vi "BIMS_Collector (SPR).vi"() -> ()   [LabVIEW 2015]
doc: "This program is currently beta software. It is designed to address the data requirements defined primarily by the DHB Ballistic Test Report.\n\nThe general operation of this program is based on the Ballistics Version 2005 application developed internally by DuPont as a research tool for the Spruance Plant Ballistics Lab in Richmond, VA.\n\nPlease note that the original trigger control logic was modified and no longer depends on a safety interlock system to enable operation of a ballistic test.\n\nDuPont makes no warranties and assumes no liabilities in connection with any use of this program."
uses:
  DataSource.ctl
  shotsArr.ctl
  Shot Record.ctl
  Collector State.ctl
  <vilib>/Utility/error.llb/DialogType.ctl
  <vilib>/registry/registry.llb/Registry RtKey.ctl
  <vilib>/DAQmx/read.llb/DAQmx Read (Counter DBL 1Chan 1Samp).vi
  BIMS_Collector Globals.vi
  <vilib>/Utility/config.llb/Write Key (String).vi
  <vilib>/addons/database/Connection.llb/DB Tools Open Connec (Path).vi
  <vilib>/addons/database/Connection.llb/Conn Execute.vi
  <vilib>/addons/database/Recordset.llb/Rec Destroy - Connection.vi
  <vilib>/DAQmx/miscellaneous.llb/DAQmx Fill In Error Info.vi
  <vilib>/addons/database/NI_Database_API.lvlib
  <vilib>/Utility/config.llb/NI_LVConfig.lvlib
  <vilib>/Utility/file.llb/Write To Spreadsheet File (string).vi
panel:
  in  "diagPageVisible":bool
  in  "runtimeMenusVisible":bool=TRUE
  out "loadStatus":string
  out "Loading":u16(ring)
  in  "RESET All":bool
  out "ConfigName":string
  out "TimeNow":string
  in  "EXIT":bool
  in  "mainTabCntrl":enum32{"Setup", "Measure", "History", "System"}(tab)=enum."System"
  in  "SampleEntryTabCntrl":enum32{"Environment", "Sample"}(tab)
  in  "ThreatDetails":u16(ring) caption="Detail"
  in  "ThreatGroups":u16(ring) caption="Group" items=["", "RCC", "FSP", "44 Magnum", "40 S&W", "9mm Luger", "357 Magnum", "357 Sig", "5.56 NATO / 223", "7.62 Win"]
  in  "PowderTypes":u16(ring) caption="Type" items=["", "ACCURATE, NO.2", "ACCURATE, NO.9", "Alliant Herc. Bullseye", "Alliant 2400", "Hercules", "Hi-Skor 700x", "Hi-Skor 800x", "IMR-4198", "IMR-4756", "IMR-4895", "Power Pistol", "Winchester Ball", "WINCHESTER-231", "WINCHESTER-296", "OTHER"]
  in  "Ballisticians":u16(ring) caption="Ballistician" items=["", "Luke Jeter", "Eric Key", "Luke Jeter - Eric Key"]
  in  "Recorders":u16(ring) caption="Recorder"
  in  "Shooters":u16(ring) caption="Shooter"
  in  "Methods":u16(ring) caption="Method" items=["", "V50", "NIJ", "V0", "Custom"]
  in  "RoomT":sgl caption="Temperature (° F)" format="%.1f"
  in  "RoomHum":sgl caption="Humidity (%)" min=0 max=100 format="%.1f"
  in  "SampleBackings":u16(ring)=3 caption="Type" items=["", "Clay", "Aluminum", "Air"]
  in  "clayCalArray":i16[](array[numeric])=[0, 0, 0, 0, 0] caption="Calibration (mm)" min=0 max=99 format="%02.0f"
  out "clayAverage":sgl caption="Clay Average (mm)" format="%#.1f"
  in  "clayTemp":sgl caption="Clay Temp (° F)" format="%.1f"
  out "threatDetails":T1 caption="Description"
  in  "SampleClamping":u16(ring) caption="Clamping" items=["", "None", "12 x 12", "12 x 15", "15 x 15 Flat", "15 x 15 Teeth", "16 x 16 Flat", "16 x 16 Teeth", "18 x 18", "20 x 20", "Hydro Pneumatic"]
  in  "Sample SubTabCntrl":T2(tab)
  in  "SampleID":string caption="Sample ID"
  in  "SampleDimensions":u16(ring) caption="Dimensions" items=["", "15 x 15", "12 x 12", "10.25 x 11.75", "15 x 16", "26 x 26", "8.5 x 11", "12 x 15", "16 x 16", "18 x 18", "20 x 16", "15 x 18", "24 x 24", "13 x 13", "7.5 x 7.5", "VEST PANEL", "CHEST PLATE", "HELMET", "NOT APPLICABLE", "ACH", "PASGT"]
  in  "ModelMfrs":u16(ring) caption="Manufacturer" items=["DuPont Experimental", "Clark Schwebel", "Industriales Textiles", "Maydown", "Second Chance Body Armor", "Point Blank-Marine Interceptor", "Safari Land", "American Body Armor", "Europe", "Force One", "Textile Filter", "Hexcel Schwebel", "BGF", "M.C. GILL", "COLUMBIA", "Britax HEATH TECN", "ARLON", "TEX TECH INC.", "TELAIR", "CADDIN BODY ARMOR", "GEPCO", "3 TEX", "PACA BODY ARMOR", "VON ROL ISOLA", "SIOUX MANUFACTURING", "APEJ-TAIWAN", "FLOPPY BODY ARMOR", "UNICOR", "n/a", "Point Blank", "Diamond Back", "Other"]
  in  "SampleTypes":u16(ring) caption="Sample Type" items=["", "Fabric", "Hard", "Helmet", "Vest", "Paper"]
  in  "Submitters":u16(ring) caption="Submitter" items=["", "Aldo Tavarez", "James Singletary", "Jeff Hanks", "Karl Chang", "Minshon Chiou", "Ron Egres", "Bryce VanArsdalen", "Kevin Mulcahy", "Dave Reichert", "Leo Carbajal"]
  in  "ProjectID":string caption="Project ID"
  in  "BackLayers":i32 caption="# of Layers" min=0 max=99 step=5
  in  "FrontLayers":i32 caption="# of Layers" min=0 max=99 step=5
  in  "BackLayer":u16(ring) caption="Back Layer" items=["", "n/a", "CORDURA 500d"]
  in  "FrontLayer":u16(ring) caption="Front Layer" items=["", "n/a", "CORDURA 1000d"]
  out "totalNumLayers":i32 caption="Total # of Layers" min=0 max=100 step=5
  out "totalBAW":sgl caption="Total BAW (psf)" format="%.2f"
  in  "LayerTabControl":enum32{"1", "2", "3", "4", "5", "6"}(tab) caption="Inner Layers"
  out "fab1_totalWt":sgl caption="Fab1 Wt" min=0 max=99 step=5 format="%.2f"
  out "SampleAttribs_1":T3 caption="fabricAttribs_1"
  in  "Layer_1":T4 caption="Fabric #1" {"plyNum" min=0 max=99 step=5}
  in  "SampleStyle_1":u16(ring)
  in  "Mfr_1":u16(ring) caption="vendor" items=["", "3M", "A&P Technology", "Absecon Mills", "ABT Sciences", "Aermet", "ArmorStruxx", "Artec", "Axiom", "BAE Advanced Ceramics", "Barrday", "BGF", "Citterio", "Coors-Tek", "DSM", "DuPont", "DuPont (JPS-SUBC)", "FTC", "Gentex", "Gurit", "Hexcel", "Honeywell", "JD Lincoln", "JPS", "JPS-Alexium", "JPS-Apjet", "JPS-DuPont", "JPS-Huntsman", "JPS-Old Hickory", "JPS-TSG", "Kamenskvolokno", "Lincoln Fabrics", "Loctite", "Lord", "LTC", "Marcus Materials", "McMaster-Carr", "Nanocomp", "Neva", "Nolax", "OConnell", "Patriot 3", "PATZ", "PBO", "Polystrand", "Pro-Systems", "ProTech", "Rusar", "Saati", "Saint Gobain", "S-Bond", "SEAL", "Sioux", "SPDW", "TechFiber", "Teijin", "Tencate", "Tensylon", "TexTech", "Toray", "TWARON", "UNKNOWN", "VonWeiss", "Xymid", "Z11"]
  in  "layerStitch_1":u16(ring) caption="Stitch" items=["", "1-inch quilt", "2-inch quilt", "Corner Bartack", "Corners", "Custom (Panel)", "Custom (Vest)", "Diamond", "Edge", "n/a", "Normal"]
  out "fab2_totalWt":sgl caption="Fab2 Wt" min=0 max=99 step=5 format="%.2f"
  out "SampleAttribs_2":T3 caption="fabricAttribs_2"
  in  "Layer_2":T4 caption="Fabric #2" {"plyNum" min=0 max=99 step=5}
  in  "SampleStyle_2":u16(ring)
  in  "Mfr_2":u16(ring) caption="vendor" items=["", "3M", "A&P Technology", "Absecon Mills", "ABT Sciences", "Aermet", "ArmorStruxx", "Artec", "Axiom", "BAE Advanced Ceramics", "Barrday", "BGF", "Citterio", "Coors-Tek", "DSM", "DuPont", "DuPont (JPS-SUBC)", "FTC", "Gentex", "Gurit", "Hexcel", "Honeywell", "JD Lincoln", "JPS", "JPS-Alexium", "JPS-Apjet", "JPS-DuPont", "JPS-Huntsman", "JPS-Old Hickory", "JPS-TSG", "Kamenskvolokno", "Lincoln Fabrics", "Loctite", "Lord", "LTC", "Marcus Materials", "McMaster-Carr", "Nanocomp", "Neva", "Nolax", "OConnell", "Patriot 3", "PATZ", "PBO", "Polystrand", "Pro-Systems", "ProTech", "Rusar", "Saati", "Saint Gobain", "S-Bond", "SEAL", "Sioux", "SPDW", "TechFiber", "Teijin", "Tencate", "Tensylon", "TexTech", "Toray", "TWARON", "UNKNOWN", "VonWeiss", "Xymid", "Z11"]
  in  "layerStitch_2":u16(ring) caption="Stitch" items=["", "1-inch quilt", "2-inch quilt", "Corner Bartack", "Corners", "Custom (Panel)", "Custom (Vest)", "Diamond", "Edge", "n/a", "Normal"]
  out "fab3_totalWt":sgl caption="Fab3 Wt" min=0 max=99 step=5 format="%.2f"
  out "SampleAttribs_3":T3 caption="fabricAttribs_3"
  in  "Layer_3":T4 caption="Fabric #3" {"plyNum" min=0 max=99 step=5}
  in  "SampleStyle_3":u16(ring)
  in  "Mfr_3":u16(ring) caption="vendor" items=["", "3M", "A&P Technology", "Absecon Mills", "ABT Sciences", "Aermet", "ArmorStruxx", "Artec", "Axiom", "BAE Advanced Ceramics", "Barrday", "BGF", "Citterio", "Coors-Tek", "DSM", "DuPont", "DuPont (JPS-SUBC)", "FTC", "Gentex", "Gurit", "Hexcel", "Honeywell", "JD Lincoln", "JPS", "JPS-Alexium", "JPS-Apjet", "JPS-DuPont", "JPS-Huntsman", "JPS-Old Hickory", "JPS-TSG", "Kamenskvolokno", "Lincoln Fabrics", "Loctite", "Lord", "LTC", "Marcus Materials", "McMaster-Carr", "Nanocomp", "Neva", "Nolax", "OConnell", "Patriot 3", "PATZ", "PBO", "Polystrand", "Pro-Systems", "ProTech", "Rusar", "Saati", "Saint Gobain", "S-Bond", "SEAL", "Sioux", "SPDW", "TechFiber", "Teijin", "Tencate", "Tensylon", "TexTech", "Toray", "TWARON", "UNKNOWN", "VonWeiss", "Xymid", "Z11"]
  in  "layerStitch_3":u16(ring) caption="Stitch" items=["", "1-inch quilt", "2-inch quilt", "Corner Bartack", "Corners", "Custom (Panel)", "Custom (Vest)", "Diamond", "Edge", "n/a", "Normal"]
  out "fab4_totalWt":sgl caption="Fab4 Wt" min=0 max=99 step=5 format="%.2f"
  out "SampleAttribs_4":T3 caption="fabricAttribs_4"
  in  "Layer_4":T4 caption="Fabric #4" {"plyNum" min=0 max=99 step=5}
  in  "SampleStyle_4":u16(ring)
  in  "Mfr_4":u16(ring) caption="vendor" items=["", "3M", "A&P Technology", "Absecon Mills", "ABT Sciences", "Aermet", "ArmorStruxx", "Artec", "Axiom", "BAE Advanced Ceramics", "Barrday", "BGF", "Citterio", "Coors-Tek", "DSM", "DuPont", "DuPont (JPS-SUBC)", "FTC", "Gentex", "Gurit", "Hexcel", "Honeywell", "JD Lincoln", "JPS", "JPS-Alexium", "JPS-Apjet", "JPS-DuPont", "JPS-Huntsman", "JPS-Old Hickory", "JPS-TSG", "Kamenskvolokno", "Lincoln Fabrics", "Loctite", "Lord", "LTC", "Marcus Materials", "McMaster-Carr", "Nanocomp", "Neva", "Nolax", "OConnell", "Patriot 3", "PATZ", "PBO", "Polystrand", "Pro-Systems", "ProTech", "Rusar", "Saati", "Saint Gobain", "S-Bond", "SEAL", "Sioux", "SPDW", "TechFiber", "Teijin", "Tencate", "Tensylon", "TexTech", "Toray", "TWARON", "UNKNOWN", "VonWeiss", "Xymid", "Z11"]
  in  "layerStitch_4":u16(ring) caption="Stitch" items=["", "1-inch quilt", "2-inch quilt", "Corner Bartack", "Corners", "Custom (Panel)", "Custom (Vest)", "Diamond", "Edge", "n/a", "Normal"]
  out "fab5_totalWt":sgl caption="Fab5 Wt" min=0 max=99 step=5 format="%.2f"
  out "SampleAttribs_5":T3 caption="fabricAttribs_5"
  in  "Layer_5":T4 caption="Fabric #5" {"plyNum" min=0 max=99 step=5}
  in  "SampleStyle_5":u16(ring)
  in  "Mfr_5":u16(ring) caption="vendor" items=["", "3M", "A&P Technology", "Absecon Mills", "ABT Sciences", "Aermet", "ArmorStruxx", "Artec", "Axiom", "BAE Advanced Ceramics", "Barrday", "BGF", "Citterio", "Coors-Tek", "DSM", "DuPont", "DuPont (JPS-SUBC)", "FTC", "Gentex", "Gurit", "Hexcel", "Honeywell", "JD Lincoln", "JPS", "JPS-Alexium", "JPS-Apjet", "JPS-DuPont", "JPS-Huntsman", "JPS-Old Hickory", "JPS-TSG", "Kamenskvolokno", "Lincoln Fabrics", "Loctite", "Lord", "LTC", "Marcus Materials", "McMaster-Carr", "Nanocomp", "Neva", "Nolax", "OConnell", "Patriot 3", "PATZ", "PBO", "Polystrand", "Pro-Systems", "ProTech", "Rusar", "Saati", "Saint Gobain", "S-Bond", "SEAL", "Sioux", "SPDW", "TechFiber", "Teijin", "Tencate", "Tensylon", "TexTech", "Toray", "TWARON", "UNKNOWN", "VonWeiss", "Xymid", "Z11"]
  in  "layerStitch_5":u16(ring) caption="Stitch" items=["", "1-inch quilt", "2-inch quilt", "Corner Bartack", "Corners", "Custom (Panel)", "Custom (Vest)", "Diamond", "Edge", "n/a", "Normal"]
  out "fab6_totalWt":sgl caption="Fab6 Wt" min=0 max=99 step=5 format="%.2f"
  out "SampleAttribs_6":T3 caption="fabricAttribs_6"
  in  "Layer_6":T4 caption="Fabric #6" {"plyNum" min=0 max=99 step=5}
  in  "SampleStyle_6":u16(ring)
  in  "Mfr_6":u16(ring) caption="vendor" items=["", "3M", "A&P Technology", "Absecon Mills", "ABT Sciences", "Aermet", "ArmorStruxx", "Artec", "Axiom", "BAE Advanced Ceramics", "Barrday", "BGF", "Citterio", "Coors-Tek", "DSM", "DuPont", "DuPont (JPS-SUBC)", "FTC", "Gentex", "Gurit", "Hexcel", "Honeywell", "JD Lincoln", "JPS", "JPS-Alexium", "JPS-Apjet", "JPS-DuPont", "JPS-Huntsman", "JPS-Old Hickory", "JPS-TSG", "Kamenskvolokno", "Lincoln Fabrics", "Loctite", "Lord", "LTC", "Marcus Materials", "McMaster-Carr", "Nanocomp", "Neva", "Nolax", "OConnell", "Patriot 3", "PATZ", "PBO", "Polystrand", "Pro-Systems", "ProTech", "Rusar", "Saati", "Saint Gobain", "S-Bond", "SEAL", "Sioux", "SPDW", "TechFiber", "Teijin", "Tencate", "Tensylon", "TexTech", "Toray", "TWARON", "UNKNOWN", "VonWeiss", "Xymid", "Z11"]
  in  "layerStitch_6":u16(ring) caption="Stitch" items=["", "1-inch quilt", "2-inch quilt", "Corner Bartack", "Corners", "Custom (Panel)", "Custom (Vest)", "Diamond", "Edge", "n/a", "Normal"]
  in  "SampleCoverings":u16(ring) caption="Sample Covering" items=["None", "RipStop", "Plastic bag", "Other"]
  in  "Assemblers":u16(ring) caption="Technician" items=["", "Steve Fox", "Ron Egres", "Patti Whitlow", "Tom Boyer", "Patti Whitlow - Steve Fox"]
  in  "Thickness":dbl caption="Thickness (in)" format="%.3f"
  in  "totalSampleWt":sgl caption="Total Weight (lbs)" format="%.3f"
  in  "Comments":string caption="Remarks (optional):"
  in  "TestConditions":u16(ring) caption="Sample Condition" items=["", "Dry", "Wet", "Hot 160 DEG. F", "Cold", "Weapon Lubricant", "Motor Oil", "Conditioned", "Accelerated Aging"]
  in  "shotsTabCntrl":T5(tab)
  out "cntDn":i32
  in  "Frag Rod":sgl format="%.1f"
  in  "Drag Corrected":bool=TRUE
  out "Impact/speed":sgl caption="Chronograph 1" min=0 max=10000 step=0.1 format="%.1f"
  out "residual/speed":sgl caption="Residual" min=0 max=10000 step=0.1 format="%.1f"
  in  "MeasVelScrnSet1":sgl caption="Set #1" min=0 max=10000 step=0.1 format="%.1f"
  in  "Current/shotstatus":u16(ring) caption="Penetration" items=["Partial", "Complete"]
  in  "Current/residual/speed":sgl caption="Residual Set" min=0 max=10000 step=0.1 format="%.1f"
  in  "shotTimestamp":string caption="Date/Time"
  in  "MeasVelScrnSet2":sgl caption="Set #2" min=0 max=1000000 step=0.1 format="%.1f"
  out "%_Difference":sgl caption="% Vel Diff" format="%.3f"
  in  "backdepth":sgl caption="BF Depth"
  out "Redundant/speed":sgl caption="Chronograph 2" min=0 max=10000 step=0.1 format="%.1f"
  out "Current/avg/speed":sgl caption="Average" min=0 max=1000000 step=0.1 format="%.1f"
  out "Avg/speed":sgl caption="Average" min=0 max=10000 step=0.1 format="%.1f"
  out "DC_ factor":sgl=1.0 caption="DC Factor" format="%.4f"
  in  "Barrel Temp":sgl format="%.1f"
  in  "Shot Description":string caption="Description (optional)"
  in  "Powder Loading":sgl caption="Powder Load" min=0 max=100 step=0.1 format="%.3f"
  in  "Shot Angle":u16 max=90 step=1
  out "Projectile Mass":sgl caption="Projectile Mass (grains)" min=0 step=1
  in  "N.I.J":u16(ring) items=["n/a", "PASS", "FAIL"]
  in  "addShot":bool caption="RANGE SETUP must be selected before shots can be added."
  in  "loadingUnits":enum32{"grams", "grains"}(radio)
  out "instruct_addShot":string="RANGE SETUP and THREAT must be selected before shots can be added."
  out "Set#1 Separation":sgl=4.0 caption="Outer" format="%.2f"
  out "Set#2 Separation":sgl=4.0 caption="Inner" format="%.2f"
  out "ARMED":bool caption="Armed"
  out "saveReq":string="Number of layers in sample ply specification and number of shots in shots table must be greater than 0 to enable saving."
  in  "VsVr Report":bool caption="Report"
  out "Table of Shots":string[][](table) caption="Shot Table"
  in  "MC Listbox of Shots":i32(listbox)
  in  "saveShots":bool
  in  "clearShots":bool
  out "highPartial":i32 caption="High Partial" min=0 max=10000 step=1
  out "lowComplete":i32 caption="Low Complete" min=0 max=10000 step=1
  out "rangeOfResults":i32 caption="Range of Results" min=0 max=10000 step=1
  out "zmr 2":sgl caption="ZMR" format="%.1f"
  out "computed_V50":sgl caption="V50" format="%.1f"
  out "Pairs":i16 min=0 max=100 step=1
  in  "reportV50":bool caption="Report"
  in  "maxDev":sgl=125.0 caption="Max Deviation" min=0 max=300 step=25
  in  "undoLastShot":bool
  in  "deleteShot":bool
  in  "nextShot":bool
  in  "shotsArr":T6 {"Frag Rod" format="%.1f"; "UncorrectedAvgVel_PB" format="%.1f"; "UncorrectedRed_PB" format="%.1f"; "strikeVel_PB" format="%.1f"; "velLoss_PB" format="%.1f"; "avgVel_PB" format="%.1f"; "Redundant_Velocity" format="%.1f"; "Energy Loss (J)" format="%.3e"; "Projectile Mass" min=0 step=1 format="%.4f"; "Corrected residual" format="%.2f"; "Uncorrected Residual" format="%.1f"; "Corrected Impact" format="%.2f"; "Uncorrected Impact" format="%.1f"; "Shot Angle" max=90 step=1; "SHOT STATUS" items=["Partial", "Complete"]; "IMPACT VELOCITY" min=0 max=10000 step=0.1 format="%.1f"; "Barrel Temperature" format="%.1f"; "Powder Loading" format="%.4f"; "RESIDUAL  VELOCITY" min=0 max=10000 step=0.1 format="%.1f"}
  out "velProfile":cluster{dbl, dbl}[](graph) caption="Shot Velocity Measurement Profile"
  out "velCompProf":cluster{"vStrike":dbl, "vA":dbl} caption="Velocity in fps\n(computed)"
  out "velMeasProf":T8 caption="Velocity in fps\n(measured)"
  out "relativeTime":cluster{"ts2":dbl, "ts3":dbl, "ts1":dbl} caption="Relative time\n(microsec)"
  out "displacement":T9={"ds_v2"=6.75, "ds2"=5.0833, "ds_vB"=4.9167, "ds3"=4.75, "ds_vAvg"=6.9167, "ds_v1"=7.0833, "ds1"=8.75, "ds_vA"=8.9167, "ds0"=9.0833} caption="Distance from\ntarget (ft)" {"ds0" format="%_4g"; "ds_vA" format="%_4g"; "ds1" format="%_4g"; "ds_v1" format="%_4g"; "ds_vAvg" format="%_4g"; "ds3" format="%_4g"; "ds_vB" format="%#_4g"; "ds2" format="%#_4g"; "ds_v2" format="%_4g"}
  out "arrIDC":dbl[](array[numeric]) caption="Instantaneous Drag Coefficient"
  in  "rangeSetup":u16(ring)=1 caption="Range Dimensions" items=["Short (small frag)", "Standard (handgun)", "Long (rifle)"]
  out "mid_to_targ_dist":sgl=5.0 caption="Mid To Target (ft)"
  in  "historyTabCntrl":enum32{"Powder Loading", "Panel Search"}(tab)=enum."Panel Search"
  in  "Threat.freeTxt":string caption="Threat"
  in  "Powder.freeTxt":string caption="Powder"
  in  "QueryLoad":bool
  in  "lkupEndDate":timestamp caption="End Date" format="%<%x>T"
  in  "lkupStartDate":timestamp caption="Begin Date" format="%<%x>T"
  out "Vel.vs.Loading":cluster{dbl[], dbl[]}(graph)
  out "v50_table":string[][](table)
  in  "maxRecs":u16=1001 caption="Max # of SHOT Records" min=1 max=10000 step=100
  out "ActualNumRecs":i32=1001 caption="Actual # Returned"
  in  "ThreatSize_0":u16(ring) caption="Threat Size" items=["", "2", "4", "16", "17", "44", "55", "62", "64", "85", "123", "124", "125", "148", "158", "166", "180", "207", "240"]
  in  "panelSearch":bool
  in  "Mfr_0":u16(ring) caption="Manufacturer" items=["", "3M", "A&P Technology", "Absecon Mills", "ABT Sciences", "Aermet", "ArmorStruxx", "Artec", "Axiom", "BAE Advanced Ceramics", "Barrday", "BGF", "Citterio", "Coors-Tek", "DSM", "DuPont", "DuPont (JPS-SUBC)", "FTC", "Gentex", "Gurit", "Hexcel", "Honeywell", "JD Lincoln", "JPS", "JPS-Alexium", "JPS-Apjet", "JPS-DuPont", "JPS-Huntsman", "JPS-Old Hickory", "JPS-TSG", "Kamenskvolokno", "Lincoln Fabrics", "Loctite", "Lord", "LTC", "Marcus Materials", "McMaster-Carr", "Nanocomp", "Neva", "Nolax", "OConnell", "Patriot 3", "PATZ", "PBO", "Polystrand", "Pro-Systems", "ProTech", "Rusar", "Saati", "Saint Gobain", "S-Bond", "SEAL", "Sioux", "SPDW", "TechFiber", "Teijin", "Tencate", "Tensylon", "TexTech", "Toray", "TWARON", "UNKNOWN", "VonWeiss", "Xymid", "Z11"]
  in  "SampleStyle_0":u16(ring) caption="Sample Style"
  in  "srchParams":T10={"maxPanels"=1001, "lkupPanelStartDate"=timestamp(0 s since 1904-01-01), "lkupPanelEndDate"=timestamp(3376658114.0909824 s since 1904-01-01)} {"lkupPanelEndDate" format="%<%x>T"; "lkupPanelStartDate" format="%<%x>T"; "maxPanels" min=1 max=10000 step=100}
  out "actualNumPanels":i32 caption="Actual # Returned"
  out "pastPanels":string[][](table)
  in  "Record #":i32=1 min=0 max=59980
  in  "reportV50_History":bool
  out "SampleAttribs_0":T11 caption="fabricAttribs_1"
  in  "Requestors_0":u16(ring) caption="Submitter" items=["", "Aldo Tavarez", "Bryce VanArsdalen", "Dave Reichert", "James Singletary", "Jeff Hanks", "Karl Chang", "Kevin Mulcahy", "Leo Carbajal", "Minshon Chiou", "Ron Egres"]
  in  "aboutTabCntrl":enum32{"About ", "Internal Use"}(tab)
  in  "RefreshMetadata":bool
  out "lastShot":i32 caption="Shot"
  out "lastSamp":i32 caption="Sample"
  in  "PublishNewRecords":bool
  in  "internal":enum32{"ctr", "deploy", "misc"}(tab)=enum."misc"
  out "taskCtr1":refnum<k21>
  in  "ctr1":tag="LightScreens/ctr1"
  in  "readyClock":bool caption="Clock"
  in  "ActiveDev":tag="LightScreens"
  in  "ctr0":tag="LightScreens/ctr0"
  in  "SampClk.Timebase.Src":tag="/LightScreens/80MHzTimebase"
  out "Device S/N":string
  in  "MeasSrc":T12=enum."Screens" caption="Source"
  in  "ARM":bool
  out "errCtr0":errorcluster
  out "errCtr1":errorcluster
  out "taskCtr0":refnum<k21>
  in  "Folder":string="esvrs11" caption="Publish Folder"
  in  "useBMC":bool caption="Use Message Center?"
  in  "Server":string="esvrs11"
  in  "Site":string="ICE1"
  in  "InterlockExists":bool=TRUE caption="Safety Interlock Hardware Exist?"
  in  "ScreenSetAvgg":bool=TRUE caption="Average Screen Sets?"
  in  "Sort by AVG":bool=TRUE caption="Sort shots by average velocity"
  in  "useBallisitican":bool=TRUE caption="Use Ballistician field in Setup?"
  in  "useRecorder":bool caption="Use Recorder field in Setup?"
  in  "useShooter":bool caption="Use Shooter field in Setup?"
  in  "close arming loop":bool
  out "progState":T13
  in  "clearErrors":bool
  in  "LayerStitchTypes":u16(ring) caption="Stitch" items=["", "Custom (Vest)", "Corners", "1-inch quilt", "2-inch quilt", "Normal", "Custom (Panel)", "Corner Bartack", "Diamond", "Edge", "n/a"]
  out "GrainSize":u16 caption="Grain"
  out "U/I EvErr":errorcluster
  out "SMErr":errorcluster
  in  "Models":u16(ring) caption="Model #" items=["n/a"]
  in  "serialNum":string caption="Serial #"
  in  "SampleDescrip":u16(ring) caption="Misc. Sample Description (legacy)"
  out "lengthUnits":string="FOOT" caption="Distance Units"
  out "massUnits":string="GRAMS" caption="Weight Units"
  in  "Threat":u16(ring) caption="Threat (long description)"
  in  "Type of work":string="QC"
  in  "minV50":i32=1500 caption="Minimum V50"
  out "configPath":path=path "P:/Private/My Projects/AFS/BIMS/2008/BIMS_Collector.ini" caption="Configuration Path (INI)"
  out "STOP (Shots MC LB)":bool=TRUE
  in  "lookupRec":bool caption="lookup"
  in  "clayCalib":string="##-##-##-##-##" caption="Calibration"
  in  "Fabric Description":string caption="Fabric Desc"
  in  "Areal density text":string
  in  "Areal Density":dbl format="%.2f"
  out "Residual factor":sgl=1.0 caption="Residual" min=0 max=1 format="%.5f"
  out "Impact factor":sgl=1.0 caption="Impact" min=0 max=1 format="%.5f"
  out "Partial":sgl[](array[numeric]) format="%.2f"
  out "factor array":sgl[](array[numeric]) format="%.4f"
  out "Complete":sgl[](array[numeric]) format="%.2f"
  in  "old threat":u16
  out "Z.M.R.":sgl min=0 step=0.1 format="%.1f"
  in  "Residual/Target Dist":sgl=7.083333 format="%.2f"
  out "Residual/Separation":sgl=4.0 format="%.2f"
  in  "Set#1_to_Target":sgl=7.083333 format="%.2f"
  out "Barrel to Screen":sgl=7.8333 format="%.2f"
  out "CorrectedVelScrnSet1":sgl=1503.981 format="%.2f"
  out "Corrected Residual":sgl=751.9905 format="%.2f"
  out "correction coefficient":sgl format="%.8f"
  in  "SoftwareVersion":dbl caption="Version" format="%.2f"
  in  "percent warning":sgl=1.0 format="%.2f"
  out "#_partials":i32
  out "#_completes":i32
  out "conversion factor":sgl=0.3048037 format="%.5f"
  out "CorrectedVelScrnSet2":sgl=1551.8816 caption="Corrected Redundant" format="%.2f"
  out "Corrected Average":sgl=1527.9313 format="%.2f"
  in  "processShots":bool caption="Proc Shots"
  in  "WeaponTypes":u16(ring) caption="Weapon" items=["", "Universal Receiver", "Other"]
  in  "TestStandards":u16(ring)=2 caption="Standard" items=["n/a", "NIJ 0101.04", "MIL-STD-662F"]
  out "SUBMIT DATE/TIME":string
  # "Effectively restarts the application from scratch, as if the user pressed the EXIT button and then restarted the application."
  # "Configured for"
  # "Threat"
  # "*"
  # "*"
  # "Test"
  # "Powder"
  # "*"
  # "Personnel"
  # "Room"
  # "*"
  # "Backing"
  # "*"
  # "*"
  # "*"
  # "Strike Face"
  # "Body Side"
  # "Layer"
  # "Mfr"
  # "Style"
  # "# of Plies"
  # "Lot"
  # "Roll"
  # "Stitch"
  # "Internal ID"
  # "Fiber"
  # "Denier"
  # "Construction"
  # "Weave"
  # "Finish"
  # "Basis weight (oz/yd²)"
  # "Yarn Merge"
  # "Total Weight"
  # "*"
  # "*"
  # "*"
  # "1"
  # "2"
  # "3"
  # "4"
  # "5"
  # "6"
  # "Required"
  # "*"
  # "Shot Parameters"
  # "cm"
  # "deg"
  # "degF"
  # "Screens\nSeparation"
  # "Ft"
  # "Velocity Measurements"
  # "Observations"
  # "Table Functions"
  # "Summary"
  # "Reports"
  # "Test Record"
  # "Edit Shot Records"
  # "Corrected"
  # "Shot #"
  # "t0"
  # "0"
  # "S Strike"
  # "0"
  # "Internal ID#"
  # "Fiber"
  # "Denier"
  # "Pick"
  # "Weave"
  # "Finish"
  # "oz/yd²"
  # "Asset"
  # "DuPont Protection Technologies\nBallistics Information Management System\n\nBIMS\nEnterprise\n\n\nSample Performance\nData Collector\n\nJanuary 2015"
  # "DuET Measurement System Technologies\nDUCOM 8 695-2330 for technical support"
  # "Last Assigned\nRecord Numbers"
  # "Deployment Configuration"
  # "NI LabVIEW 2014 Ver 14.0f1 (32-bit)\nLast build on 12/05/2014"
  # "Correction Factors"
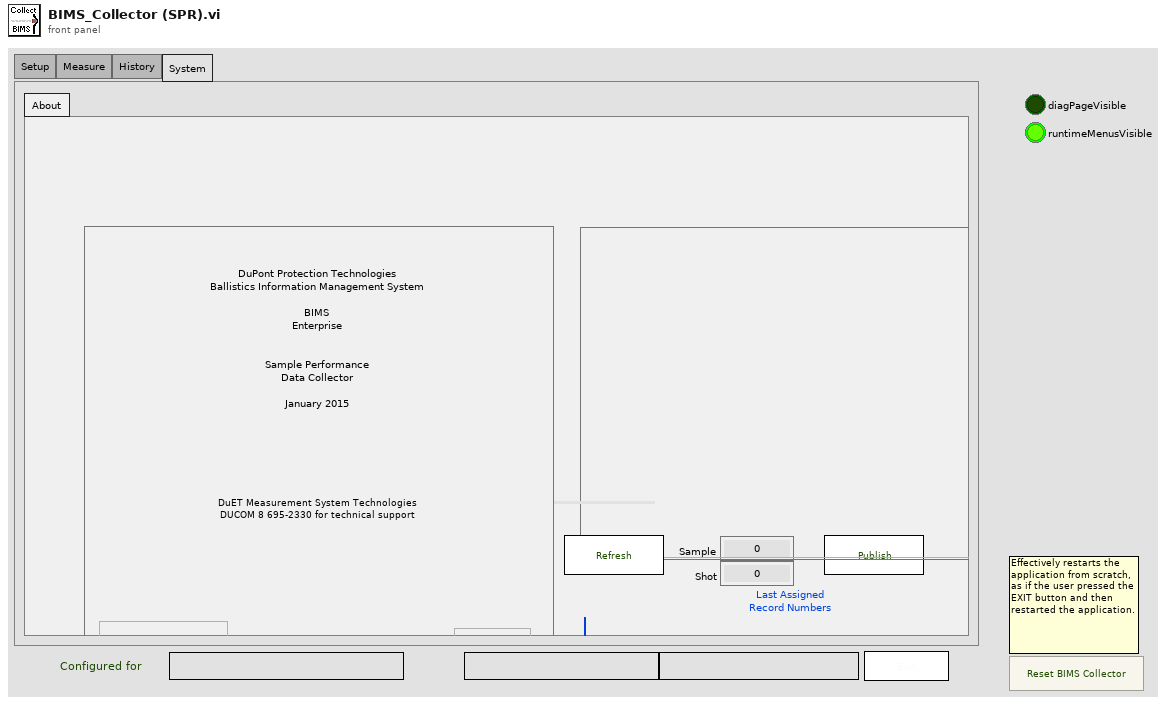
[diagram p1: front panel]
types:
  T1 = cluster{"barrelLength":string, "dragCorrection":string, "detailDescription":string, "barrelCaliber":string, "grainSize":string, "Make":string, "Model":string}
  T2 = enum32{"General Specification", "Ply Specification", "Preparation"}
  T3 = cluster{"Fabric.fiber":string, "Fabric.denier":string, "pick":string, "weave":string, "finish":string, "ozPerYd2":string, "fabricID_DHB":string, "yarnMerge":string}
  T4 = cluster{"plyNum":i32, "LotNum":string, "RollNum":string}
  T5 = enum32{"Ready-Aim-Fire", "Shots Table", "Edit", "Instantaneous DC"}
  T6 = typedef "shotsArr.ctl" = T7[]
  T7 = typedef "Shot Record.ctl" = cluster{"Uncorrected Impact":sgl, "Uncorrected Residual":sgl, "avgVel_PB":sgl, "IMPACT VELOCITY":sgl, "RESIDUAL  VELOCITY ":sgl, "Shot Description":string, "Powder Loading ":sgl, "Barrel Temperature":sgl, "TIME / DATE":string, "shot order":i32, "SHOT STATUS":u16, "Shot Angle":u16, "Corrected Impact":sgl, "Corrected residual":sgl, "Projectile Mass":sgl, "usedv50":bool, "Energy Loss (J)":sgl, "BackFace\nDepth":sgl, "BackFace\nDiameter":sgl, "Redundant_Velocity":sgl, "velLoss_PB":sgl, "strikeVel_PB":sgl, "UncorrectedRed_PB":sgl, "CorrectedRed_PB":sgl, "UncorrectedAvgVel_PB":sgl, "V50userExcl":bool, "Frag Rod":sgl}
  T8 = cluster{"v2":dbl, "vB":dbl, "vOuter":dbl, "v1":dbl, "vA":dbl, "vInner":dbl}
  T9 = cluster{"ds_v2":dbl, "ds2":dbl, "ds_vB":dbl, "ds3":dbl, "ds_vAvg":dbl, "ds_v1":dbl, "ds1":dbl, "ds_vA":dbl, "ds0":dbl}
  T10 = cluster{"maxPanels":u16, "lkupPanelStartDate":timestamp, "lkupPanelEndDate":timestamp}
  T11 = cluster{"Fabric.fiber":string, "Fabric.denier":string, "pick":string, "weave":string, "finish":string, "ozPerYd2":string, "fabricID_DHB":string, "asset":string}
  T12 = typedef "DataSource.ctl" = enum16{"Simulated", "Radar", "Screens"}
  T13 = typedef "Collector State.ctl" = enum16{"POLL", "INITIALIZE", "V50 Report or GET Record", "VsVr Report", "SAVE SHOTS", "ADD SHOT", "CLEAR SHOTS", "NEXT SHOT", "DELETE SHOT", "READY CLOCK", "PROC SHOTS", "CHECK DAQ"}
  T14 = typedef "DialogType.ctl" = u16
  T15 = enum8{"Enabled", "Disabled", "Disabled and Grayed Out"}
  T16 = enum32{"Page Enabled", "Page Disabled", "Page Disabled & Grayed"}
  T17 = enum32{"invalid app kind", "Development System", "Run Time System", "Student Edition", "Embedded LabVIEW", "Evaluation", "Custom"}
  T18 = typedef "LVRowAndColumnTypeDef.ctl" = cluster{"Row":i32, "Column":i32}
  T19 = cluster{"barrelLength":string, "dragCoefficient":string, "detailDescription":string, "barrelCaliber":string, "grainSize":string, "Make":string, "Model":string}
  T20 = cluster{"fiber":string, "denier":string, "construction":string, "weave":string, "finish":string, "ozPerYd2":string, "fabricStyle_DHB":string, "yarnMerge":string}
  T21 = cluster{"fiber":string, "denier":string, "pick":string, "weave":string, "finish":string, "ozPerYd2":string, "internal_ID":string, "asset":string}[]
  T22 = cluster{"plyNum":i32, "LotNum":string, "RollNum":string}[]
  T23 = typedef "NI_LVConfig.lvlib/Config Data RefNum.ctl" = refnum<k1>
  T24 = typedef "Registry RtKey.ctl" = enum32{"HKEY_CLASSES_ROOT", "HKEY_CURRENT_USER", "HKEY_LOCAL_MACHINE", "HKEY_USERS", "HKEY_PERFORMANCE_DATA", "HKEY_CURRENT_CONFIG", "HKEY_DYN_DATA"}
  T25 = cluster{"[0]":string, "[1]":string, "[2]":string, "[3]":string, "[4]":string, "[5]":string, "[6]":string, "[7]":string, "[8]":string, "[9]":string}[]
  T26 = cluster{"[0]":string, "[1]":string, "[2]":string, "[3]":string, "[4]":string, "[5]":string, "[6]":string, "[7]":string, "[8]":string}[]
  T27 = cluster{"Fabric.fiber":string, "Fabric.denier":string, "pick":string, "weave":string, "finish":string, "ozPerYd2":string, "fabricID_DHB":string, "yarnMerge":string}[]
  T28 = cluster{"Uncorrected Impact":bool, "Uncorrected Residual":bool, "avgVel_PB":bool, "IMPACT VELOCITY":bool, "RESIDUAL  VELOCITY ":bool, "Shot Description":bool, "Powder Loading ":bool, "Barrel Temperature":bool, "TIME / DATE":bool, "shot order":bool, "SHOT STATUS":bool, "Shot Angle":bool, "Corrected Impact":bool, "Corrected residual":bool, "Projectile Mass":bool, "usedv50":bool, "Energy Loss (J)":bool, "BackFace\nDepth":bool, "BackFace\nDiameter":bool, "Redundant_Velocity":bool, "velLoss_PB":bool, "strikeVel_PB":bool, "UncorrectedRed_PB":bool, "CorrectedRed_PB":bool, "UncorrectedAvgVel_PB":bool, "V50userExcl":bool, "Frag Rod":bool}
  T29 = cluster{"SampleTypes":refnum<vi>, "SampleDescrip":refnum<vi>}
  T30 = cluster{"max dev":sgl, "residual separation":sgl, "Set#1 Separation":sgl, "Set#2 Separation ":sgl, "impact target dist":sgl, "resid target dist":sgl, "barrel screen dist":sgl, "midpt_to_target_dist":sgl}
  T31 = cluster{"numOfPlies":i32, "LotNum":string, "RollNum":string}[]
  T32 = cluster{string, string, string, string, string, string, string, string, "clayCalib":string, string}
  T33 = cluster{string, string, string, string, string, string, string}
  T34 = cluster{"SampleID":string, "element":string, "Type of work":string, "serialNum":string, "element":string, string, string, string, "element":string, string}
  T35 = cluster{"SampleID":string, "element":string, string, string, string, "element":string}
  T36 = cluster{"[0]":string, "[1]":string, "[2]":string, "[3]":string, "[4]":string, "[5]":string, "[6]":string, "[7]":string, "[8]":string, "[9]":string}
  T37 = cluster{"[0]":string, "[1]":string, "[2]":string, "[3]":string, "[4]":string, "[5]":string, "[6]":string, "[7]":string, "[8]":string}
  T38 = cluster{"element":string, "element":string, "grainSize":string, "element":string, "barrelLength":string, string, "element":string, "element":string, "element":string}
  T39 = cluster{"element":string, "grainSize":string, "element":string, "barrelLength":string, string, "element":string}
  T40 = typedef "NI_Database_API.lvlib/Conn ObjectReference.ctl" = refnum<k1>
  T41 = typedef "NI_Database_API.lvlib/Rec ObjectReference.ctl" = refnum<k1>
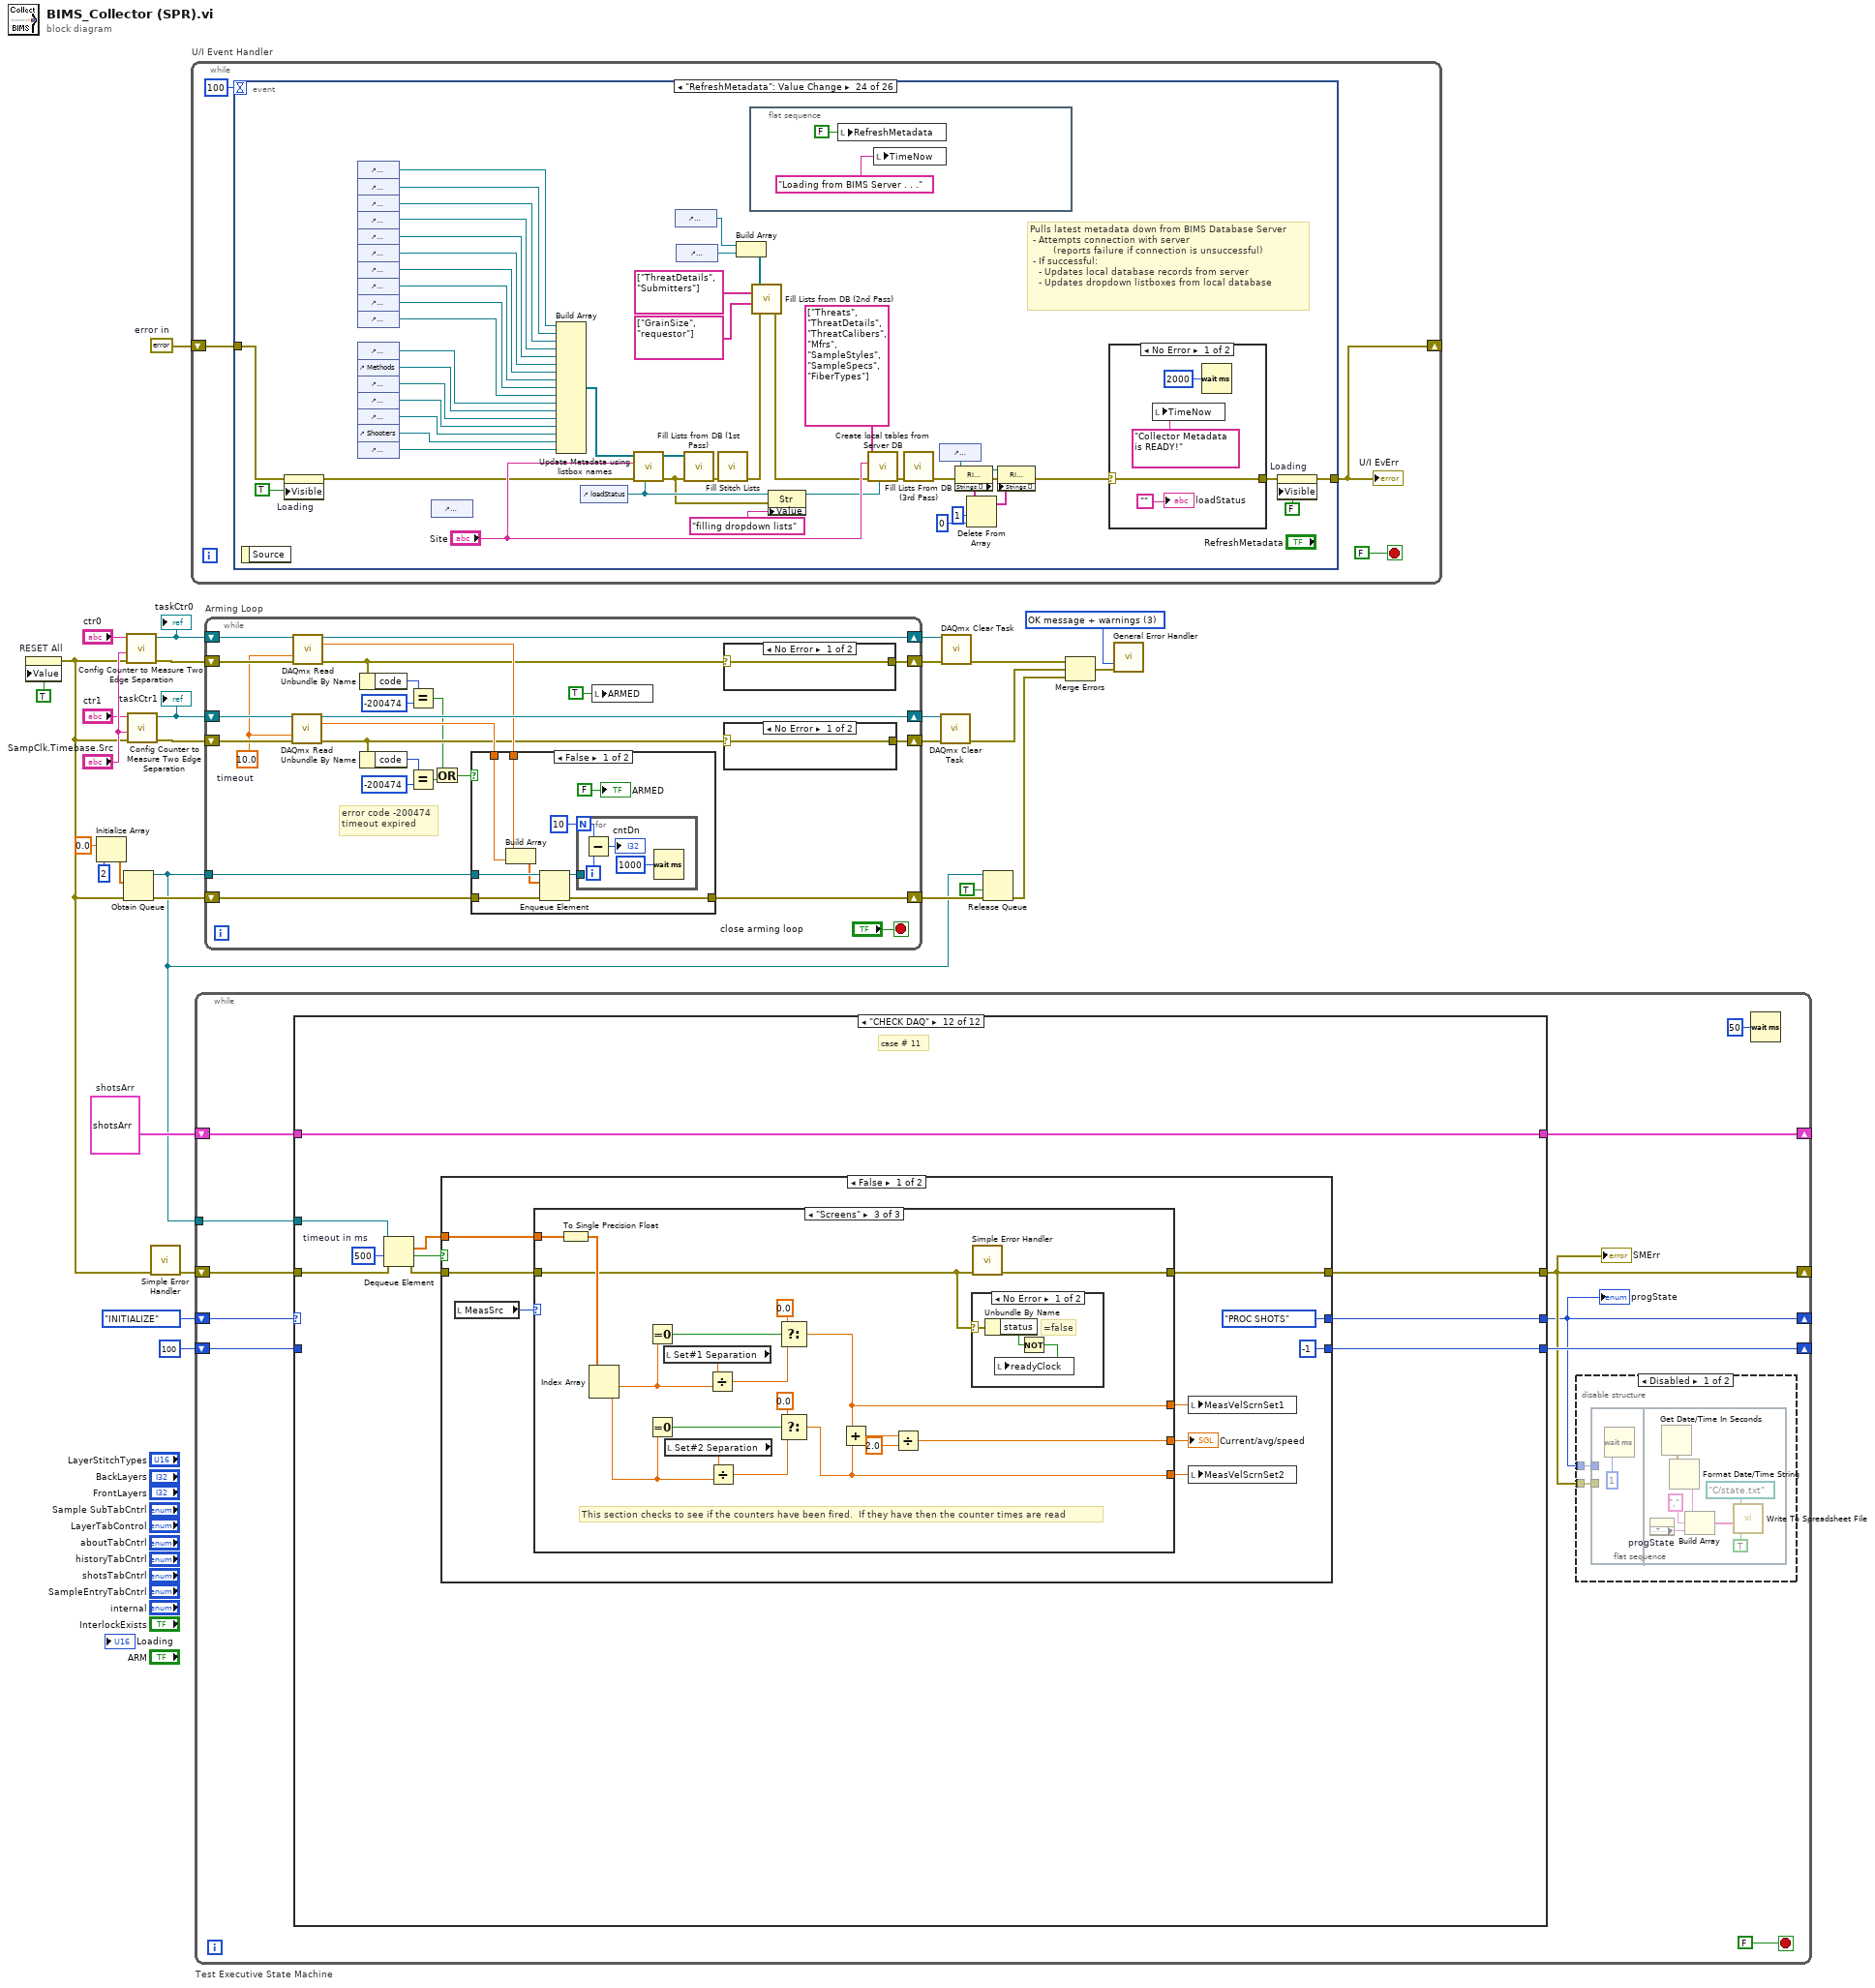
[diagram p0: block diagram]
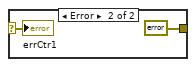
[diagram p3: hidden frame]
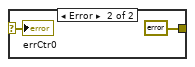
[diagram p4: hidden frame]
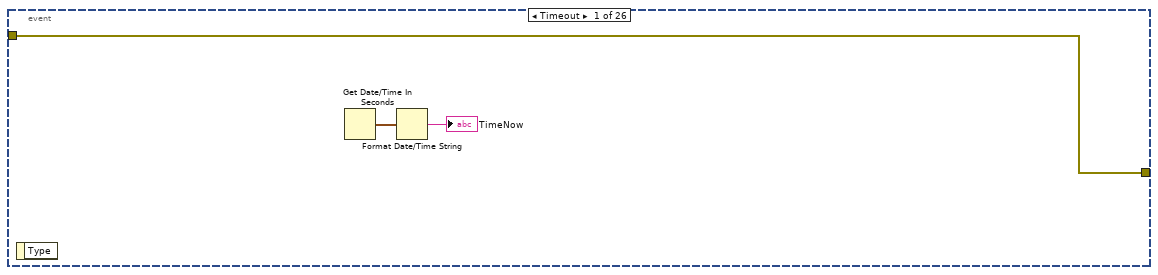
[diagram p5: hidden frame]
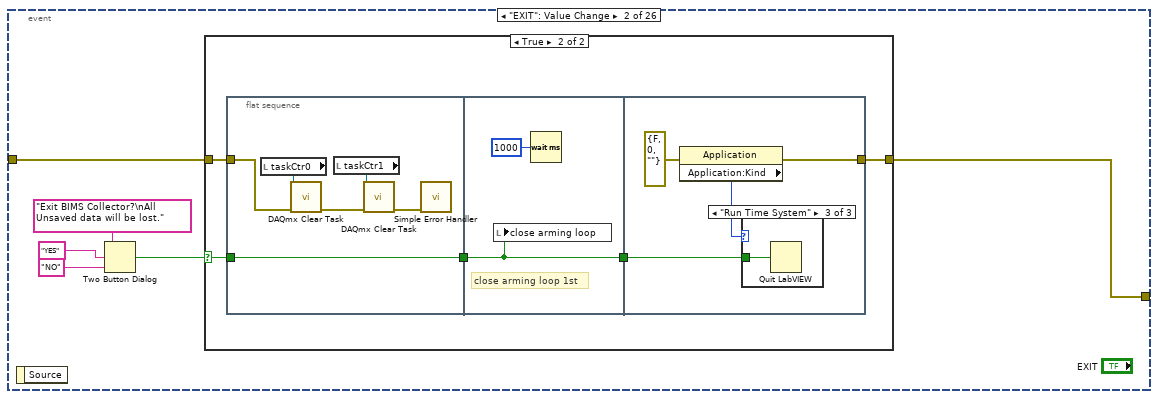
[diagram p6: hidden frame]
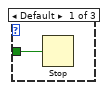
[diagram p8: hidden frame]
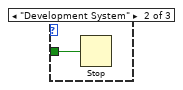
[diagram p9: hidden frame]
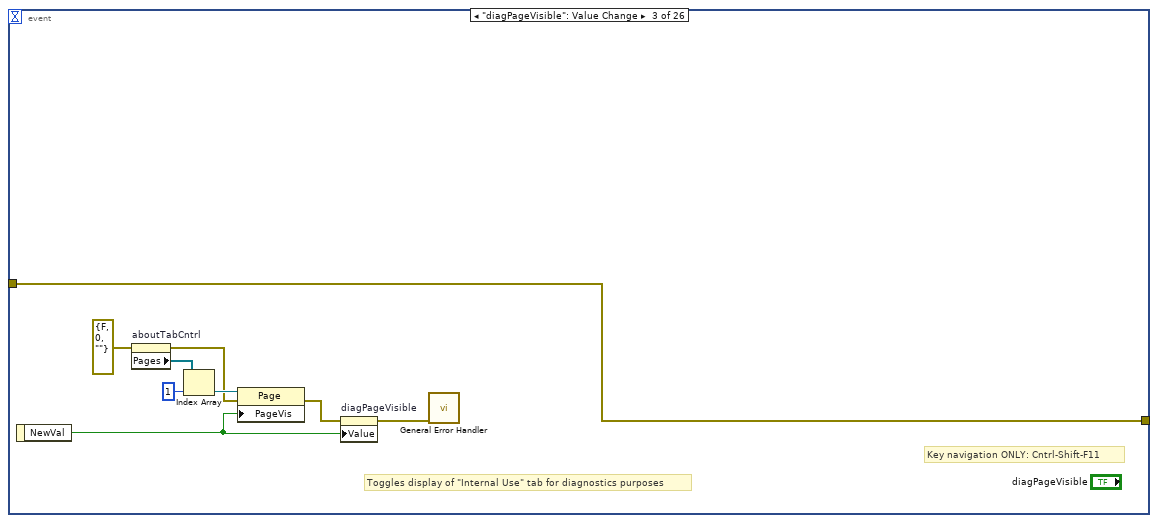
[diagram p10: hidden frame]
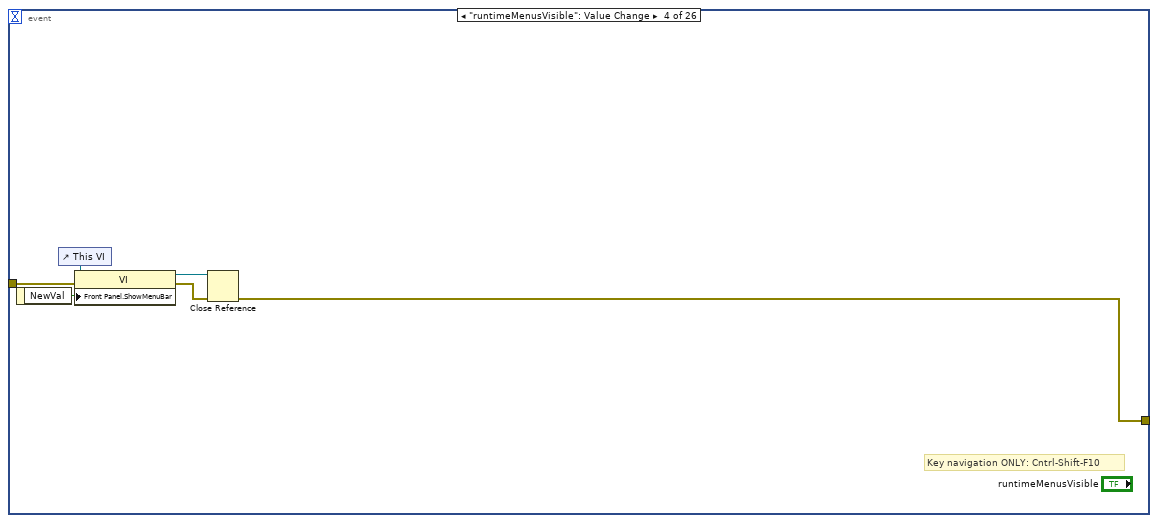
[diagram p11: hidden frame]
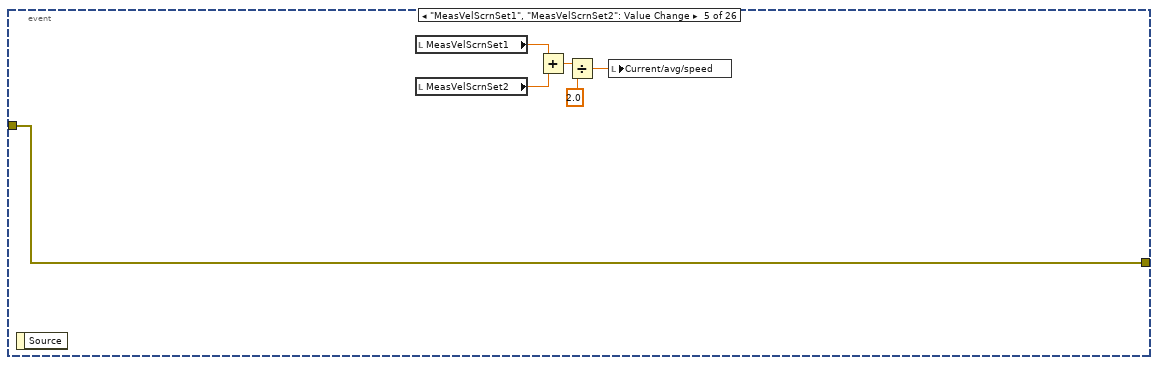
[diagram p12: hidden frame]
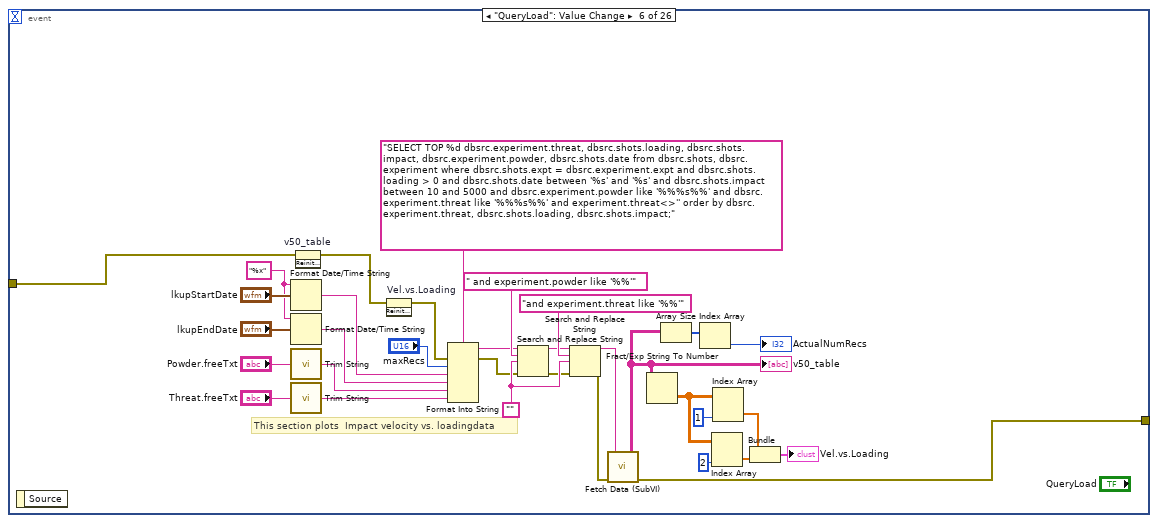
[diagram p13: hidden frame]
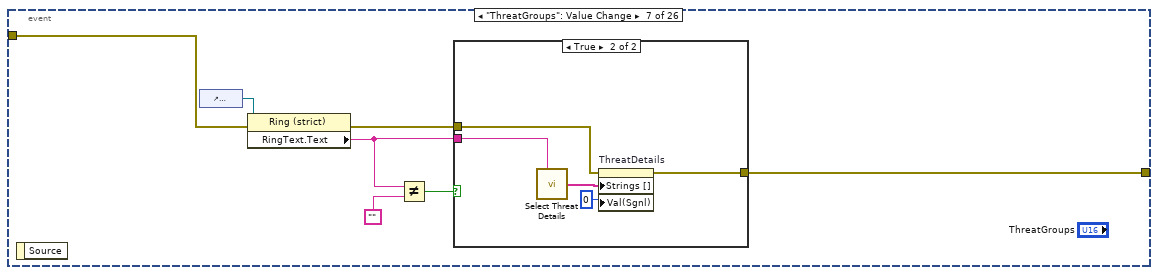
[diagram p14: hidden frame]
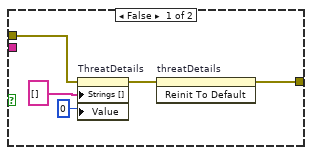
[diagram p15: hidden frame]
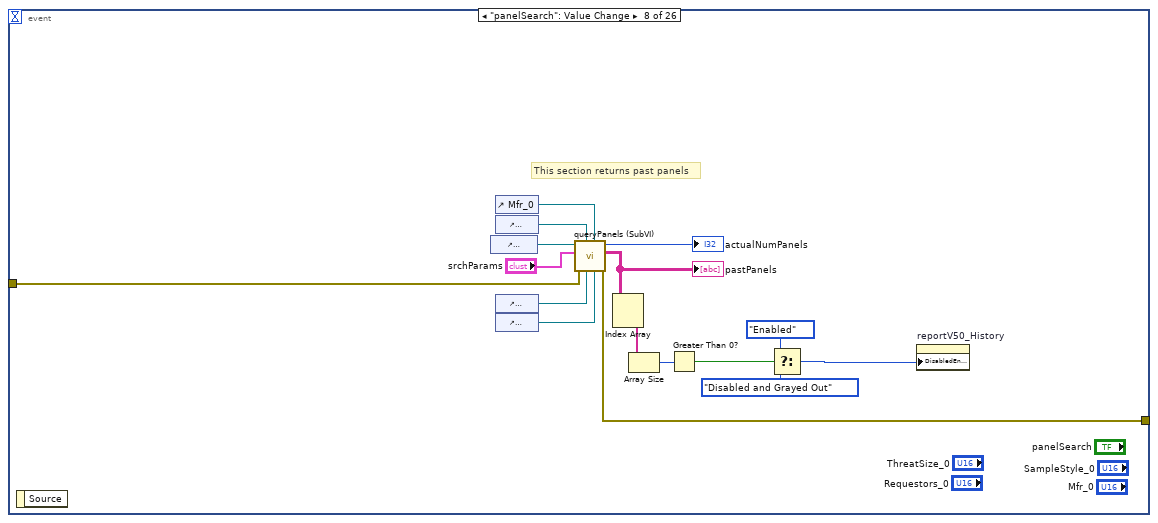
[diagram p16: hidden frame]
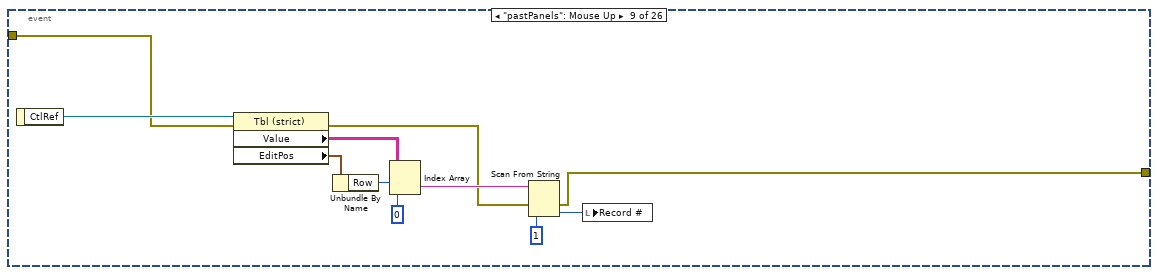
[diagram p17: hidden frame]
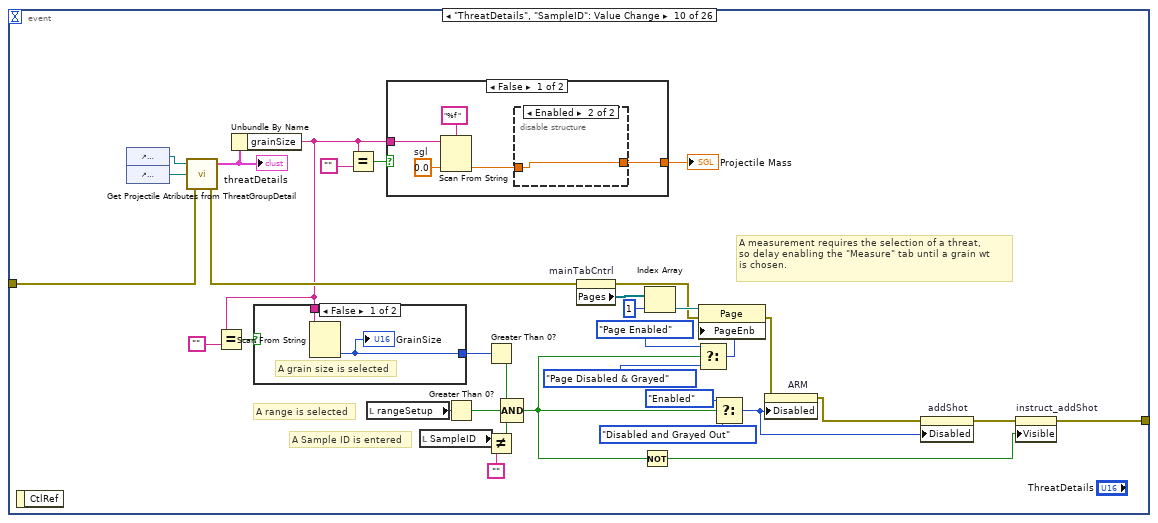
[diagram p18: hidden frame]
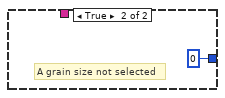
[diagram p19: hidden frame]
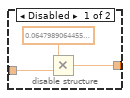
[diagram p20: hidden frame]
diagram:
  w16 = T14 3 items=["no dialog", "OK message", "continue or stop message", "OK message + warnings", "continue/stop + warnings"] ("type of dialog (OK msg:1)")
  w26 = T6 [{"Uncorrected Impact"=0.0, "Uncorrected Residual"=0.0, "avgVel_PB"=0.0, "IMPACT VELOCITY"=0.0, "RESIDUAL  VELOCITY "=0.0, "Shot Description"="", "Powder Loading "=0.0, "Barrel Temperature"=0.0, "TIME / DATE"="", "shot order"=1, "SHOT STATUS"=1, "Shot Angle"=0, "Corrected Impact"=0.0, "Corrected residual"=0.0, "Projectile Mass"=0.0, "usedv50"=FALSE, "Energy Loss (J)"=0.0, "BackFace\nDepth"=0.0, "BackFace\nDiameter"=0.0, "Redundant_Velocity"=0.0, "velLoss_PB"=0.0, "strikeVel_PB"=0.0, "UncorrectedRed_PB"=0.0, "CorrectedRed_PB"=0.0, "UncorrectedAvgVel_PB"=0.0, "V50userExcl"=FALSE, "Frag Rod"=0.0}]  # shotsArr
  w27 = errorcluster {"status"=FALSE, "code"=0, "source"=""}  # error in
  n1 = property on="RESET All" class="Bool (strict)"("Value"=TRUE ("RESET")) -> (error out=w5:errorcluster)  [unwired: 2 in, 1 out]
  n2 = Initialize Array(0.0, 2 ("dimension size")) -> (w6:dbl[])
  n3 = Obtain Queue(element data type=w6, error in (no error)=w5) -> (queue out=w3:refnum<queue>, error out=w21:errorcluster)  [unwired: 3 in, 1 out]
  n4 = call "Config Counter to Measure Two Edge Separation.vi"("errIN"=w5, "SampClk.Timebase.Src"="SampClk.Timebase.Src", "Counter"="ctr0") -> ("errOUT"=w10:errorcluster, "task out"=w2:refnum<k21>)  [unwired: 7 in]
  "taskCtr0" <- w2
  n5 = call "Config Counter to Measure Two Edge Separation.vi"("errIN"=w5, "SampClk.Timebase.Src"="SampClk.Timebase.Src", "Counter"="ctr1") -> ("errOUT"=w9:errorcluster, "task out"=w1:refnum<k21>)  [unwired: 7 in]
  "taskCtr1" <- w1
  n6 = call <vilib>:"Simple Error Handler.vi"("error in (no error)"=w5) -> ("error out"=w22:errorcluster)  [unwired: 4 in, 4 out]
  n7 = while "U/I Event Handler" {
    shift-right: [w31] -> _
    shift-left: w27 -> [w32]
    stop <- FALSE stop-if-true
    n8 = event shown="[23] \"RefreshMetadata\": Value Change" {
      selector: _ -> [_ _ _ _ _ _ _ _ _ _ _ _ _ _ _ _ _ _ _ _ _ _ _ _ _ _]
      dyn-events: _ -> [_ _ _ _ _ _ _ _ _ _ _ _ _ _ _ _ _ _ _ _ _ _ _ _ _ _]
      timeout: 100 -> [_ _ _ _ _ _ _ _ _ _ _ _ _ _ _ _ _ _ _ _ _ _ _ _ _ _]
      tunnel: w32 -> [w35 w38 w67 w77 w85 w87 w124 w148 w154 w180 w217 w259 w297 w299 w335 w371 w374 w383 w410 w416 w442 w459 w461 w493 w524 _]
      tunnel: [w35 w40 w67 w74 w85 w86 w123 w147 w152 w188 w216 w256 w297 w299 w335 w371 w373 w379 w410 w413 w439 w459 w461 w495 w524 w531] -> w31
      event Timeout {
        n9 = event-data() -> ()  [unwired: 2 out]
        n10 = Get Date/Time In Seconds() -> (seconds since 1Jan1904=w37:timestamp)
        n11 = Format Date/Time String(seconds (now)=w37) -> (date/time string=→"TimeNow":string)  [unwired: 2 out]
      }
      event "EXIT": Value Change {
        n12 = event-data() -> ()  [unwired: 2 out]
        n13 = Two Button Dialog(message="Exit BIMS Collector?\nAll Unsaved data will be lost.", 1:"NO" ("F button name (\"Cancel\")"), 2:"YES" ("T button name (\"OK\")")) -> (T button?=w39:bool)
        n14 = case shown="True" w39 {
          selector: w39 -> [_ w48]
          tunnel: [w44 w49] -> w40
          tunnel: w38 -> [w44 w45]
          frame False {
          }
          frame True {
            n15 = flat-sequence {
              tunnel: w48 -> [w55]
              tunnel: [w55] -> w46
              tunnel: w45 -> [w52]
              tunnel: [w57] -> w47
              tunnel: w46 -> [w57]
              tunnel: [w59] -> w49
              tunnel: w47 -> [w58]
              frame #0 {
                n16 = local read "taskCtr0"() -> (w53:refnum<k21>)
                n17 = call <vilib>:"DAQmx Clear Task.vi"("task in"=w53, "error in"=w52) -> ("error out"=w51:errorcluster)  [unwired: 13 in]
                n18 = local read "taskCtr1"() -> (w54:refnum<k21>)
                n19 = call <vilib>:"DAQmx Clear Task.vi"("task in"=w54, "error in"=w51) -> ("error out"=w50:errorcluster)  [unwired: 13 in]
                n20 = call <vilib>:"Simple Error Handler.vi"("error in (no error)"=w50) -> ()  [unwired: 4 in, 5 out]
              }
              frame #1 {
                # "close arming loop 1st"
                n21 = local write "close arming loop"(w57) -> ()
                n22 = Wait (ms)(milliseconds to wait=u32 1000) -> ()  [unwired: 1 out]
              }
              frame #2 {
                n23 = property on="Property Node" class="Application"(error in=errorcluster {"status"=FALSE, "code"=0, "source"=""} ("error in (no error)")) -> (error out=w59:errorcluster, "Application:Kind"=w61:T17)  [unwired: 1 in, 1 out]
                n24 = case shown="\"Run Time System\"" w61 {
                  tunnel: w58 -> [w62 w63 w64]
                  frame Default {
                    n25 = Stop(stop? (T)=w62) -> ()
                  }
                  frame "Development System" {
                    n26 = Stop(stop? (T)=w63) -> ()
                  }
                  frame "Run Time System" {
                    n27 = Quit LabVIEW(quit? (T)=w64) -> ()
                  }
                }
              }
            }
          }
        }
      }
      event "diagPageVisible": Value Change {
        # "Toggles display of \"Internal Use\" tab for diagnostics purposes"
        # "Key navigation ONLY: Cntrl-Shift-F11"
        n28 = event-data() -> ("NewVal"=w70:bool)  [unwired: 1 out]
        n29 = property on="aboutTabCntrl" class="TabCtl (strict)"(error in=errorcluster {"status"=FALSE, "code"=0, "source"=""} ("error in (no error)")) -> (error out=w69:errorcluster, "Pages"=w73:refnum<vi>[])  [unwired: 1 in, 1 out]
        n30 = Index Array(array=w73, index=1) -> (element=w71:refnum<vi>)
        n31 = property on="Property Node" class="Page"(reference=w71, error in=w69, "PageVis"=w70) -> (error out=w68:errorcluster)  [unwired: 1 out]
        n32 = property on="diagPageVisible" class="Bool (strict)"(error in=w68, "Value"=w70) -> (error out=w65:errorcluster)  [unwired: 1 in, 1 out]
        n33 = call <vilib>:"General Error Handler.vi"("error in (no error)"=w65) -> ()  [unwired: 2 in, 13 out]
      }
      event "runtimeMenusVisible": Value Change {
        # "Key navigation ONLY: Cntrl-Shift-F10"
        n34 = event-data() -> ("NewVal"=w79:bool)  [unwired: 1 out]
        n35 = control-ref of="This VI"() -> (w78:refnum<vi>)
        n36 = property class="VI"(reference=w78, error in=w77, "Front Panel.ShowMenuBar"=w79) -> (reference out=w76:refnum<vi>, error out=w75:errorcluster)
        n37 = Close Reference(reference=w76, error in (no error)=w75) -> (error out=w74:errorcluster)
      }
      event "MeasVelScrnSet1", "MeasVelScrnSet2": Value Change {
        n38 = event-data() -> ()  [unwired: 2 out]
        n39 = local read "MeasVelScrnSet1"() -> (w84:sgl)
        n40 = local read "MeasVelScrnSet2"() -> (w83:sgl)
        n41 = Add(x=w84, y=w83) -> (x+y=w82:sgl)
        n42 = Divide(x=w82, y=sgl 2.0) -> (x/y=w80:sgl)
        n43 = local write "Current/avg/speed"(w80) -> ()
      }
      event "QueryLoad": Value Change {
        w92 = "%x" ("time format string (%c)")
        w108 = "" ("replace string (\"\")")
        # "This section plots  Impact velocity vs. loadingdata"
        n44 = event-data() -> ()  [unwired: 2 out]
        n45 = Format Date/Time String(time format string (%c)=w92, seconds (now)="lkupStartDate") -> (date/time string=w91:string)  [unwired: 1 out]
        n46 = Format Date/Time String(time format string (%c)=w92, seconds (now)="lkupEndDate") -> (date/time string=w90:string)  [unwired: 1 out]
        n47 = call "Trim String.vi"("inStr"="Powder.freeTxt") -> ("outStr"=w106:string)
        n48 = call "Trim String.vi"("inStr"="Threat.freeTxt") -> ("outStr"=w107:string)
        n49 = invoke on="v50_table" class="Tbl" method="Reinit To Default"(error in=w87) -> (error out=w99:errorcluster)  [unwired: 2 in, 2 out]
        n50 = invoke on="Vel.vs.Loading" class="WFGraph (strict)" method="Reinit To Default"(error in=w99) -> (error out=w94:errorcluster)  [unwired: 2 in, 2 out]
        n51 = Format Into String(format string="SELECT TOP %d dbsrc.experiment.threat, dbsrc.shots.loading, dbsrc.shots.impact, dbsrc.experiment.powder, dbsrc.shots.date from dbsrc.shots, dbsrc.experiment where dbsrc.shots.expt = dbsrc.experiment.expt and dbsrc.shots.loading > 0 and dbsrc.shots.date between '%s' and '%s' and dbsrc.shots.impact between 10 and 5000 and dbsrc.experiment.powder like '%%%s%%' and dbsrc.experiment.threat like '%%%s%%' and experiment.threat<>'' order by dbsrc.experiment.threat, dbsrc.shots.loading, dbsrc.shots.impact;" ("Format String"), error in=w94, "maxRecs", w91, w90, w106, w107) -> (resulting string=w112:string, error out=w97:errorcluster)  [unwired: 1 in]
        n52 = Search and Replace String(input string=w112, search string=" and experiment.powder like '%%'", replace string=w108, error in=w97) -> (result string=w110:string, error out=w98:errorcluster)  [unwired: 6 out]
        n53 = Search and Replace String(input string=w110, search string="and experiment.threat like '%%'", replace string=w108, error in=w98) -> (result string=w101:string, error out=w96:errorcluster)  [unwired: 6 out]
        n54 = call "Fetch Data (SubVI).vi"("error IN"=w96, "query string"=w101) -> ("error OUT"=w86:errorcluster, "recordset data"=w102:string[][])  [unwired: 4 out]
        "v50_table" <- w102
        n55 = Fract/Exp String To Number(string=w102) -> (number=w116:dbl[][])  [unwired: 4 out]
        n56 = Array Size(array=w102) -> (size(s)=w104:i32[])
        n57 = Index Array(array=w104) -> (element=→"ActualNumRecs":i32)  [unwired: 1 in]
        n58 = Index Array(array=w116, index (col)=2 ("Disabled Index (col)")) -> (element=w115:dbl[])  [unwired: 1 in]
        n59 = Index Array(array=w116, index (col)=1 ("Disabled Index (col)")) -> (element=w114:dbl[])  [unwired: 1 in]
        n60 = Bundle(w114, w115) -> (→"Vel.vs.Loading":cluster{dbl[], dbl[]})  [unwired: 1 out]
      }
      event "ThreatGroups": Value Change {
        n61 = event-data() -> ()  [unwired: 2 out]
        n62 = control-ref of="ThreatGroups"() -> (w125:refnum<vi>)
        n63 = property on="Property Node" class="Ring (strict)"(reference=w125, error in=w124) -> (error out=w122:errorcluster, "RingText.Text"=w120:string)  [unwired: 1 out]
        n64 = Not Equal?(x=w120, y="") -> (x != y?=w119:bool)
        n65 = case shown="True" w119 {
          tunnel: w120 -> [_ w134]
          tunnel: [w126 w132] -> w123
          tunnel: w122 -> [w129 w131]
          frame False {
            n66 = property on="ThreatDetails" class="Ring (strict)"(error in=w129, "Strings []"=string[] [], "Value"=u16 0 ("Value (Signaling)")) -> (error out=w127:errorcluster)  [unwired: 1 in, 1 out]
            n67 = invoke on="threatDetails" class="Clust (strict)" method="Reinit To Default"(error in=w127) -> (error out=w126:errorcluster)  [unwired: 2 in, 2 out]
          }
          frame True {
            n68 = call "Select Threat Details.vi"("threatGroup"=w134) -> ("threatDetails"=w133:string[])  [unwired: 1 out]
            n69 = property on="ThreatDetails" class="Ring (strict)"(error in=w131, "Strings []"=w133, "Val(Sgnl)"=u16 0 ("Value (Signaling)")) -> (error out=w132:errorcluster)  [unwired: 1 in, 1 out]
          }
        }
      }
      event "panelSearch": Value Change {
        # "This section returns past panels"
        n70 = event-data() -> ()  [unwired: 2 out]
        n71 = control-ref of="pastPanels"() -> (w150:refnum<vi>)
        n72 = control-ref of="Mfr_0"() -> (w145:refnum<vi>)
        n73 = control-ref of="SampleStyle_0"() -> (w146:refnum<vi>)
        n74 = control-ref of="Requestors_0"() -> (w144:refnum<vi>)
        n75 = control-ref of="ThreatSize_0"() -> (w143:refnum<vi>)
        n76 = call "queryPanels (SubVI).vi"("ThreatSize_0"=w143, "Mfr_0"=w145, "Requestors_0"=w144, "Style_0"=w146, "error in"=w148, "srchParams"="srchParams", "pastPanels"=w150) -> ("error out"=w147:errorcluster, "recordset data"=w142:string[][], "actualNumPanels"=→"actualNumPanels":i32)  [unwired: 2 in]
        "pastPanels" <- w142
        n77 = Index Array(array=w142) -> (element=w136:string[])  [unwired: 2 in]
        n78 = Array Size(array=w136) -> (size(s)=w141:i32)
        n79 = Greater Than 0?(x=w141) -> (x > 0?=w140:bool)
        n80 = Select(t=T15."Enabled" ("Disabled"), s=w140, f=T15."Disabled and Grayed Out" ("Disabled")) -> (s? t:f=w139:T15)
        n81 = property on="reportV50_History" class="Bool"("DisabledEnum"=w139) -> ()  [unwired: 2 in, 2 out]
      }
      event "pastPanels": Mouse Up {
        n82 = event-data() -> ("CtlRef"=w162:refnum<vi>)  [unwired: 1 out]
        n83 = property on="Property Node" class="Tbl (strict)"(reference=w162, error in=w154) -> (error out=w153:errorcluster, "Value"=w161:string[][], "EditPos"=w160:T18)  [unwired: 1 out]
        n84 = Unbundle By Name(w160) -> ("Row"=w159:i32)
        n85 = Index Array(array=w161, index (row)=w159, index (col)=0 ("disabled index (col)")) -> (element=w158:string)
        n86 = Scan From String(input string=w158, error in=w153, default 1=1 ("Record #")) -> (error out=w152:errorcluster, output 1=w156:i32)  [unwired: 2 in, 2 out]
        n87 = local write "Record #"(w156) -> ()
      }
      event "ThreatDetails", "SampleID": Value Change {
        # "A Sample ID is entered"
        # "A range is selected"
        # "A measurement requires the selection of a threat,\nso delay enabling the \"Measure\" tab until a grain wt\nis chosen."
        n88 = event-data() -> ()  [unwired: 2 out]
        n89 = control-ref of="ThreatGroups"() -> (w181:refnum<vi>)
        n90 = control-ref of="ThreatDetails"() -> (w178:refnum<vi>)
        n91 = call "Get Projectile Atributes from ThreatGroupDetail.vi"("error IN"=w180, "ThreatDetail"=w178, "ThreatGroup"=w181) -> ("error out"=w179:errorcluster, "projectileAttribs"=w177:T19)  [unwired: 1 out]
        "threatDetails" <- w177
        n92 = Unbundle By Name(w177) -> ("grainSize"=w170:string)
        n93 = Equal?(x=w170, y="") -> (x = y?=w171:bool)
        n94 = case shown="False" w171 {
          tunnel: w170 -> [w198 _]
          tunnel: [w197 u16 0 ("GrainSize")] -> w176
          frame False {
            # "A grain size is selected"
            n95 = Scan From String(input string=w198) -> (output 1=w197:u16)  [unwired: 3 in, 4 out]
            "GrainSize" <- w197
          }
          frame True {
            # "A grain size not selected"
          }
        }
        n96 = Equal?(x=w170, y="") -> (x = y?=w195:bool)
        n97 = local read "rangeSetup"() -> (w192:u16)
        n98 = case shown="False" w195 {
          tunnel: [w202 sgl 0.0] -> w191
          tunnel: w170 -> [w200 _]
          frame False {
            w204 = sgl 0.0  # sgl
            n99 = Scan From String(format string="%f " ("Format String"), input string=w200, default 1=w204) -> (output 1=w203:sgl)  [unwired: 2 in, 3 out]
            n100 = disable-structure shown="Enabled" {
              disable-tunnel: w203 -> [w207 w208]
              disable-tunnel: [w206 w208] -> w202
              frame Disabled {
                n101 = Multiply(x=sgl 0.06479891, y=w207) -> (x*y=w206:sgl)
              }
              frame Enabled {
              }
            }
          }
          frame True {
          }
        }
        "Projectile Mass" <- w191
        n102 = local read "SampleID"() -> (w175:string)
        n103 = Greater Than 0?(x=w192) -> (x > 0?=w193:bool)
        n104 = Greater Than 0?(x=w176) -> (x > 0?=w194:bool)
        n105 = Not Equal?(x=w175, y="") -> (x != y?=w173:bool)
        n106 = Compound Arithmetic op=AND(w194, w193, w173) -> (w168:bool)
        n107 = property on="mainTabCntrl" class="TabCtl (strict)"(error in=w179) -> (error out=w184:errorcluster, "Pages"=w187:refnum<vi>[])  [unwired: 1 in, 1 out]
        n108 = Not(x=w168) -> (.not. x?=w183:bool)
        n109 = Index Array(array=w187, index=1) -> (element=w185:refnum<vi>)
        n110 = Select(t=T16."Page Enabled" ("Page Enabled State"), s=w168, f=T16."Page Disabled & Grayed" ("Page Enabled State")) -> (s? t:f=w167:T16)
        n111 = property on="Property Node" class="Page"(reference=w185, error in=w184, "PageEnb"=w167) -> (error out=w182:errorcluster)  [unwired: 1 out]
        n112 = Select(t=T15."Enabled" ("Disabled"), s=w168, f=T15."Disabled and Grayed Out" ("Disabled")) -> (s? t:f=w165:T15)
        n113 = property on="ARM" class="Bool"(error in=w182, "Disabled"=w165) -> (error out=w190:errorcluster)  [unwired: 1 in, 1 out]
        n114 = property on="addShot" class="Bool"(error in=w190, "Disabled"=w165) -> (error out=w189:errorcluster)  [unwired: 1 in, 1 out]
        n115 = property on="instruct_addShot" class="Str"(error in=w189, "Visible"=w183) -> (error out=w188:errorcluster)  [unwired: 1 in, 1 out]
      }
      event "Mfr_1", "Mfr_2", "Mfr_3", "Mfr_4", "Mfr_5", "Mfr_6", "Mfr_0": Value Change {
        n116 = event-data() -> ("CtlRef"=w225:refnum<vi>)  [unwired: 1 out]
        n117 = property on="Property Node" class="Ring (strict)"(reference=w225, error in=w217) -> (error out=w215:errorcluster, "Label.Text"=w221:string, "RingText.Text"=w222:string)  [unwired: 1 out]
        n118 = flat-sequence {
          tunnel: ["Mfr_1"] -> _
          tunnel: ["Mfr_2"] -> _
          tunnel: ["Mfr_3"] -> _
          tunnel: ["Mfr_4"] -> _
          tunnel: ["Mfr_5"] -> _
          tunnel: ["Mfr_6"] -> _
          frame #0 {
          }
        }
        n119 = call "Select Sample Style.vi"("error IN"=w215, "Mfr"=w222) -> ("error Out"=w214:errorcluster, "SampleStyles"=w211:string[])  [unwired: 4 out]
        n120 = Scan From String(format string="Mfr_%d", input string=w221, error in=w214, default 1=0 ("Mfr#")) -> (error out=w212:errorcluster, output 1=w220:i32)  [unwired: 1 in, 2 out]
        n121 = case shown="1" w220 {
          tunnel: [w237 w240 w243 w246 w249 w252 w255] -> w219
          tunnel: [w236 w239 w242 w245 w248 w251 w254] -> w213
          tunnel: w212 -> [w236 w239 w242 w245 w248 w251 w254]
          tunnel: w211 -> [w235 w238 w241 w244 w247 w250 w253]
          tunnel: [w234 w238 w241 w244 w247 w250 w253] -> w210
          frame 0, Default {
            n122 = Delete From Array(array=w235, length=1, index=0) -> (array with subset deleted=w234:string[])  [unwired: 1 out]
            n123 = control-ref of="SampleStyle_0"() -> (w237:refnum<vi>)
          }
          frame 1 {
            n124 = control-ref of="SampleStyle_1"() -> (w240:refnum<vi>)
          }
          frame 2 {
            n125 = control-ref of="SampleStyle_2"() -> (w243:refnum<vi>)
          }
          frame 3 {
            n126 = control-ref of="SampleStyle_3"() -> (w246:refnum<vi>)
          }
          frame 4 {
            n127 = control-ref of="SampleStyle_4"() -> (w249:refnum<vi>)
          }
          frame 5 {
            n128 = control-ref of="SampleStyle_5"() -> (w252:refnum<vi>)
          }
          frame 6 {
            n129 = control-ref of="SampleStyle_6"() -> (w255:refnum<vi>)
          }
        }
        n130 = property on="Property Node" class="Ring (strict)"(reference=w219, error in=w213, "Strings []"=w210, "Val(Sgnl)"=u16 0 ("Value (Signaling)")) -> (error out=w216:errorcluster)  [unwired: 1 out]
      }
      event "SampleStyle_1", "SampleStyle_2", "SampleStyle_3", "SampleStyle_4", "SampleStyle_5", "SampleStyle_6", "SampleStyle_0": Value Change {
        n131 = event-data() -> ("CtlRef"=w265:refnum<vi>)  [unwired: 1 out]
        n132 = call "Get Sample Style Atributes.vi"("StyleNumRef"=w265) -> ("SampleSpecs"=w260:T20)  [unwired: 1 in]
        n133 = flat-sequence {
          tunnel: ["SampleStyle_1"] -> _
          tunnel: ["SampleStyle_2"] -> _
          tunnel: ["SampleStyle_3"] -> _
          tunnel: ["SampleStyle_4"] -> _
          tunnel: ["SampleStyle_5"] -> _
          tunnel: ["SampleStyle_6"] -> _
          frame #0 {
          }
        }
        n134 = property on="Property Node" class="Ring (strict)"(reference=w265, error in=w259) -> (error out=w258:errorcluster, "Label.Text"=w264:string)  [unwired: 1 out]
        n135 = Scan From String(format string="SampleStyle_%d", input string=w264, error in=w258, default 1=0 ("default value 1")) -> (error out=w257:errorcluster, output 1=w262:i32)  [unwired: 1 in, 2 out]
        n136 = case shown="0, Default" w262 {
          tunnel: w260 -> [w274 w277 w280 w283 w286 w289 w292]
          tunnel: w257 -> [w273 w276 w279 w282 w285 w288 w291]
          tunnel: [w272 w275 w278 w281 w284 w287 w290] -> w256
          frame 0, Default {
            n137 = property on="SampleAttribs_0" class="Clust (strict)"(error in=w273, "Val(Sgnl)"=w274) -> (error out=w272:errorcluster)  [unwired: 1 in, 1 out]
            "SampleAttribs_0" <- w274
          }
          frame 1 {
            n138 = property on="SampleAttribs_1" class="Clust (strict)"(error in=w276, "Val(Sgnl)"=w277) -> (error out=w275:errorcluster)  [unwired: 1 in, 1 out]
            "SampleAttribs_1" <- w277
          }
          frame 2 {
            n139 = property on="SampleAttribs_2" class="Clust (strict)"(error in=w279, "Val(Sgnl)"=w280) -> (error out=w278:errorcluster)  [unwired: 1 in, 1 out]
            "SampleAttribs_2" <- w280
          }
          frame 3 {
            n140 = property on="SampleAttribs_3" class="Clust (strict)"(error in=w282, "Val(Sgnl)"=w283) -> (error out=w281:errorcluster)  [unwired: 1 in, 1 out]
            "SampleAttribs_3" <- w283
          }
          frame 4 {
            n141 = property on="SampleAttribs_4" class="Clust (strict)"(error in=w285, "Val(Sgnl)"=w286) -> (error out=w284:errorcluster)  [unwired: 1 in, 1 out]
            "SampleAttribs_4" <- w286
          }
          frame 5 {
            n142 = property on="SampleAttribs_5" class="Clust (strict)"(error in=w288, "Val(Sgnl)"=w289) -> (error out=w287:errorcluster)  [unwired: 1 in, 1 out]
            "SampleAttribs_5" <- w289
          }
          frame 6 {
            n143 = property on="SampleAttribs_6" class="Clust (strict)"(error in=w291, "Val(Sgnl)"=w292) -> (error out=w290:errorcluster)  [unwired: 1 in, 1 out]
            "SampleAttribs_6" <- w292
          }
        }
      }
      event "Sort by AVG": Value Change {
        n144 = event-data() -> ()  [unwired: 2 out]
        n145 = local read "shotsArr"() -> (w295:T6)
        n146 = local read "Site"() -> (w293:string)
        n147 = call "Update Shot Table.vi"("Sort by AVG"="Sort by AVG", "Site"=w293, "shotsArr"=w295) -> ("shotTable OUT"=→"Table of Shots":string[][])
      }
      event "Layer_1.plyNum", "Layer_2.plyNum", "Layer_3.plyNum", "Layer_4.plyNum", "Layer_5.plyNum", "Layer_6.plyNum", "SampleAttribs_1.ozPerYd2", "SampleAttribs_2.ozPerYd2", "SampleAttribs_3.ozPerYd2", "SampleAttribs_4.ozPerYd2", "SampleAttribs_5.ozPerYd2", "SampleAttribs_6.ozPerYd2": Value Change {
        n148 = event-data() -> ()  [unwired: 2 out]
        n149 = global read "BIMS_Collector Globals.vi" "SampleAttribs"() -> (w298:T21)
        n150 = Build Array("Layer_1", "Layer_2", "Layer_3", "Layer_4", "Layer_5", "Layer_6") -> (w300:T22)
        n151 = global write "BIMS_Collector Globals.vi" "LayerSpecs"(w300) -> ()
        n152 = for {
          tunnel: w300 -> [w327] mode=indexing
          shift-right: [w329] -> w308
          shift-left: 0 -> [w328]
          tunnel: [w326] -> w318 mode=indexing
          tunnel: w298 -> [w324] mode=indexing
          n153 = Unbundle By Name(w324) -> ("ozPerYd2"=w320:string)
          n154 = Equal?(x=w320, y="" ("Empty String Constant")) -> (x = y?=w319:bool)
          n155 = case shown="False" w319 {
            tunnel: [w333 sgl 0.0 ("default value 1")] -> w323
            tunnel: w320 -> [w330 _]
            frame False {
              n156 = Scan From String(format string="%f", input string=w330, default 1=sgl 0.0 ("default value 1")) -> (output 1=w333:sgl)  [unwired: 2 in, 3 out]
            }
            frame True {
            }
          }
          n157 = Unbundle By Name(w327) -> ("plyNum"=w325:i32)
          n158 = Add(x=w328, y=w325) -> (x+y=w329:i32)
          n159 = To Single Precision Float(number=w325) -> (single precision float=w322:sgl)
          n160 = Multiply(x=w322, y=w323) -> (x*y=w326:sgl)
        }
        "totalNumLayers" <- w308
        n161 = Divide(x=w318, y=sgl 144.0) -> (x/y=w316:sgl[])
        n162 = Index Array(array=w316) -> (element #1=→"fab1_totalWt":sgl, element #2=→"fab2_totalWt":sgl, element #3=→"fab3_totalWt":sgl, element #4=→"fab4_totalWt":sgl, element #5=→"fab5_totalWt":sgl, element #6=→"fab6_totalWt":sgl)  [unwired: 6 in]
        n163 = Add Array Elements(numeric array=w316) -> (sum=→"totalBAW":sgl)
      }
      event "clayCalArray": Value Change {
        n164 = event-data() -> ()  [unwired: 2 out]
        n165 = for {
          tunnel: "clayCalArray" -> [w361] mode=indexing
          shift-right: [w360] -> w343
          shift-left: "" ("Empty String Constant") -> [w358]
          shift-right: [w355] -> w339
          shift-left: i16[] [] -> [w354]
          n166 = Greater Than 0?(x=w361) -> (x > 0?=w362:bool)
          n167 = case shown="False" w362 {
            tunnel: w361 -> [_ w368]
            tunnel: ["##" ("clayCalib") w370] -> w359
            tunnel: w358 -> [w365 w369]
            tunnel: [w365 w369] -> w357
            tunnel: [w363 w367] -> w355
            tunnel: w354 -> [w363 w366]
            frame False {
            }
            frame True {
              n168 = Format Into String(w368) -> (resulting string=w370:string)  [unwired: 3 in, 1 out]
              n169 = Build Array (concatenate)(w366, w368) -> (w367:i16[])
            }
          }
          n170 = Concatenate Strings(w357, w359, "-" ("string")) -> (w360:string)
        }
        n171 = String Length(string=w343) -> (length=w344:i32)
        n172 = Add Array Elements(numeric array=w339) -> (sum=w348:i16)
        n173 = Array Size(array=w339) -> (size(s)=w349:i32)
        n174 = Decrement(x=w344) -> (x-1=w341:i32)
        n175 = To Single Precision Float(number=w348) -> (single precision float=w347:sgl)
        n176 = To Single Precision Float(number=w349) -> (single precision float=w337:sgl)
        n177 = String Subset(string=w343, length (rest)=w341) -> (substring=w342:string)  [unwired: 1 out]
        n178 = Equal To 0?(x=w337) -> (x = 0?=w336:bool)
        n179 = local write "clayCalib"(w342) -> ()
        n180 = case shown="True" w336 {
          tunnel: w347 -> [w352 w353]
          tunnel: w337 -> [w351 _]
          tunnel: [w350 w353] -> w346
          frame False {
            n181 = Divide(x=w352, y=w351) -> (x/y=w350:sgl)
          }
          frame True {
          }
        }
        "clayAverage" <- w346
      }
      event "reportV50_History": Value Change {
        n182 = event-data() -> ()  [unwired: 2 out]
        n183 = local write "lookupRec"(TRUE ("lookupRec")) -> ()
      }
      event "Methods": Value Change {
        n184 = event-data() -> ("CtlRef"=w378:refnum<vi>)  [unwired: 1 out]
        n185 = call "Dropdown Selection (SubVI).vi"("reference"=w378) -> ("element"=w377:string)
        n186 = Equal?(x=w377, y="V50") -> (x = y?=w375:bool)
        n187 = property on="minV50" class="DigNum (strict)"(error in=w374, "Visible"=w375) -> (error out=w373:errorcluster)  [unwired: 1 in, 1 out]
      }
      event "rangeSetup": Value Change {
        n188 = event-data() -> ("NewVal"=w387:u16)  [unwired: 1 out]
        n189 = case shown="2" w387 {
          tunnel: ["0" ("section") "5.0" ("section") "7.5" ("section") "45.0" ("section")] -> w393
          frame 0, Default {
          }
          frame 1 {
          }
          frame 2 {
          }
          frame 3 {
          }
        }
        n190 = local read "configPath"() -> (w395:path)
        n191 = local read "GrainSize"() -> (w386:u16)
        n192 = Greater Than 0?(x=w387) -> (x > 0?=w390:bool)
        n193 = Greater Than 0?(x=w386) -> (x > 0?=w388:bool)
        n194 = call <vilib>:"Open Config Data (compatibility).vi"("error in (no error)"=w383, "configuration file path"=w395) -> ("error out"=w403:errorcluster, "refnum"=w405:T23)  [unwired: 7 in, 1 out]
        n195 = And(x=w390, y=w388) -> (x .and. y?=w389:bool)
        n196 = call-poly <vilib>:"Write Key.vi"("write raw string? (F)"=TRUE, "section"="Ballistic Parameters", "error in (no error)"=w403, "value"=w393, "key"="MidPoint To Target Distance", "refnum"=w405) -> ("error out"=w402:errorcluster, "refnum out"=w401:T23)  [unwired: 4 out]
        n197 = call <vilib>:"Close Config Data.vi"("error in (no error)"=w402, "refnum"=w401) -> ("error out"=w394:errorcluster)  [unwired: 1 in, 8 out]
        n198 = Not(x=w389) -> (.not. x?=w399:bool)
        n199 = Select(t=u8 0 ("y"), s=w389, f=u8 2 ("y")) -> (s? t:f=w385:u8)
        n200 = Scan From String(input string=w393, error in=w394, default 1=sgl 0.0 ("default value 1")) -> (error out=w382:errorcluster, output 1=w392:sgl)  [unwired: 2 in, 2 out]
        n201 = local write "mid_to_targ_dist"(w392) -> ()
        n202 = property on="ARM" class="Bool"(error in=w382, "Disabled"=w385) -> (error out=w381:errorcluster)  [unwired: 1 in, 1 out]
        n203 = property on="addShot" class="Bool"(error in=w381, "Disabled"=w385) -> (error out=w380:errorcluster)  [unwired: 1 in, 1 out]
        n204 = property on="instruct_addShot" class="Str"(error in=w380, "Visible"=w399) -> (error out=w379:errorcluster)  [unwired: 1 in, 1 out]
        "instruct_addShot" <- "RANGE SETUP and THREAT must be selected before shots can be added." ("instruct_addShot")
      }
      event "Drag Corrected", "maxDev": Value Change {
        n205 = event-data() -> ()  [unwired: 2 out]
        n206 = local write "processShots"(TRUE ("ProcessShots")) -> ()
      }
      event "MC Listbox of Shots": Mouse Up {
        n207 = event-data() -> ()  [unwired: 2 out]
        n208 = flat-sequence {
          tunnel: w416 -> [w420]
          tunnel: [w418] -> w415
          tunnel: ["MC Listbox of Shots"] -> w412
          tunnel: w415 -> [w424]
          tunnel: [w423] -> w414
          tunnel: w412 -> [_]
          tunnel: w414 -> [w429]
          tunnel: [w427] -> w413
          frame #0 {
            n209 = property on="Table of Shots" class="Tbl (strict)"(error in=w420) -> (error out=w419:errorcluster, "Value"=w421:string[][])  [unwired: 1 in, 1 out]
            n210 = local write "STOP (Shots MC LB)"(FALSE ("STOP (Shots MC LB)")) -> ()
            n211 = property on="MC Listbox of Shots" class="MCListbox (strict)"(error in=w419, "ItemNames"=w421) -> (error out=w418:errorcluster)  [unwired: 1 in, 1 out]
          }
          frame #1 {
            n212 = control-ref of="MC Listbox of Shots"() -> (w426:refnum<vi>)
            n213 = control-ref of="STOP (Shots MC LB)"() -> (w425:refnum<vi>)
            n214 = call "multicolumn listbox sort.vi"("error IN"=w424, "Bool Refnum"=w425, "MCListbox Refnum"=w426) -> ("error out"=w423:errorcluster)  [unwired: 4 in]
          }
          frame #2 {
            n215 = property on="MC Listbox of Shots" class="MCListbox (strict)"(error in=w429) -> (error out=w428:errorcluster, "ItemNames"=w430:string[][])  [unwired: 1 in, 1 out]
            n216 = property on="Table of Shots" class="Tbl (strict)"(error in=w428, "Val(Sgnl)"=w430) -> (error out=w427:errorcluster)  [unwired: 1 in, 1 out]
          }
        }
      }
      event "PublishNewRecords": Value Change {
        w436 = "\\" ("string")
        w446 = TRUE  # overwrite (F)
        # "2. INSERT new records to Experiments and  \n      Shots tables in local Export.mdb file."
        # "1. SELECT new records from local MDB \n     by comparing against last record numbers \n     found in IMPORT table on BIMS server."
        # "Pushes latest ballistics performance data up to BIMS Server\n\n - Attempts connection with server (reports connection success in msgbox)\n - If successful:\n   - Exports all experiment/shot records since last table marker to [site].mdb file\n   - Sends export.mdb file to drop location on BIMS File Server\n   - Executes SSIS package to import records from export.mdb file\n - Otherwise provides option to try again or cancel"
        # "3. Copy Export.mdb file to [sitename].mdb in [sitename] \n      FileDrop folder on BIMS server."
        n217 = event-data() -> ()  [unwired: 2 out]
        n218 = property on="Loading" class="Ring (strict)"(error in=w442, "Visible"=TRUE) -> (error out=w441:errorcluster)  [unwired: 1 in, 1 out]
        n219 = local read "Site"() -> (w431:string)
        n220 = call "Export New Records.vi"("error IN"=w441, "Site"=w431) -> ("error out"=w448:errorcluster)  [unwired: 3 in, 6 out]
        n221 = Concatenate Strings("\\\\" ("string"), "Server", w436, "Folder", w436, w431, ".mdb" ("string")) -> (w432:string)
        n222 = String To Path(string=w432) -> (path=w444:path)
        n223 = Copy(8:w448, 9:w446, 10:w444, 11:path "C:/Ballistics/Export.mdb" ("source path")) -> (0:w445:errorcluster)  [unwired: 3 out]
        n224 = case shown="No Error" w445 {
          selector: w445 -> [w450 w452]
          tunnel: [w450 w451] -> w440
          frame No Error {
            n225 = One Button Dialog(message="New sample performance records submitted \nto BIMS Warehouse successfully.\n\nPublishing will occur in under five minutes.") -> ()  [unwired: 2 out]
          }
          frame Error {
            n226 = call <vilib>:"General Error Handler.vi"("error in (no error)"=w452) -> ("error out"=w451:errorcluster)  [unwired: 2 in, 12 out]
          }
        }
        n227 = property on="Loading" class="Ring (strict)"(error in=w440, "Visible"=FALSE) -> (error out=w439:errorcluster)  [unwired: 1 in, 1 out]
      }
      event "arrIDC": Mouse Up {
        n228 = event-data() -> ()  [unwired: 2 out]
        "velProfile" <- cluster{dbl, dbl}[] [] ("velProfile")
        "arrIDC" <- dbl[] [] ("arrIDC")
        "relativeTime" <- cluster{"ts2":dbl, "ts3":dbl, "ts1":dbl} {"ts2"=0.0, "ts3"=0.0, "ts1"=0.0} ("relativeTime")
        "velMeasProf" <- T8 {"v2"=0.0, "vB"=0.0, "vOuter"=0.0, "v1"=0.0, "vA"=0.0, "vInner"=0.0} ("velMeasProf")
        "velCompProf" <- cluster{"vStrike":dbl, "vA":dbl} {"vStrike"=0.0, "vA"=0.0} ("velCompProf")
        "displacement" <- T9 {"ds_v2"=6.75, "ds2"=5.0833, "ds_vB"=4.9167, "ds3"=4.75, "ds_vAvg"=6.9167, "ds_v1"=7.0833, "ds1"=8.75, "ds_vA"=8.9167, "ds0"=9.0833} ("displacement")
      }
      event "SampleBackings": Value Change {
        # "Clay is the default sample backing material.\n\n  If another selection is made, then grey out and disable all controls relating to clay."
        n229 = event-data() -> ()  [unwired: 2 out]
        n230 = case shown="0, Default" "SampleBackings" {
          tunnel: [T15."Disabled and Grayed Out" ("Disabled") T15."Enabled" ("Disabled") T15."Disabled and Grayed Out" ("Disabled")] -> w460
          frame 0, Default {
          }
          frame 1 {
          }
          frame 2.. {
          }
        }
        n231 = property on="clayCalArray" class="Arr (strict)"("DisabledEnum"=w460) -> ()  [unwired: 2 in, 2 out]
        n232 = property on="clayAverage" class="DigNum (strict)"("DisabledEnum"=w460) -> ()  [unwired: 2 in, 2 out]
        n233 = property on="clayTemp" class="DigNum (strict)"("DisabledEnum"=w460) -> ()  [unwired: 2 in, 2 out]
      }
      event "RefreshMetadata": Value Change {
        # "Pulls latest metadata down from BIMS Database Server\n - Attempts connection with server \n        (reports failure if connection is unsuccessful)\n - If successful:\n   - Updates local database records from server\n   - Updates dropdown listboxes from local database"
        n234 = event-data() -> ()  [unwired: 2 out]
        n235 = property on="Loading" class="Ring (strict)"(error in=w493, "Visible"=TRUE) -> (error out=w492:errorcluster)  [unwired: 1 in, 1 out]
        n236 = control-ref of="LayerStitchTypes"() -> (w477:refnum<vi>)
        n237 = control-ref of="BackLayer"() -> (w488:refnum<vi>)
        n238 = control-ref of="FrontLayer"() -> (w489:refnum<vi>)
        n239 = control-ref of="ThreatGroups"() -> (w490:refnum<vi>)
        n240 = control-ref of="SampleClamping"() -> (w497:refnum<vi>)
        n241 = control-ref of="SampleTypes"() -> (w514:refnum<vi>)
        n242 = control-ref of="SampleDimensions"() -> (w513:refnum<vi>)
        n243 = control-ref of="ModelMfrs"() -> (w512:refnum<vi>)
        n244 = control-ref of="Assemblers"() -> (w511:refnum<vi>)
        n245 = control-ref of="Submitters"() -> (w510:refnum<vi>)
        n246 = control-ref of="PowderTypes"() -> (w509:refnum<vi>)
        n247 = control-ref of="Methods"() -> (w506:refnum<vi>)
        n248 = control-ref of="TestConditions"() -> (w505:refnum<vi>)
        n249 = control-ref of="SampleBackings"() -> (w504:refnum<vi>)
        n250 = control-ref of="Ballisticians"() -> (w503:refnum<vi>)
        n251 = control-ref of="Shooters"() -> (w502:refnum<vi>)
        n252 = control-ref of="Recorders"() -> (w501:refnum<vi>)
        n253 = control-ref of="SampleCoverings"() -> ()  [unwired: 1 out]
        n254 = Build Array(w477, w488, w489, w490, w497, w514, w513, w512, w511, w510, w509, w506, w505, w504, w503, w502, w501) -> (w508:refnum<vi>[])
        n255 = control-ref of="loadStatus"() -> (w469:refnum<vi>)
        n256 = call "Update Metadata using listbox names.vi"("loadStatus Refnum"=w469, "error in"=w492, "Site"="Site", "RefNumArrIn"=w508) -> ("error out"=w467:errorcluster, "RefNumArrOut"=w507:refnum<vi>[])  [unwired: 6 out]
        n257 = control-ref of="ThreatSize_0"() -> (w471:refnum<vi>)
        n258 = control-ref of="Requestors_0"() -> (w476:refnum<vi>)
        n259 = call "Fill Lists from DB (1st Pass).vi"("error in"=w467, "RefNumArray"=w507) -> ("error out"=w478:errorcluster)  [unwired: 1 in, 4 out]
        n260 = call "Fill Stitch Lists.vi"("error IN"=w478) -> ("error OUT"=w473:errorcluster)  [unwired: 6 in]
        n261 = Build Array(w471, w476) -> (w475:refnum<vi>[])
        n262 = flat-sequence {
          frame #0 {
            n263 = local write "RefreshMetadata"(FALSE ("UpdateMetadata")) -> ()
            n264 = local write "TimeNow"("Loading from BIMS Server . . ." ("TimeNow")) -> ()
          }
        }
        n265 = call "Fill Lists from DB (2nd Pass).vi"("errorIN"=w473, "colNames"=string[] ["GrainSize", "requestor"] ("lkupTableNames"), "lkupTableNames"=string[] ["ThreatDetails", "Submitters"], "RefNumArray"=w475) -> ("error OUT"=w472:errorcluster)  [unwired: 3 in]
        n266 = property class="Str"(reference=w469, error in=w467, "Value"="filling dropdown lists") -> (reference out=w468:refnum<vi>)  [unwired: 1 out]
        n267 = call "Create local tables from Server DB.vi"("loadStatus Refnum"=w468, "error in"=w472, "Site"="Site", "tableNames"=string[] ["Threats", "ThreatDetails", "ThreatCalibers", "Mfrs", "SampleStyles", "SampleSpecs", "FiberTypes"]) -> ("error out"=w499:errorcluster)  [unwired: 7 out]
        n268 = call "Fill Lists From DB (3rd Pass).vi"("error IN"=w499) -> ("error OUT"=w480:errorcluster)  [unwired: 3 in, 3 out]
        n269 = control-ref of="ModelMfrs"() -> (w487:refnum<vi>)
        n270 = property class="Ring (strict)"(reference=w487, error in=w480) -> (reference out=w486:refnum<vi>, error out=w485:errorcluster, "Strings []"=w484:string[])
        n271 = Delete From Array(array=w484, length=1, index=0) -> (array with subset deleted=w483:string[])  [unwired: 1 out]
        n272 = property class="Ring (strict)"(reference=w486, error in=w485, "Strings []"=w483) -> (error out=w479:errorcluster)  [unwired: 1 out]
        n273 = case shown="No Error" w479 {
          selector: w479 -> [w516 w519]
          tunnel: [w516 w519] -> w496
          frame No Error {
            n274 = local write "TimeNow"("Collector Metadata is READY!" ("TimeNow")) -> ()
            n275 = Wait (ms)(milliseconds to wait=u32 2000) -> ()  [unwired: 1 out]
            "loadStatus" <- ""
          }
          frame Error {
            n276 = call <vilib>:"General Error Handler.vi"("error in (no error)"=w519) -> ()  [unwired: 2 in, 13 out]
          }
        }
        n277 = property on="Loading" class="Ring (strict)"(error in=w496, "Visible"=FALSE) -> (error out=w495:errorcluster)  [unwired: 1 in, 1 out]
      }
      event "loadingUnits": Value Change {
        n278 = local read "Powder Loading"() -> (w523:sgl)
        n279 = event-data() -> ("NewVal"=w522:enum32{"grams", "grains"})  [unwired: 6 out]
        n280 = case shown="\"grams\", Default" w522 {
          tunnel: w523 -> [w527 w528]
          frame "grams", Default {
            n281 = Multiply(x=w527, y=sgl 0.06479891) -> (x*y=w525:sgl)
            n282 = local write "Powder Loading"(w525) -> ()
          }
          frame "grains" {
            n283 = Multiply(x=w528, y=sgl 15.432359) -> (x*y=w529:sgl)
            n284 = local write "Powder Loading"(w529) -> ()
          }
        }
      }
      event "clearErrors": Value Change {
        w531 = errorcluster {"status"=FALSE, "code"=0, "source"=""} ("error in")
        n285 = event-data() -> ()  [unwired: 7 out]
        n286 = local write "SMErr"(w531) -> ()
      }
    }
    "U/I EvErr" <- w31
  }
  n287 = while "Test Executive State Machine" {
    shift-left: 100 -> [w540]
    shift-right: [w541] -> _
    shift-left: Collector_State."INITIALIZE" ("progState") -> [w537]
    shift-right: [w534] -> _
    shift-right: [w538] -> _
    shift-left: w26 -> [w539]
    shift-right: [w535] -> _
    shift-left: w22 -> [w536]
    tunnel: w3 -> [w532]
    stop <- FALSE stop-if-true
    n288 = case shown="\"CHECK DAQ\"" w537 {
      tunnel: [w561 w673 Collector_State."POLL" ("progState") Collector_State."POLL" ("progState") w1618 Collector_State."PROC SHOTS" ("progState") Collector_State."POLL" ("progState") Collector_State."PROC SHOTS" ("progState") Collector_State."PROC SHOTS" ("progState") Collector_State."POLL" ("progState") Collector_State."POLL" ("progState") w2218] -> w534
      tunnel: [-1 -1 ("index of element") -1 ("index of element") -1 ("index of element") w1617 -1 ("index of element") -1 -1 ("index of element") -1 ("index of element") -1 -1 ("index of element") w2217] -> w541
      tunnel: w540 -> [_ w674 _ _ _ _ _ _ _ _ _ _]
      tunnel: w539 -> [w564 w672 w825 w1366 w1612 w1847 w1889 w1899 w1917 w1968 w1982 w2219]
      tunnel: [w556 w671 w825 w1366 w1611 w1833 w1893 w1899 w1914 w1968 w1986 w2219] -> w538
      tunnel: w536 -> [_ w667 w822 w1364 w1614 w1843 w1885 w1902 w1913 w1965 w1981 w2211]
      tunnel: [w567 w668 w821 w1363 w1613 w1841 w1885 w1900 w1912 w1964 w1980 w2216] -> w535
      tunnel: w532 -> [_ _ _ _ _ _ _ _ _ _ _ w2210]
      frame "POLL", Default {
        w565 = Collector_State."POLL"  # progStateType
        w577 = TRUE  # element
        w580 = 4  # SAVE
        # "case # 0"
        # "This section checks for any buttons, maintains routine check of the parameters"
        n289 = case shown="\"Measure\"" "mainTabCntrl" {
          frame "Setup", Default {
            n290 = control-ref of="layerStitch_1"() -> (w597:refnum<vi>)
            n291 = control-ref of="layerStitch_2"() -> (w596:refnum<vi>)
            n292 = control-ref of="layerStitch_3"() -> (w595:refnum<vi>)
            n293 = control-ref of="layerStitch_4"() -> (w594:refnum<vi>)
            n294 = control-ref of="layerStitch_5"() -> (w593:refnum<vi>)
            n295 = control-ref of="layerStitch_6"() -> (w592:refnum<vi>)
            n296 = control-ref of="SampleStyle_0"() -> (w590:refnum<vi>)
            n297 = control-ref of="SampleStyle_1"() -> (w611:refnum<vi>)
            n298 = control-ref of="SampleStyle_2"() -> (w612:refnum<vi>)
            n299 = control-ref of="SampleStyle_3"() -> (w613:refnum<vi>)
            n300 = control-ref of="SampleStyle_4"() -> (w614:refnum<vi>)
            n301 = control-ref of="SampleStyle_5"() -> (w615:refnum<vi>)
            n302 = control-ref of="SampleStyle_6"() -> (w616:refnum<vi>)
            n303 = Build Array(w597, w596, w595, w594, w593, w592) -> (w598:refnum<vi>[])
            n304 = global write "BIMS_Collector Globals.vi" "LayerStitchTypeRefs"(w598) -> ()
            n305 = Build Array(w590, w611, w612, w613, w614, w615, w616) -> (w609:refnum<vi>[])
            n306 = global write "BIMS_Collector Globals.vi" "SampleStyles"(w609) -> ()
            n307 = local read "Fabric Description"() -> (w601:string)
            n308 = control-ref of="Mfr_0"() -> (w591:refnum<vi>)
            n309 = control-ref of="Mfr_1"() -> (w622:refnum<vi>)
            n310 = control-ref of="Mfr_2"() -> (w621:refnum<vi>)
            n311 = control-ref of="Mfr_3"() -> (w620:refnum<vi>)
            n312 = control-ref of="Mfr_4"() -> (w619:refnum<vi>)
            n313 = control-ref of="Mfr_5"() -> (w618:refnum<vi>)
            n314 = control-ref of="Mfr_6"() -> (w617:refnum<vi>)
            n315 = String Subset(string=w601, length (rest)=75 ("length (rest)")) -> (substring=w600:string)  [unwired: 1 out]
            n316 = Build Array(w591, w622, w621, w620, w619, w618, w617) -> (w610:refnum<vi>[])
            n317 = local write "Fabric Description"(w600) -> ()
            n318 = global write "BIMS_Collector Globals.vi" "Mfrs"(w610) -> ()
            n319 = local read "SampleAttribs_1"() -> (w603:T3)
            n320 = local read "SampleAttribs_2"() -> (w605:T3)
            n321 = local read "SampleAttribs_3"() -> (w606:T3)
            n322 = local read "SampleAttribs_4"() -> (w607:T3)
            n323 = local read "SampleAttribs_5"() -> (w608:T3)
            n324 = local read "SampleAttribs_6"() -> (w604:T3)
            n325 = Build Array(w603, w605, w606, w607, w608, w604) -> (w602:T27)
            n326 = global write "BIMS_Collector Globals.vi" "SampleAttribs"(w602) -> ()
          }
          frame "Measure" {
            # "Disable and gray out the \"Save\" button\nIF the shot table has no shots, \nOR if there are no plies; otherwise, enable it."
            # "Disable and gray out the \"Clear Shots\" button\nIF the shot table has no shots; otherwise, enable it."
            n327 = local read "shotsArr"() -> (w627:T6)
            n328 = local read "totalNumLayers"() -> (w625:i32)
            n329 = Equal To 0?(x=w625) -> (x = 0?=w626:bool)
            n330 = Array Size(array=w627) -> (size(s)=w637:i32)
            n331 = Equal To 0?(x=w637) -> (x = 0?=w624:bool)
            n332 = Or(x=w624, y=w626) -> (x .or. y?=w623:bool)
            n333 = property on="saveReq" class="Str"("Visible"=w623) -> ()  [unwired: 2 in, 2 out]
            n334 = Select(t=T15."Disabled and Grayed Out" ("Disabled"), s=w623, f=T15."Enabled" ("Disabled")) -> (s? t:f=w628:T15)
            n335 = Select(t=T15."Disabled and Grayed Out" ("Disabled"), s=w624, f=T15."Enabled" ("Disabled")) -> (s? t:f=w636:T15)
            n336 = property on="reportV50" class="Bool"("Disabled"=w628) -> ()  [unwired: 2 in, 2 out]
            n337 = property on="saveShots" class="Bool"("Disabled"=w628) -> ()  [unwired: 2 in, 2 out]
            n338 = property on="clearShots" class="Bool"("Disabled"=w636) -> ()  [unwired: 2 in, 2 out]
            n339 = local read "Shot Description"() -> (w635:string)
            n340 = String Subset(string=w635, length (rest)=30 ("length (rest)")) -> (substring=w633:string)  [unwired: 1 out]
            n341 = local write "Shot Description"(w633) -> ()
          }
          frame "History" {
          }
          frame "System" {
          }
        }
        n342 = Format Date/Time String(time format string (%c)="%x   %H:%M:%S") -> (date/time string=w553:string)  [unwired: 2 out]
        n343 = local write "shotTimestamp"(w553) -> ()
        n344 = Or(x="undoLastShot", y="deleteShot") -> (x .or. y?=w575:bool)
        n345 = Or(x="reportV50", y="reportV50_History") -> (x .or. y?=w583:bool)
        n346 = flat-sequence {
          tunnel: [w644] -> w566
          frame #0 {
            n347 = Wait (ms)(milliseconds to wait=u32 10 ("millisecond timer value")) -> ()  [unwired: 1 out]
          }
          frame #1 {
            n348 = local read "SMErr"() -> (w644:errorcluster)
          }
        }
        n349 = Build Array("RESET All", w583, "VsVr Report", "saveShots", "addShot", "clearShots", "nextShot", w575, "readyClock", "processShots") -> (w578:bool[])
        n350 = Search 1D Array(1D array=w578, element=w577) -> (index of element=w588:i32)  [unwired: 1 out]
        n351 = Increment(x=w588) -> (x+1=w589:i32)
        n352 = Equal?(x=w589, y=w580) -> (x = y?=w581:bool)
        n353 = case shown="False" w581 {
          tunnel: w589 -> [w646 w658]
          tunnel: [w647 w663] -> w587
          tunnel: w566 -> [w645 w654]
          tunnel: [w645 w652] -> w567
          frame False {
            w649 = 0  # Not Found
            n354 = Equal?(x=w646, y=w649) -> (x = y?=w648:bool)
            n355 = case shown="True" w648 {
              tunnel: w646 -> [w650 _]
              tunnel: [w650 w651] -> w647
              frame False {
              }
              frame True {
                w651 = 11  # CheckDAQ
                # "USUAL SCENARIO"
              }
            }
          }
          frame True {
            # "Before allowing data record to be saved,\nprompt user to validate."
            n356 = call "Get Last Record (SubVI).vi"("error in"=w654) -> ("error out"=w653:errorcluster, "experiment record"=w655:i32, "shot record"=w656:i32)  [unwired: 2 out]
            n357 = local write "lastSamp"(w655) -> ()
            n358 = local write "lastShot"(w656) -> ()
            n359 = To Double Precision Float(number=w655) -> (double precision float=w657:dbl)
            n360 = Two Button Dialog(message="Are ALL Data Valid?", 1:"NO" ("F button name (\"Cancel\")"), 2:"YES" ("T button name (\"OK\")")) -> (T button?=w662:bool)
            n361 = property on="Record #" class="DigNum (strict)"(error in=w653, "Maximum"=w657) -> (error out=w652:errorcluster)  [unwired: 1 in, 1 out]
            n362 = case shown="False" w662 {
              tunnel: [0 ("index of element") w665] -> w663
              tunnel: w658 -> [_ w665]
              frame False {
                # "POLL"
              }
              frame True {
              }
            }
          }
        }
        n363 = local read "shotsArr"() -> (w556:T6)
        n364 = for {
          tunnel: w564 -> [w641] mode=indexing
          tunnel: w556 -> [w642] mode=indexing
          tunnel: [w638] -> w563 mode=indexing
          n365 = Not Equal?(x=w642, y=w641) -> (x != y?=w640:T28)
          n366 = Cluster To Array(cluster=w640) -> (array=w639:bool[])
          n367 = Or Array Elements(Boolean array=w639) -> (logical OR=w638:bool)
        }
        n368 = Or Array Elements(Boolean array=w563) -> (logical OR=w559:bool)
        n369 = To Variant(anything=w587) -> (Variant=w586:variant)
        n370 = Variant To Data(type=w565, Variant=w586) -> (data=w562:T13)  [unwired: 1 in, 1 out]
        n371 = Select(t=Collector_State."PROC SHOTS" ("progStateType"), s=w559, f=w562) -> (s? t:f=w561:T13)
        "STOP (Shots MC LB)" <- TRUE ("STOP (Shots MC LB)")
      }
      frame "INITIALIZE" {
        # "case # 1"
        # "This section reads the ini file"
        n372 = case shown="100" w674 {
          tunnel: [w680 w699] -> w675
          tunnel: [w678 w699] -> w670
          tunnel: w667 -> [w677 w691]
          tunnel: [w676 w691] -> w666
          frame 0, Default {
            n373 = local read "RESET All"() -> (w679:bool)
            n374 = case shown="False" w679 {
              tunnel: [TRUE w687] -> w680
              tunnel: [FALSE w687] -> w678
              tunnel: w677 -> [w681 w684]
              tunnel: [w681 w684] -> w676
              frame False {
                # "Refresh"
              }
              frame True {
                n375 = Two Button Dialog(message="Resetting will remove all unsaved data.\n\nDo you really  want to reset? ", 1:"NO" ("F button name (\"Cancel\")"), 2:"YES" ("T button name (\"OK\")")) -> (T button?=w687:bool)
              }
            }
          }
          frame 100 {
            w699 = TRUE  # Reset ALL
            n376 = control-ref of="Mfr_0"() -> (w689:refnum<vi>)
            n377 = control-ref of="Mfr_1"() -> (w698:refnum<vi>)
            n378 = control-ref of="Mfr_2"() -> (w697:refnum<vi>)
            n379 = control-ref of="Mfr_3"() -> (w696:refnum<vi>)
            n380 = control-ref of="Mfr_4"() -> (w695:refnum<vi>)
            n381 = control-ref of="Mfr_5"() -> (w694:refnum<vi>)
            n382 = control-ref of="Mfr_6"() -> (w693:refnum<vi>)
            n383 = property on="Loading" class="Ring (strict)"("Visible"=FALSE) -> ()  [unwired: 2 in, 2 out]
            n384 = Build Array(w689, w698, w697, w696, w695, w694, w693) -> (w692:refnum<vi>[])
            n385 = global write "BIMS_Collector Globals.vi" "Mfrs"(w692) -> ()
          }
        }
        n386 = case shown="True" w675 {
          tunnel: [Collector_State."POLL" ("progState") w741] -> w673
          tunnel: w672 -> [w702 _]
          tunnel: [w702 "shotsArr"] -> w671
          tunnel: w670 -> [_ w742]
          tunnel: [w700 w709] -> w668
          tunnel: w666 -> [w700 w740]
          frame False {
            n387 = local write "RESET All"(FALSE ("RESET")) -> ()
          }
          frame True {
            n388 = case shown="True" w742 {
              selector: w742 -> [_ w768]
              tunnel: [w751 w768] -> w723
              tunnel: [w750 w783] -> w705
              tunnel: w740 -> [w750 w770]
              tunnel: [w749 w767] -> w711
              frame False {
                w751 = FALSE  # Reset All
                # "Refresh"
                n389 = local read "configPath"() -> (w749:path)
              }
              frame True {
                # "This section resets\nentire program"
                # "Reset ALL"
                n390 = control-ref of="This VI"() -> (w760:refnum<vi>)
                n391 = invoke on="Invoke Node" class="VI" method="Default Vals.Reinit All"(reference=w760, error in=w770) -> (reference out=w759:refnum<vi>, error out=w758:errorcluster)  [unwired: 1 in, 1 out]
                n392 = property class="VI"(reference=w759, error in=w758, "Front Panel.ShowMenuBar"=FALSE ("Front Panel Window:Show Menu Bar")) -> (reference out=w756:refnum<vi>, error out=w754:errorcluster)
                n393 = control-ref of="ScreenSetAvgg"() -> (w778:refnum<vi>)
                n394 = control-ref of="InterlockExists"() -> (w779:refnum<vi>)
                n395 = control-ref of="useBallisitican"() -> (w780:refnum<vi>)
                n396 = control-ref of="useRecorder"() -> (w781:refnum<vi>)
                n397 = control-ref of="useShooter"() -> (w782:refnum<vi>)
                n398 = control-ref of="useBMC"() -> (w753:refnum<vi>)
                n399 = property on="mainTabCntrl" class="TabCtl (strict)"() -> (error out=w762:errorcluster, "Pages"=w764:refnum<vi>[])  [unwired: 2 in, 1 out]
                n400 = Close Reference(reference=w756, error in (no error)=w754) -> (error out=w755:errorcluster)
                n401 = call "RegReadParams.vi"("ScreenSetAveraging_Ref"=w778, "useBMC_Ref"=w753, "InterlockExist_Ref"=w779, "errorIN"=w755, "useShooter_Ref"=w782, "useRecorder_Ref"=w781, "useBallistician_Ref"=w780) -> ("error out"=w777:errorcluster)  [unwired: 4 out]
                n402 = Index Array(array=w764, index=1) -> (element=w766:refnum<vi>)
                n403 = control-ref of="Server"() -> (w769:refnum<vi>)
                n404 = control-ref of="ConfigName"() -> (w773:refnum<vi>)
                n405 = control-ref of="Site"() -> (w771:refnum<vi>)
                n406 = control-ref of="Folder"() -> (w752:refnum<vi>)
                n407 = property on="Property Node" class="Page"(reference=w766, error in=w762, "PageEnb"=T16."Page Disabled & Grayed" ("Page Enabled State")) -> (error out=w761:errorcluster)  [unwired: 1 out]
                n408 = Build Array(w773, w771, w769, w752) -> (w774:refnum<vi>[])
                n409 = property on="minV50" class="DigNum (strict)"(error in=w761, "Visible"=w768) -> ()  [unwired: 1 in, 2 out]
                n410 = call "InitStringValuesFromRegistry(SubVI).vi"("error in"=w777, "String References"=w774, "subkey"="SOFTWARE\\DuPont\\BIMS-14\\Collector", "root key (HKEY_LOCAL_MACHINE)"=Registry_RtKey."HKEY_LOCAL_MACHINE") -> ("error out"=w776:errorcluster)  [unwired: 3 out]
                n411 = Current VI's Path() -> (path=w786:path)
                n412 = call "Initialize (SubVI).vi"("path"=w786, "error IN"=w776) -> ("pathConfigOUT"=w767:path, "lengthUnits"=→"lengthUnits":string, "massUnits"=→"massUnits":string, "error out"=w783:errorcluster)  [unwired: 1 out]
                "configPath" <- w767
              }
            }
            n413 = control-ref of="MeasSrc"() -> (w707:refnum<vi>)
            n414 = call "check timing board (SubVI).vi"("errIN"=w705, "ActiveDev"="ActiveDev", "measSrc_ref"=w707) -> ("error out"=w704:errorcluster, "deviceID"=→"Device S/N":string)  [unwired: 7 in]
            n415 = property on="Ballisticians" class="Ring (strict)"("Visible"="useBallisitican") -> ()  [unwired: 2 in, 2 out]
            n416 = property on="Shooters" class="Ring (strict)"("Visible"="useShooter") -> ()  [unwired: 2 in, 2 out]
            n417 = property on="Recorders" class="Ring (strict)"("Visible"="useRecorder") -> ()  [unwired: 2 in, 2 out]
            n418 = control-ref of="Threat"() -> (w726:refnum<vi>)
            n419 = control-ref of="SampleTypes"() -> (w728:refnum<vi>)
            n420 = control-ref of="SampleDescrip"() -> (w735:refnum<vi>)
            n421 = call "Get Threats (SubVI).vi"("pathConfigIN"=w711, "refThreat"=w726, "error in"=w704) -> ("pathConfigOUT"=w730:path, "factorOut"=→"factor array":sgl[], "error out"=w733:errorcluster)  [unwired: 4 out]
            n422 = Bundle("SampleTypes"=w728, "SampleDescrip"=w735) -> (w734:T29)  [unwired: 1 out]
            n423 = call "Fill Lists from INI (SubVI).vi"("clusterListboxes"=w734, "error in"=w733, "pathConfigIN"=w730) -> ("error out"=w732:errorcluster, "pathConfigOUT"=w731:path)  [unwired: 4 out]
            n424 = call "Read Parameters.vi"("error in (no error)"=w732, "appended path"=w731) -> ("error out"=w725:errorcluster, "rangeParams"=w727:T30)  [unwired: 4 out]
            n425 = Unbundle(w727) -> ("max dev"=w712:sgl, "residual separation"=→"Residual/Separation":sgl, "Set#1 Separation"=→"Set#1 Separation":sgl, "Set#2 Separation"=→"Set#2 Separation":sgl, "impact target dist"=w716:sgl, "resid target dist"=w717:sgl, "barrel screen dist"=→"Barrel to Screen":sgl, "midpt_to_target_dist"=→"mid_to_targ_dist":sgl)
            n426 = local write "maxDev"(w712) -> ()
            n427 = local write "Set#1_to_Target"(w716) -> ()
            n428 = local write "Residual/Target Dist"(w717) -> ()
            n429 = property on="RefreshMetadata" class="Bool (strict)"(error in=w725, "Val(Sgnl)"=TRUE) -> (error out=w720:errorcluster)  [unwired: 1 in, 1 out]
            n430 = case shown="True" w723 {
              tunnel: [Collector_State."POLL" ("progState") w809] -> w741
              tunnel: [w787 w789] -> w739
              tunnel: w720 -> [w787 w806]
              tunnel: w711 -> [_ w797]
              tunnel: "useBMC" -> [_ w796]
              frame False {
                # "Refresh"
              }
              frame True {
                w790 = T15."Disabled and Grayed Out" ("Disabled")
                # "Reset ALL"
                n431 = global read "BIMS_Collector Globals.vi" "SampleStyles"() -> (w799:refnum<vi>[])
                n432 = local read "InterlockExists"() -> (w808:bool)
                n433 = case shown="True" w796 {
                  tunnel: w797 -> [_ w811]
                  frame False {
                  }
                  frame True {
                    n434 = Path To String(path=w811) -> (string=w812:string)
                    n435 = call "Ballistics Message Center.vi"("INI File Name"=w812) -> ()
                  }
                }
                n436 = local read "MeasSrc"() -> (w810:T12)
                n437 = call "Get Last Record (SubVI).vi"("error in"=w806) -> ("error out"=w798:errorcluster, "experiment record"=w804:i32, "shot record"=→"lastShot":i32)  [unwired: 2 out]
                "lastSamp" <- w804
                n438 = control-ref of="ThreatDetails"() -> (w795:refnum<vi>)
                n439 = control-ref of="SampleStyle_0"() -> (w801:refnum<vi>)
                n440 = control-ref of="ThreatGroups"() -> (w800:refnum<vi>)
                n441 = To Double Precision Float(number=w804) -> (double precision float=w803:dbl)
                n442 = case shown="\"Screens\"" w810 {
                  tunnel: [Collector_State."POLL" ("progState") Collector_State."POLL" ("progState") Collector_State."READY CLOCK" ("progState")] -> w809
                  frame "Simulated", Default {
                  }
                  frame "Radar" {
                  }
                  frame "Screens" {
                    # "check for PCI 6602"
                  }
                }
                n443 = Build Array (concatenate)(w795, w801, w800, w799) -> (w802:refnum<vi>[])
                n444 = property on="Record #" class="DigNum (strict)"(error in=w798, "Maximum"=w803) -> (error out=w789:errorcluster)  [unwired: 1 in, 1 out]
                n445 = Select(t=T15."Enabled" ("Disabled"), s=w808, f=T15."Disabled and Grayed Out" ("Disabled")) -> (s? t:f=w807:T15)
                n446 = for {
                  tunnel: w802 -> [w813] mode=indexing
                  n447 = property on="Property Node" class="Ring (strict)"(reference=w813, "Strings []"=string[] []) -> ()  [unwired: 1 in, 2 out]
                }
                n448 = property on="addShot" class="Bool"("Disabled"=T15."Enabled") -> ()  [unwired: 2 in, 2 out]
                n449 = property on="undoLastShot" class="Bool"("Disabled"=w790) -> ()  [unwired: 2 in, 2 out]
                n450 = property on="saveShots" class="Bool"("Disabled"=w790) -> ()  [unwired: 2 in, 2 out]
                n451 = property on="clearShots" class="Bool"("Disabled"=w790) -> ()  [unwired: 2 in, 2 out]
                n452 = property on="ARM" class="Bool"("Disabled"=w807) -> ()  [unwired: 2 in, 2 out]
                n453 = property on="saveReq" class="Str"("Visible"=TRUE) -> ()  [unwired: 2 in, 2 out]
              }
            }
            n454 = call <vilib>:"General Error Handler.vi"("error in (no error)"=w739) -> ("error out"=w709:errorcluster)  [unwired: 2 in, 12 out]
            n455 = flat-sequence {
              tunnel: w709 -> [w743]
              frame #0 {
                n456 = local read "ConfigName"() -> (w744:string)
                n457 = case shown="No Error" w743 {
                  tunnel: [w747 "NOT READY!" ("ConfigName")] -> w745
                  tunnel: w744 -> [w747 _]
                  frame No Error {
                    n458 = Wait (ms)(milliseconds to wait=u32 1000) -> ()  [unwired: 1 out]
                  }
                  frame Error {
                  }
                }
                "ConfigName" <- w745
              }
            }
            "saveReq" <- "Number of layers in sample ply specification and number of shots in shots table must be greater than 0 to enable saving." ("saveReq")
          }
        }
      }
      frame "V50 Report or GET Record" {
        # "case # 2"
        # "The custom Excel template file is \nexpected in the C:\\Ballistics folder."
        n459 = case shown="True" "lookupRec" {
          selector: "lookupRec" -> [_ w1345]
          tunnel: [w868 w1335] -> w849
          tunnel: [w867 w1321] -> w848
          tunnel: [w866 w1338] -> w847
          tunnel: [w865 w1278] -> w846
          tunnel: [w864 w1336] -> w845
          tunnel: [w863 w1298] -> w844
          tunnel: [w862 w1285] -> w831
          tunnel: [w861 w1287] -> w830
          tunnel: [w860 w1288] -> w829
          tunnel: [w859 "Record #"] -> w828
          tunnel: [w858 w1337] -> w827
          tunnel: [w857 w1287] -> w820
          tunnel: w825 -> [w856 _]
          tunnel: [w855 w1310] -> w823
          tunnel: w822 -> [w855 w1311]
          tunnel: [w854 w1283] -> w818
          frame False {
            n460 = stacked-sequence {
              tunnel: [_ _ _ _ _ w1198] -> w863
              tunnel: [_ w937 _ _ _ _] -> w867
              tunnel: [_ _ _ _ w1042 _] -> w864
              tunnel: [_ _ _ w988 _ _] -> w865
              tunnel: [_ _ w959 _ _ _] -> w866
              tunnel: [w880 _ _ _ _ _] -> w868
              tunnel: [_ _ _ _ _ w1204] -> w862
              tunnel: [_ _ _ _ _ w1200] -> w861
              tunnel: [_ _ _ _ _ w1199] -> w860
              tunnel: [_ _ _ _ _ w1203] -> w859
              tunnel: [_ _ _ _ _ w1202] -> w858
              tunnel: [_ _ _ _ _ w1201] -> w857
              tunnel: w856 -> [_ _ w958 _ w1041 _]
              frame #0 {
                # "Need to remove first element\nsince it's associated with the \nhistory page."
                # "FABRIC"
                n461 = local read "fab1_totalWt"() -> (w883:sgl)
                n462 = local read "fab3_totalWt"() -> (w885:sgl)
                n463 = local read "fab5_totalWt"() -> (w887:sgl)
                n464 = global read "BIMS_Collector Globals.vi" "SampleStyles"() -> (w871:refnum<vi>[])
                n465 = global read "BIMS_Collector Globals.vi" "Mfrs"() -> (w876:refnum<vi>[])
                n466 = local read "fab2_totalWt"() -> (w884:sgl)
                n467 = local read "fab4_totalWt"() -> (w886:sgl)
                n468 = local read "fab6_totalWt"() -> (w888:sgl)
                n469 = global read "BIMS_Collector Globals.vi" "LayerStitchTypeRefs"() -> (w878:refnum<vi>[])
                n470 = global read "BIMS_Collector Globals.vi" "SampleAttribs"() -> (w869:T21)
                n471 = global read "BIMS_Collector Globals.vi" "LayerSpecs"() -> (w879:T31)
                n472 = Delete From Array(array=w871, length=1, index=0) -> (array with subset deleted=w870:refnum<vi>[])  [unwired: 1 out]
                n473 = Delete From Array(array=w876, length=1, index=0) -> (array with subset deleted=w877:refnum<vi>[])  [unwired: 1 out]
                n474 = Build Array(w883, w884, w885, w886, w887, w888) -> (w882:sgl[])
                n475 = for {
                  tunnel: w882 -> [w892] mode=indexing
                  tunnel: [w900] -> w881 mode=indexing
                  tunnel: w869 -> [w899] mode=indexing
                  tunnel: w879 -> [w898] mode=indexing
                  tunnel: w877 -> [w897] mode=indexing
                  tunnel: w870 -> [w896] mode=indexing
                  tunnel: w878 -> [w895] mode=indexing
                  n476 = call "Dropdown Selection (SubVI).vi"("reference"=w897) -> ("element"=w890:string)
                  n477 = call "Dropdown Selection (SubVI).vi"("reference"=w896) -> ("element"=w894:string)
                  n478 = Equal?(x="", y=w890) -> (x = y?=w889:bool)
                  n479 = call "Dropdown Selection (SubVI).vi"("reference"=w895) -> ("element"=w893:string)
                  n480 = case shown="False" w889 {
                    tunnel: [w919 w921] -> w900
                    tunnel: w899 -> [w918 _]
                    tunnel: w898 -> [w917 _]
                    tunnel: w894 -> [w911 _]
                    tunnel: w893 -> [w906 _]
                    tunnel: w892 -> [w904 _]
                    tunnel: w890 -> [w903 _]
                    frame False {
                      n481 = Unbundle By Name(w917) -> ("numOfPlies"=w905:i32, "LotNum"=w914:string, "RollNum"=w915:string)
                      n482 = Unbundle By Name(w918) -> ("internal_ID"=w909:string, "fiber"=w910:string, "denier"=w913:string, "pick"=w912:string, "weave"=w907:string, "finish"=w908:string, "ozPerYd2"=w916:string)
                      n483 = Format Into String(w905) -> (resulting string=w902:string)  [unwired: 3 in, 1 out]
                      n484 = Format Into String(w904) -> (resulting string=w901:string)  [unwired: 3 in, 1 out]
                      n485 = Build Array(w902, w903, w911, w909, w910, w913, w912, w907, w908, w914, w915, w916, w901, w906) -> (w919:string[])
                    }
                    frame True {
                      n486 = Initialize Array("", 14 ("dimension size")) -> (w921:string[])
                    }
                  }
                }
                n487 = Transpose 2D Array(2D array=w881) -> (transposed array=w880:string[][])
              }
              frame #1 {
                w923 = "%.1f" ("format string")
                # "muzzel / midpoint"
                # "muzzle / scr#1"
                # "muzzle / target"
                # "scr#2 / target"
                # "RANGE"
                n488 = local read "Set#1 Separation"() -> (w930:sgl)
                n489 = local read "mid_to_targ_dist"() -> (w927:sgl)
                n490 = local read "Barrel to Screen"() -> (w924:sgl)
                n491 = local read "clayAverage"() -> (w945:sgl)
                n492 = Divide(x=w930, y=sgl 2.0) -> (x/y=w925:sgl)
                n493 = local read "RoomHum"() -> (w940:sgl)
                n494 = local read "clayTemp"() -> (w943:sgl)
                n495 = local read "clayCalib"() -> (w946:string)
                n496 = local read "RoomT"() -> (w941:sgl)
                n497 = Add(x=w924, y=w927) -> (x+y=w931:sgl)
                n498 = Subtract(x=w924, y=w925) -> (x-y=w926:sgl)
                n499 = Subtract(x=w927, y=w925) -> (x-y=w928:sgl)
                n500 = Format Into String(w931) -> (resulting string=w932:string)  [unwired: 3 in, 1 out]
                n501 = Format Into String(w926) -> (resulting string=w933:string)  [unwired: 3 in, 1 out]
                n502 = Format Into String(w930) -> (resulting string=w934:string)  [unwired: 3 in, 1 out]
                n503 = Format Into String(w928) -> (resulting string=w935:string)  [unwired: 3 in, 1 out]
                n504 = Format Into String(w927) -> (resulting string=w936:string)  [unwired: 3 in, 1 out]
                n505 = Format Into String(w940) -> (resulting string=w938:string)  [unwired: 3 in, 1 out]
                n506 = Format Into String(format string=w923, w941) -> (resulting string=w939:string)  [unwired: 2 in, 1 out]
                n507 = Format Into String(format string=w923, w943) -> (resulting string=w942:string)  [unwired: 2 in, 1 out]
                n508 = Format Into String(format string=w923, w945) -> (resulting string=w944:string)  [unwired: 2 in, 1 out]
                n509 = Bundle(w932, w933, w934, w935, w936, w938, w939, w942, "clayCalib"=w946, w944) -> (w947:T32)  [unwired: 1 out]
                n510 = Cluster To Array(cluster=w947) -> (array=w937:string[])
              }
              frame #2 {
                # "RESULTS"
                n511 = control-ref of="Methods"() -> (w948:refnum<vi>)
                n512 = call "Dropdown Selection (SubVI).vi"("reference"=w948) -> ("element"=w949:string)
                n513 = for {
                  tunnel: w958 -> [w986] mode=indexing
                  tunnel: [w985] -> w957 mode=indexing
                  tunnel: [w984] -> w956
                  i -> [w984]
                  n514 = Unbundle By Name(w986) -> ("BackFace\nDepth"=w985:sgl)
                }
                n515 = Increment(x=w956) -> (x+1=w954:i32)
                n516 = Add Array Elements(numeric array=w957) -> (sum=w955:sgl)
                n517 = To Single Precision Float(number=w954) -> (single precision float=w953:sgl)
                n518 = Divide(x=w955, y=w953) -> (x/y=w952:sgl)
                n519 = Format Into String(format string="%1.1f", w952) -> (resulting string=w951:string)  [unwired: 2 in, 1 out]
                n520 = case shown="\"V50\"" w949 {
                  tunnel: [w974 w983] -> w961
                  tunnel: w951 -> [w962 w982]
                  frame "V50" {
                    w968 = "%1d" ("format string")
                    n521 = local read "Z.M.R."() -> (w966:sgl)
                    n522 = Less Than 0?(x=w966) -> (x < 0?=w967:bool)
                    n523 = local read "rangeOfResults"() -> (w970:i32)
                    n524 = local read "computed_V50"() -> (w973:sgl)
                    n525 = local read "lowComplete"() -> (w971:i32)
                    n526 = local read "highPartial"() -> (w972:i32)
                    n527 = case shown="True" w967 {
                      tunnel: w966 -> [w979 _]
                      tunnel: [w979 sgl 0.0 ("Z.M.R.")] -> w965
                      frame False {
                      }
                      frame True {
                      }
                    }
                    n528 = Format Into String(format string="%1.1f", w973) -> (resulting string=w977:string)  [unwired: 2 in, 1 out]
                    n529 = Format Into String(format string=w968, w972) -> (resulting string=w976:string)  [unwired: 2 in, 1 out]
                    n530 = Format Into String(format string=w968, w971) -> (resulting string=w975:string)  [unwired: 2 in, 1 out]
                    n531 = Format Into String(format string=w968, w970) -> (resulting string=w978:string)  [unwired: 2 in, 1 out]
                    n532 = Format Into String(format string="%1.1f", w965) -> (resulting string=w964:string)  [unwired: 2 in, 1 out]
                    n533 = Bundle(w977, w976, w975, w978, w964, w962, w962) -> (w974:T33)  [unwired: 1 out]
                  }
                  frame Default {
                    w981 = "" ("Empty String Constant")
                    n534 = Bundle(w981, w981, w981, w981, w981, w982, w982) -> (w983:T33)  [unwired: 1 out]
                  }
                }
                n535 = Cluster To Array(cluster=w961) -> (array=w960:string[])
                n536 = Build Array(w960) -> (w959:string[][])
              }
              frame #3 {
                # "SAMPLE"
                n537 = local read "Site"() -> (w987:string)
                n538 = case shown="\"SPR1\"" w987 {
                  tunnel: [w990 w1014 w1027] -> w988
                  frame "ICE1", Default {
                    # "PB Req"
                    n539 = control-ref of="Methods"() -> (w991:refnum<vi>)
                    n540 = call "Dropdown Selection (SubVI).vi"("reference"=w991) -> ("element"=w993:string)
                    n541 = Equal?(x=w993, y="V50") -> (x = y?=w992:bool)
                    n542 = local read "totalSampleWt"() -> (w1003:sgl)
                    n543 = case shown="True" w992 {
                      tunnel: ["n/a" w1013] -> w997
                      frame False {
                      }
                      frame True {
                        n544 = local read "minV50"() -> (w1012:i32)
                        n545 = Format Into String(w1012) -> (resulting string=w1013:string)  [unwired: 3 in, 1 out]
                      }
                    }
                    n546 = control-ref of="SampleDimensions"() -> (w1009:refnum<vi>)
                    n547 = control-ref of="SampleCoverings"() -> (w1010:refnum<vi>)
                    n548 = control-ref of="Models"() -> (w996:refnum<vi>)
                    n549 = local read "serialNum"() -> (w1005:string)
                    n550 = local read "SampleID"() -> (w1007:string)
                    n551 = local read "Thickness"() -> (w1000:dbl)
                    n552 = local read "totalBAW"() -> (w999:sgl)
                    n553 = call "Dropdown Selection (SubVI).vi"("reference"=w1009) -> ("element"=w1006:string)
                    n554 = call "Dropdown Selection (SubVI).vi"("reference"=w996) -> ("element"=w995:string)
                    n555 = call "Dropdown Selection (SubVI).vi"("reference"=w1010) -> ("element"=w1004:string)
                    n556 = Format Into String(w1003) -> (resulting string=w1002:string)  [unwired: 3 in, 1 out]
                    n557 = Format Into String(w1000) -> (resulting string=w1001:string)  [unwired: 3 in, 1 out]
                    n558 = Format Into String(w999) -> (resulting string=w998:string)  [unwired: 3 in, 1 out]
                    n559 = Bundle("SampleID"=w1007, "element"=w1006, "Type of work"="Type of work", "serialNum"=w1005, "element"=w995, w1002, w1001, w998, "element"=w1004, w997) -> (w1008:T34)  [unwired: 1 out]
                    n560 = Cluster To Array(cluster=w1008) -> (array=w990:string[])
                  }
                  frame "SPR0" {
                    n561 = local read "totalSampleWt"() -> (w1020:sgl)
                    n562 = control-ref of="SampleDimensions"() -> (w1025:refnum<vi>)
                    n563 = control-ref of="SampleCoverings"() -> (w1026:refnum<vi>)
                    n564 = local read "SampleID"() -> (w1023:string)
                    n565 = local read "Thickness"() -> (w1017:dbl)
                    n566 = local read "totalBAW"() -> (w1016:sgl)
                    n567 = call "Dropdown Selection (SubVI).vi"("reference"=w1025) -> ("element"=w1022:string)
                    n568 = call "Dropdown Selection (SubVI).vi"("reference"=w1026) -> ("element"=w1021:string)
                    n569 = Format Into String(w1020) -> (resulting string=w1019:string)  [unwired: 3 in, 1 out]
                    n570 = Format Into String(w1017) -> (resulting string=w1018:string)  [unwired: 3 in, 1 out]
                    n571 = Format Into String(w1016) -> (resulting string=w1015:string)  [unwired: 3 in, 1 out]
                    n572 = Bundle("SampleID"=w1023, "element"=w1022, w1019, w1018, w1015, "element"=w1021) -> (w1024:T35)  [unwired: 1 out]
                    n573 = Cluster To Array(cluster=w1024) -> (array=w1014:string[])
                  }
                  frame "SPR1" {
                    n574 = local read "totalSampleWt"() -> (w1033:sgl)
                    n575 = control-ref of="SampleDimensions"() -> (w1038:refnum<vi>)
                    n576 = control-ref of="SampleCoverings"() -> (w1039:refnum<vi>)
                    n577 = local read "SampleID"() -> (w1036:string)
                    n578 = local read "Thickness"() -> (w1030:dbl)
                    n579 = local read "totalBAW"() -> (w1029:sgl)
                    n580 = call "Dropdown Selection (SubVI).vi"("reference"=w1038) -> ("element"=w1035:string)
                    n581 = call "Dropdown Selection (SubVI).vi"("reference"=w1039) -> ("element"=w1034:string)
                    n582 = Format Into String(w1033) -> (resulting string=w1032:string)  [unwired: 3 in, 1 out]
                    n583 = Format Into String(w1030) -> (resulting string=w1031:string)  [unwired: 3 in, 1 out]
                    n584 = Format Into String(w1029) -> (resulting string=w1028:string)  [unwired: 3 in, 1 out]
                    n585 = Bundle("SampleID"=w1036, "element"=w1035, w1032, w1031, w1028, "element"=w1034) -> (w1037:T35)  [unwired: 1 out]
                    n586 = Cluster To Array(cluster=w1037) -> (array=w1027:string[])
                  }
                }
              }
              frame #4 {
                n587 = local read "Site"() -> (w1040:string)
                n588 = case shown="\"SPR1\"" w1040 {
                  tunnel: [w1052 w1102 w1154] -> w1042
                  tunnel: w1041 -> [w1045 w1095 w1147]
                  frame "ICE1", Default {
                    # "SHOT TABLE"
                    n589 = control-ref of="Methods"() -> (w1044:refnum<vi>)
                    n590 = call "Dropdown Selection (SubVI).vi"("reference"=w1044) -> ("element"=w1043:string)
                    n591 = for {
                      tunnel: w1045 -> [w1084] mode=indexing
                      shift-right: [w1061] -> _
                      shift-left: T25 [] -> [w1063]
                      tunnel: [w1061] -> w1048
                      tunnel: w1043 -> [w1057]
                      n592 = Unbundle By Name(w1084) -> ("shot order"=w1083:i32, "Powder Loading"=w1082:sgl, "Uncorrected Impact"=w1081:sgl, "UncorrectedRed_PB"=w1080:sgl, "UncorrectedAvgVel_PB"=w1079:sgl, "velLoss_PB"=w1078:sgl, "strikeVel_PB"=w1077:sgl, "SHOT STATUS"=w1066:u16, "usedv50"=w1076:bool, "Shot Angle"=w1058:u16, "BackFace\nDepth"=w1059:sgl)
                      n593 = case shown="\"V50\"" w1057 {
                        tunnel: w1076 -> [w1086 _]
                        tunnel: [w1085 w1090] -> w1075
                        tunnel: w1058 -> [_ w1089]
                        frame "V50" {
                          n594 = case shown="True" w1086 {
                            tunnel: ["" ("Empty String Constant") "*"] -> w1085
                            frame False {
                            }
                            frame True {
                            }
                          }
                        }
                        frame Default {
                          n595 = Format Into String(w1089) -> (resulting string=w1090:string)  [unwired: 3 in, 1 out]
                        }
                      }
                      n596 = case shown="1" w1066 {
                        tunnel: ["P" "C"] -> w1065
                        frame 0, Default {
                        }
                        frame 1 {
                        }
                      }
                      n597 = Format Into String(format string="%2d", w1083) -> (resulting string=w1068:string)  [unwired: 2 in, 1 out]
                      n598 = Format Into String(w1082) -> (resulting string=w1069:string)  [unwired: 3 in, 1 out]
                      n599 = Format Into String(w1081) -> (resulting string=w1070:string)  [unwired: 3 in, 1 out]
                      n600 = Format Into String(w1080) -> (resulting string=w1071:string)  [unwired: 3 in, 1 out]
                      n601 = Format Into String(w1079) -> (resulting string=w1072:string)  [unwired: 3 in, 1 out]
                      n602 = Format Into String(w1078) -> (resulting string=w1073:string)  [unwired: 3 in, 1 out]
                      n603 = Format Into String(w1077) -> (resulting string=w1074:string)  [unwired: 3 in, 1 out]
                      n604 = Format Into String(w1059) -> (resulting string=w1067:string)  [unwired: 3 in, 1 out]
                      n605 = Build Array(w1068, w1069, w1070, w1071, w1072, w1073, w1074, w1065, w1075, w1067) -> (w1062:string[])
                      n606 = Array To Cluster(array=w1062) -> (cluster=w1064:T36)
                      n607 = Build Array (concatenate)(w1063, w1064) -> (w1061:T25)
                    }
                    n608 = Array Size(array=w1048) -> (size(s)=w1050:i32)
                    n609 = Equal To 0?(x=w1050) -> (x = 0?=w1046:bool)
                    n610 = case shown="True" w1046 {
                      tunnel: [w1053 T25 [{"[0]"="", "[1]"="", "[2]"="", "[3]"="", "[4]"="", "[5]"="", "[6]"="", "[7]"="", "[8]"="", "[9]"=""}]] -> w1047
                      tunnel: w1048 -> [w1053 _]
                      frame False {
                      }
                      frame True {
                      }
                    }
                    n611 = Sort 1D Array(array=w1047) -> (sorted array=w1049:T25)
                    n612 = for {
                      tunnel: w1049 -> [w1056] mode=indexing
                      tunnel: [w1055] -> w1052 mode=indexing
                      n613 = Cluster To Array(cluster=w1056) -> (array=w1055:string[])
                    }
                  }
                  frame "SPR0" {
                    # "SHOT TABLE"
                    n614 = control-ref of="Methods"() -> (w1094:refnum<vi>)
                    n615 = call "Dropdown Selection (SubVI).vi"("reference"=w1094) -> ("element"=w1093:string)
                    n616 = for {
                      tunnel: w1095 -> [w1132] mode=indexing
                      shift-right: [w1113] -> _
                      shift-left: T26 [] -> [w1115]
                      tunnel: [w1113] -> w1098
                      tunnel: w1093 -> [w1109]
                      n617 = Unbundle By Name(w1132) -> ("shot order"=w1131:i32, "Powder Loading"=w1130:sgl, "Uncorrected Impact"=w1129:sgl, "UncorrectedRed_PB"=w1128:sgl, "strikeVel_PB"=w1127:sgl, "SHOT STATUS"=w1118:u16, "usedv50"=w1126:bool, "Shot Angle"=w1110:u16, "BackFace\nDepth"=w1111:sgl, "V50userExcl"=w1108:bool, "Shot Description"=w1107:string)
                      n618 = case shown="\"V50\"" w1109 {
                        tunnel: w1126 -> [w1135 _]
                        tunnel: [w1134 w1142] -> w1125
                        tunnel: w1110 -> [_ w1141]
                        tunnel: w1108 -> [w1133 _]
                        frame "V50" {
                          n619 = case shown="True" w1133 {
                            tunnel: w1135 -> [w1137 _]
                            tunnel: [w1136 "!"] -> w1134
                            frame False {
                              n620 = case shown="False" w1137 {
                                tunnel: ["" ("Empty String Constant") "*"] -> w1136
                                frame False {
                                }
                                frame True {
                                }
                              }
                            }
                            frame True {
                            }
                          }
                        }
                        frame Default {
                          n621 = Format Into String(w1141) -> (resulting string=w1142:string)  [unwired: 3 in, 1 out]
                        }
                      }
                      n622 = case shown="1" w1118 {
                        tunnel: ["P" "C"] -> w1117
                        frame 0, Default {
                        }
                        frame 1 {
                        }
                      }
                      n623 = Format Into String(format string="%2d", w1131) -> (resulting string=w1120:string)  [unwired: 2 in, 1 out]
                      n624 = Format Into String(w1130) -> (resulting string=w1121:string)  [unwired: 3 in, 1 out]
                      n625 = Format Into String(w1129) -> (resulting string=w1122:string)  [unwired: 3 in, 1 out]
                      n626 = Format Into String(w1128) -> (resulting string=w1123:string)  [unwired: 3 in, 1 out]
                      n627 = Format Into String(w1127) -> (resulting string=w1124:string)  [unwired: 3 in, 1 out]
                      n628 = Format Into String(w1111) -> (resulting string=w1119:string)  [unwired: 3 in, 1 out]
                      n629 = Build Array(w1120, w1121, w1122, w1123, w1124, w1117, w1125, w1119, w1107) -> (w1114:string[])
                      n630 = Array To Cluster(array=w1114) -> (cluster=w1116:T37)
                      n631 = Build Array (concatenate)(w1115, w1116) -> (w1113:T26)
                    }
                    n632 = Array Size(array=w1098) -> (size(s)=w1100:i32)
                    n633 = Equal To 0?(x=w1100) -> (x = 0?=w1096:bool)
                    n634 = case shown="True" w1096 {
                      tunnel: [w1103 T26 [{"[0]"="", "[1]"="", "[2]"="", "[3]"="", "[4]"="", "[5]"="", "[6]"="", "[7]"="", "[8]"=""}]] -> w1097
                      tunnel: w1098 -> [w1103 _]
                      frame False {
                      }
                      frame True {
                      }
                    }
                    n635 = Sort 1D Array(array=w1097) -> (sorted array=w1099:T26)
                    n636 = for {
                      tunnel: w1099 -> [w1106] mode=indexing
                      tunnel: [w1105] -> w1102 mode=indexing
                      n637 = Cluster To Array(cluster=w1106) -> (array=w1105:string[])
                    }
                  }
                  frame "SPR1" {
                    # "SHOT TABLE"
                    n638 = control-ref of="Methods"() -> (w1146:refnum<vi>)
                    n639 = call "Dropdown Selection (SubVI).vi"("reference"=w1146) -> ("element"=w1145:string)
                    n640 = for {
                      tunnel: w1147 -> [w1184] mode=indexing
                      shift-right: [w1165] -> _
                      shift-left: T26 [] -> [w1167]
                      tunnel: [w1165] -> w1150
                      tunnel: w1145 -> [w1161]
                      n641 = Unbundle By Name(w1184) -> ("shot order"=w1183:i32, "Powder Loading"=w1182:sgl, "Uncorrected Impact"=w1181:sgl, "UncorrectedRed_PB"=w1180:sgl, "strikeVel_PB"=w1179:sgl, "SHOT STATUS"=w1170:u16, "usedv50"=w1178:bool, "Shot Angle"=w1162:u16, "BackFace\nDepth"=w1163:sgl, "V50userExcl"=w1160:bool, "Shot Description"=w1159:string)
                      n642 = case shown="\"V50\"" w1161 {
                        tunnel: w1178 -> [w1187 _]
                        tunnel: [w1186 w1194] -> w1177
                        tunnel: w1162 -> [_ w1193]
                        tunnel: w1160 -> [w1185 _]
                        frame "V50" {
                          n643 = case shown="True" w1185 {
                            tunnel: w1187 -> [w1189 _]
                            tunnel: [w1188 "!"] -> w1186
                            frame False {
                              n644 = case shown="False" w1189 {
                                tunnel: ["" ("Empty String Constant") "*"] -> w1188
                                frame False {
                                }
                                frame True {
                                }
                              }
                            }
                            frame True {
                            }
                          }
                        }
                        frame Default {
                          n645 = Format Into String(w1193) -> (resulting string=w1194:string)  [unwired: 3 in, 1 out]
                        }
                      }
                      n646 = case shown="1" w1170 {
                        tunnel: ["P" "C"] -> w1169
                        frame 0, Default {
                        }
                        frame 1 {
                        }
                      }
                      n647 = Format Into String(format string="%2d", w1183) -> (resulting string=w1172:string)  [unwired: 2 in, 1 out]
                      n648 = Format Into String(w1182) -> (resulting string=w1173:string)  [unwired: 3 in, 1 out]
                      n649 = Format Into String(w1181) -> (resulting string=w1174:string)  [unwired: 3 in, 1 out]
                      n650 = Format Into String(w1180) -> (resulting string=w1175:string)  [unwired: 3 in, 1 out]
                      n651 = Format Into String(w1179) -> (resulting string=w1176:string)  [unwired: 3 in, 1 out]
                      n652 = Format Into String(w1163) -> (resulting string=w1171:string)  [unwired: 3 in, 1 out]
                      n653 = Build Array(w1172, w1173, w1174, w1175, w1176, w1169, w1177, w1171, w1159) -> (w1166:string[])
                      n654 = Array To Cluster(array=w1166) -> (cluster=w1168:T37)
                      n655 = Build Array (concatenate)(w1167, w1168) -> (w1165:T26)
                    }
                    n656 = Array Size(array=w1150) -> (size(s)=w1152:i32)
                    n657 = Equal To 0?(x=w1152) -> (x = 0?=w1148:bool)
                    n658 = case shown="True" w1148 {
                      tunnel: [w1155 T26 [{"[0]"="", "[1]"="", "[2]"="", "[3]"="", "[4]"="", "[5]"="", "[6]"="", "[7]"="", "[8]"=""}]] -> w1149
                      tunnel: w1150 -> [w1155 _]
                      frame False {
                      }
                      frame True {
                      }
                    }
                    n659 = Sort 1D Array(array=w1149) -> (sorted array=w1151:T26)
                    n660 = for {
                      tunnel: w1151 -> [w1158] mode=indexing
                      tunnel: [w1157] -> w1154 mode=indexing
                      n661 = Cluster To Array(cluster=w1158) -> (array=w1157:string[])
                    }
                  }
                }
              }
              frame #5 {
                n662 = local read "Site"() -> (w1197:string)
                n663 = case shown="\"SPR1\"" w1197 {
                  tunnel: [w1228 w1249 w1269] -> w1204
                  tunnel: [w1227 w1248 w1268] -> w1203
                  tunnel: [w1226 w1247 w1267] -> w1202
                  tunnel: [w1225 w1232 w1252] -> w1201
                  tunnel: ["" ("projNum") w1232 w1252] -> w1200
                  tunnel: [w1223 w1246 w1266] -> w1199
                  tunnel: [w1207 w1235 w1255] -> w1198
                  frame "ICE1", Default {
                    # "THREAT"
                    # "Range # (supports a PB reporting requirement)"
                    # "Project Name goes here.\nSupports a PB reporting requirement."
                    # "GENERAL"
                    n664 = local read "threatDetails"() -> (w1206:T1)
                    n665 = Unbundle By Name(w1206) -> ("barrelLength"=w1210:string)
                    n666 = Unbundle By Name(w1206) -> ("grainSize"=w1205:string)
                    n667 = local read "Shot Angle"() -> (w1211:u16)
                    n668 = control-ref of="WeaponTypes"() -> (w1220:refnum<vi>)
                    n669 = control-ref of="ThreatGroups"() -> (w1219:refnum<vi>)
                    n670 = control-ref of="PowderTypes"() -> (w1218:refnum<vi>)
                    n671 = control-ref of="Recorders"() -> (w1221:refnum<vi>)
                    n672 = control-ref of="Shooters"() -> (w1222:refnum<vi>)
                    n673 = Format Into String(w1211) -> (resulting string=w1212:string)  [unwired: 3 in, 1 out]
                    n674 = call "Dropdown Selection (SubVI).vi"("reference"=w1220) -> ("element"=w1216:string)
                    n675 = call "Dropdown Selection (SubVI).vi"("reference"=w1219) -> ("element"=w1215:string)
                    n676 = call "Dropdown Selection (SubVI).vi"("reference"=w1218) -> ("element"=w1214:string)
                    n677 = call "Dropdown Selection (SubVI).vi"("reference"=w1221) -> ("element"=w1213:string)
                    n678 = call "Dropdown Selection (SubVI).vi"("reference"=w1222) -> ("element"=w1209:string)
                    n679 = local read "Comments"() -> (w1226:string)
                    n680 = local read "ProjectID"() -> (w1223:string)
                    n681 = Bundle("element"=w1216, "element"=w1215, "grainSize"=w1205, "element"=w1214, "barrelLength"=w1210, w1212, "element"="1", "element"=w1209, "element"=w1213) -> (w1217:T38)  [unwired: 1 out]
                    n682 = local read "lastSamp"() -> (w1231:i32)
                    n683 = control-ref of="TestStandards"() -> (w1230:refnum<vi>)
                    n684 = control-ref of="Methods"() -> (w1229:refnum<vi>)
                    n685 = Cluster To Array(cluster=w1217) -> (array=w1207:string[])
                    n686 = call "Dropdown Selection (SubVI).vi"("reference"=w1230) -> ("element"=w1225:string)
                    n687 = call "Dropdown Selection (SubVI).vi"("reference"=w1229) -> ("element"=w1228:string)
                    n688 = Increment(x=w1231) -> (x+1=w1227:i32)
                  }
                  frame "SPR0" {
                    w1232 = "" ("projNum")
                    # "THREAT"
                    # "Project Name goes here.\nSupports a PB reporting requirement."
                    # "GENERAL"
                    n689 = local read "threatDetails"() -> (w1234:T1)
                    n690 = Unbundle By Name(w1234) -> ("barrelLength"=w1237:string)
                    n691 = Unbundle By Name(w1234) -> ("grainSize"=w1233:string)
                    n692 = local read "Shot Angle"() -> (w1238:u16)
                    n693 = control-ref of="ThreatGroups"() -> (w1244:refnum<vi>)
                    n694 = control-ref of="PowderTypes"() -> (w1243:refnum<vi>)
                    n695 = control-ref of="Ballisticians"() -> (w1245:refnum<vi>)
                    n696 = Format Into String(w1238) -> (resulting string=w1239:string)  [unwired: 3 in, 1 out]
                    n697 = call "Dropdown Selection (SubVI).vi"("reference"=w1244) -> ("element"=w1241:string)
                    n698 = call "Dropdown Selection (SubVI).vi"("reference"=w1243) -> ("element"=w1240:string)
                    n699 = call "Dropdown Selection (SubVI).vi"("reference"=w1245) -> ("element"=w1236:string)
                    n700 = local read "Comments"() -> (w1247:string)
                    n701 = local read "ProjectID"() -> (w1246:string)
                    n702 = Bundle("element"=w1241, "grainSize"=w1233, "element"=w1240, "barrelLength"=w1237, w1239, "element"=w1236) -> (w1242:T39)  [unwired: 1 out]
                    n703 = local read "lastSamp"() -> (w1251:i32)
                    n704 = control-ref of="Methods"() -> (w1250:refnum<vi>)
                    n705 = Cluster To Array(cluster=w1242) -> (array=w1235:string[])
                    n706 = call "Dropdown Selection (SubVI).vi"("reference"=w1250) -> ("element"=w1249:string)
                    n707 = Increment(x=w1251) -> (x+1=w1248:i32)
                  }
                  frame "SPR1" {
                    w1252 = "" ("projNum")
                    # "THREAT"
                    # "Project Name goes here.\nSupports a PB reporting requirement."
                    # "GENERAL"
                    n708 = local read "threatDetails"() -> (w1254:T1)
                    n709 = Unbundle By Name(w1254) -> ("barrelLength"=w1257:string)
                    n710 = Unbundle By Name(w1254) -> ("grainSize"=w1253:string)
                    n711 = local read "Shot Angle"() -> (w1258:u16)
                    n712 = control-ref of="Ballisticians"() -> (w1265:refnum<vi>)
                    n713 = control-ref of="ThreatGroups"() -> (w1264:refnum<vi>)
                    n714 = control-ref of="PowderTypes"() -> (w1263:refnum<vi>)
                    n715 = call "Dropdown Selection (SubVI).vi"("reference"=w1265) -> ("element"=w1256:string)
                    n716 = call "Dropdown Selection (SubVI).vi"("reference"=w1264) -> ("element"=w1261:string)
                    n717 = call "Dropdown Selection (SubVI).vi"("reference"=w1263) -> ("element"=w1260:string)
                    n718 = Format Into String(w1258) -> (resulting string=w1259:string)  [unwired: 3 in, 1 out]
                    n719 = control-ref of="Methods"() -> (w1270:refnum<vi>)
                    n720 = local read "Comments"() -> (w1267:string)
                    n721 = local read "lastSamp"() -> (w1271:i32)
                    n722 = local read "ProjectID"() -> (w1266:string)
                    n723 = Bundle("element"=w1261, "grainSize"=w1253, "element"=w1260, "barrelLength"=w1257, w1259, "element"=w1256) -> (w1262:T39)  [unwired: 1 out]
                    n724 = call "Dropdown Selection (SubVI).vi"("reference"=w1270) -> ("element"=w1269:string)
                    n725 = Cluster To Array(cluster=w1262) -> (array=w1255:string[])
                    n726 = Increment(x=w1271) -> (x+1=w1268:i32)
                  }
                }
              }
            }
            n727 = Get Date/Time String() -> (date string=w854:string)  [unwired: 3 in, 1 out]
          }
          frame True {
            w1287 = ""
            w1279 = 16  # dimensions
            w1282 = 5  # SampleID
            # "date"
            # "method"
            # "general"
            # "remark"
            # "threat"
            # "shots"
            # "sample"
            # "results"
            # "range"
            # "fabric"
            # "query db with the entered record number and use result to populate the xlt"
            n728 = Not(x=w1345) -> (.not. x?=w1344:bool)
            n729 = local write "lookupRec"(w1344) -> ()
            n730 = Format Into String(format string="SELECT * FROM Experiments\nWHERE expt=%d;" ("query string"), error in=w1311, "Record #") -> (resulting string=w1341:string, error out=w1312:errorcluster)  [unwired: 1 in]
            n731 = call "Fetch Data (SubVI).vi"("error IN"=w1312, "query string"=w1341) -> ("error OUT"=w1310:errorcluster, "recordset data"=w1343:string[][])  [unwired: 4 out]
            n732 = Index Array(array=w1343) -> (element=w1281:string[])  [unwired: 2 in]
            n733 = Index Array(array=w1281, index=111) -> (element=w1314:string)
            n734 = local read "Set#1 Separation"() -> (w1328:sgl)
            n735 = call "Load Shots (SubVI).vi"("Record #"="Record #", "Method"=w1314) -> ("Shot Array"=w1336:string[][], "AvgDef"=w1319:dbl)  [unwired: 1 in]
            n736 = local read "mid_to_targ_dist"() -> (w1331:sgl)
            n737 = local read "Barrel to Screen"() -> (w1334:sgl)
            n738 = Format Into String(w1319) -> (resulting string=w1317:string)  [unwired: 3 in, 1 out]
            n739 = Match Pattern(string=w1314, regular expression="N.I.J.") -> (offset past match=w1316:i32)  [unwired: 4 out]
            n740 = Greater Or Equal To 0?(x=w1316) -> (x >= 0?=w1313:bool)
            n741 = case shown="False" w1313 {
              tunnel: [w1356 w1357] -> w1318
              tunnel: w1317 -> [w1353 w1359]
              tunnel: w1281 -> [w1355 _]
              frame False {
                n742 = Index Array(array=w1355, index #1=124 ("index"), index #2=149 ("index"), index #5=145 ("index")) -> (element #1=w1354:string, element #2=w1352:string, element #3=w1351:string, element #4=w1347:string, element #5=w1348:string)  [unwired: 2 in]
                n743 = Build Array(w1354, w1352, w1351, w1347, w1348, w1353) -> (w1356:string[])
              }
              frame True {
                w1358 = "" ("Empty String Constant")
                n744 = Build Array(w1358, w1358, w1358, w1358, w1358, w1359, w1359) -> (w1357:string[])
              }
            }
            n745 = Divide(x=w1328, y=sgl 2.0) -> (x/y=w1333:sgl)
            n746 = Add(x=w1334, y=w1331) -> (x+y=w1327:sgl)
            n747 = Subtract(x=w1334, y=w1333) -> (x-y=w1332:sgl)
            n748 = Subtract(x=w1331, y=w1333) -> (x-y=w1330:sgl)
            n749 = Index Array(array=w1281, index #1=120 ("index"), index #2=119 ("index"), index #3=127 ("index"), index #4=12 ("index"), index #5=7 ("index")) -> (element #1=w1299:string, element #2=w1297:string, element #3=w1296:string, element #4=w1293:string, element #5=w1292:string)
            n750 = Index Array(array=w1281, index #1=113 ("index"), index #2=112 ("index"), index #3=103 ("index")) -> (element #1=w1308:string, element #2=w1307:string, element #3=w1306:string, element #4=w1305:string, element #5=w1301:string)  [unwired: 2 in]
            n751 = Format Into String(w1327) -> (resulting string=w1326:string)  [unwired: 3 in, 1 out]
            n752 = Format Into String(w1332) -> (resulting string=w1325:string)  [unwired: 3 in, 1 out]
            n753 = Format Into String(w1328) -> (resulting string=w1324:string)  [unwired: 3 in, 1 out]
            n754 = Format Into String(w1330) -> (resulting string=w1323:string)  [unwired: 3 in, 1 out]
            n755 = Format Into String(w1331) -> (resulting string=w1322:string)  [unwired: 3 in, 1 out]
            n756 = Index Array(array=w1281, index #1=w1282, index #2=w1279, index #3=147 ("index"), index #5=148 ("index")) -> (element #1=w1280:string, element #2=w1277:string, element #3=w1276:string, element #5=w1273:string)  [unwired: 1 in, 1 out]
            n757 = Build Array(w1299, w1297, w1296, "", w1293, w1292) -> (w1298:string[])
            n758 = Build Array(w1326, w1325, w1324, w1323, w1322, w1308, w1307, w1306, w1305, w1301) -> (w1321:string[])
            n759 = Index Array(array=w1281, index #1=4 ("index"), index #2=111 ("index")) -> (element #1=w1288:string, element #2=w1285:string)
            n760 = Index Array(array=w1281, index=107) -> (element=w1337:string)
            n761 = Build Array(w1280, w1277, w1276, "", w1273) -> (w1278:string[])
            n762 = Index Array(array=w1281, index=2) -> (element=w1283:string)
            n763 = call "Get Model Construction.vi"("panel record"=w1281) -> ("Fabric Array"=w1335:string[][])
            n764 = Build Array(w1318) -> (w1338:string[][])
          }
        }
        n765 = To Variant(anything=w849) -> (Variant=w843:variant)
        n766 = To Variant(anything=w848) -> (Variant=w842:variant)
        n767 = To Variant(anything=w847) -> (Variant=w841:variant)
        n768 = To Variant(anything=w846) -> (Variant=w840:variant)
        n769 = To Variant(anything=w845) -> (Variant=w839:variant)
        n770 = To Variant(anything=w844) -> (Variant=w838:variant)
        n771 = To Variant(anything=w831) -> (Variant=w837:variant)
        n772 = To Variant(anything=w830) -> (Variant=w836:variant)
        n773 = To Variant(anything=w829) -> (Variant=w835:variant)
        n774 = To Variant(anything=w828) -> (Variant=w832:variant)
        n775 = To Variant(anything=w827) -> (Variant=w833:variant)
        n776 = To Variant(anything=w820) -> (Variant=w834:variant)
        n777 = To Variant(anything=w818) -> (Variant=w819:variant)
        n778 = call "TestReport_XL.vi"("Enable"=TRUE, "blockFabric"=w843, "blockRange"=w842, "blockResults"=w841, "blockSample"=w840, "blockShotTbl"=w839, "error in (no error)"=w823, "blockThreat"=w838, "testDate"=w819, "method"=w837, "projName"=w836, "projNum"=w835, "recNum"=w832, "remark"=w833, "standard"=w834) -> ("error out"=w850:errorcluster)  [unwired: 4 in, 8 out]
        n779 = call <vilib>:"Simple Error Handler.vi"("error in (no error)"=w850) -> ("error out"=w852:errorcluster)  [unwired: 1 in, 7 out]
        n780 = case shown="No Error" w852 {
          selector: w852 -> [w1360 w1362]
          tunnel: [w1360 w1362] -> w821
          frame No Error {
            n781 = One Button Dialog(message=" V50 Ballistic Test Report is ready") -> ()  [unwired: 2 out]
          }
          frame Error {
          }
        }
      }
      frame "VsVr Report" {
        w1392 = TRUE  # Enable
        # "case # 3"
        # "The custom Excel template file is \nexpected in the C:\\Ballistics folder."
        n782 = stacked-sequence {
          tunnel: [_ _ _ _ _ w1583] -> w1385
          tunnel: [_ w1456 _ _ _ _] -> w1389
          tunnel: [_ _ _ _ w1540 _] -> w1386
          tunnel: [_ _ _ w1507 _ _] -> w1387
          tunnel: [_ _ w1478 _ _ _] -> w1388
          tunnel: [w1400 _ _ _ _ _] -> w1390
          tunnel: [_ _ _ _ _ w1604] -> w1372
          tunnel: [_ _ _ _ _ "" ("projNum")] -> w1371
          tunnel: [_ _ _ _ _ w1599] -> w1370
          tunnel: [_ _ _ _ _ w1603] -> w1369
          tunnel: [_ _ _ _ _ w1602] -> w1368
          tunnel: [_ _ _ _ _ w1601] -> w1367
          tunnel: w1366 -> [_ _ w1477 _ w1533 _]
          frame #0 {
            # "FABRIC"
            n783 = local read "fab1_totalWt"() -> (w1403:sgl)
            n784 = local read "fab3_totalWt"() -> (w1405:sgl)
            n785 = local read "fab5_totalWt"() -> (w1407:sgl)
            n786 = global read "BIMS_Collector Globals.vi" "LayerStitchTypeRefs"() -> (w1395:refnum<vi>[])
            n787 = global read "BIMS_Collector Globals.vi" "SampleAttribs"() -> (w1396:T21)
            n788 = global read "BIMS_Collector Globals.vi" "SampleStyles"() -> (w1398:refnum<vi>[])
            n789 = local read "fab2_totalWt"() -> (w1404:sgl)
            n790 = local read "fab4_totalWt"() -> (w1406:sgl)
            n791 = local read "fab6_totalWt"() -> (w1408:sgl)
            n792 = global read "BIMS_Collector Globals.vi" "LayerSpecs"() -> (w1397:T31)
            n793 = global read "BIMS_Collector Globals.vi" "Mfrs"() -> (w1399:refnum<vi>[])
            n794 = Build Array(w1403, w1404, w1405, w1406, w1407, w1408) -> (w1402:sgl[])
            n795 = for {
              tunnel: w1402 -> [w1410] mode=indexing
              tunnel: [w1416] -> w1401 mode=indexing
              tunnel: w1396 -> [w1414] mode=indexing
              tunnel: w1397 -> [w1413] mode=indexing
              tunnel: w1399 -> [w1412] mode=indexing
              tunnel: w1398 -> [w1411] mode=indexing
              tunnel: w1395 -> [w1409] mode=indexing
              n796 = Less Or Equal To 0?(x=w1410) -> (x <= 0?=w1415:bool)
              n797 = case shown="False" w1415 {
                tunnel: [w1438 w1440] -> w1416
                tunnel: w1414 -> [w1437 _]
                tunnel: w1413 -> [w1422 _]
                tunnel: w1412 -> [w1431 _]
                tunnel: w1411 -> [w1428 _]
                tunnel: w1410 -> [w1421 _]
                tunnel: w1409 -> [w1417 _]
                frame False {
                  n798 = Unbundle By Name(w1422) -> ("numOfPlies"=w1420:i32, "LotNum"=w1434:string, "RollNum"=w1435:string)
                  n799 = Unbundle By Name(w1437) -> ("internal_ID"=w1425:string, "fiber"=w1426:string, "denier"=w1433:string, "pick"=w1432:string, "weave"=w1423:string, "finish"=w1424:string, "ozPerYd2"=w1436:string)
                  n800 = Format Into String(w1420) -> (resulting string=w1430:string)  [unwired: 3 in, 1 out]
                  n801 = call "Dropdown Selection (SubVI).vi"("reference"=w1431) -> ("element"=w1429:string)
                  n802 = call "Dropdown Selection (SubVI).vi"("reference"=w1428) -> ("element"=w1427:string)
                  n803 = call "Dropdown Selection (SubVI).vi"("reference"=w1417) -> ("element"=w1418:string)
                  n804 = Format Into String(w1421) -> (resulting string=w1419:string)  [unwired: 3 in, 1 out]
                  n805 = Build Array(w1430, w1429, w1427, w1425, w1426, w1433, w1432, w1423, w1424, w1434, w1435, w1436, w1419, w1418) -> (w1438:string[])
                }
                frame True {
                  n806 = call <vilib>:"Space Constant.vi"() -> ("String"=w1441:string)
                  n807 = Initialize Array(w1441, 12 ("dimension size")) -> (w1440:string[])
                }
              }
            }
            n808 = Transpose 2D Array(2D array=w1401) -> (transposed array=w1400:string[][])
          }
          frame #1 {
            w1442 = "%.1f" ("format string")
            # "muzzel / midpoint"
            # "muzzle / scr#1"
            # "muzzle / target"
            # "scr#2 / target"
            # "RANGE"
            n809 = local read "Set#1 Separation"() -> (w1449:sgl)
            n810 = local read "mid_to_targ_dist"() -> (w1446:sgl)
            n811 = local read "Barrel to Screen"() -> (w1443:sgl)
            n812 = local read "clayAverage"() -> (w1464:sgl)
            n813 = Divide(x=w1449, y=sgl 2.0) -> (x/y=w1444:sgl)
            n814 = local read "RoomHum"() -> (w1459:sgl)
            n815 = local read "clayTemp"() -> (w1462:sgl)
            n816 = local read "clayCalib"() -> (w1465:string)
            n817 = local read "RoomT"() -> (w1460:sgl)
            n818 = Add(x=w1443, y=w1446) -> (x+y=w1450:sgl)
            n819 = Subtract(x=w1443, y=w1444) -> (x-y=w1445:sgl)
            n820 = Subtract(x=w1446, y=w1444) -> (x-y=w1447:sgl)
            n821 = Format Into String(w1450) -> (resulting string=w1451:string)  [unwired: 3 in, 1 out]
            n822 = Format Into String(w1445) -> (resulting string=w1452:string)  [unwired: 3 in, 1 out]
            n823 = Format Into String(w1449) -> (resulting string=w1453:string)  [unwired: 3 in, 1 out]
            n824 = Format Into String(w1447) -> (resulting string=w1454:string)  [unwired: 3 in, 1 out]
            n825 = Format Into String(w1446) -> (resulting string=w1455:string)  [unwired: 3 in, 1 out]
            n826 = Format Into String(w1459) -> (resulting string=w1457:string)  [unwired: 3 in, 1 out]
            n827 = Format Into String(format string=w1442, w1460) -> (resulting string=w1458:string)  [unwired: 2 in, 1 out]
            n828 = Format Into String(format string=w1442, w1462) -> (resulting string=w1461:string)  [unwired: 2 in, 1 out]
            n829 = Format Into String(format string=w1442, w1464) -> (resulting string=w1463:string)  [unwired: 2 in, 1 out]
            n830 = Bundle(w1451, w1452, w1453, w1454, w1455, w1457, w1458, w1461, "clayCalib"=w1465, w1463) -> (w1466:T32)  [unwired: 1 out]
            n831 = Cluster To Array(cluster=w1466) -> (array=w1456:string[])
          }
          frame #2 {
            # "RESULTS"
            n832 = control-ref of="Methods"() -> (w1467:refnum<vi>)
            n833 = call "Dropdown Selection (SubVI).vi"("reference"=w1467) -> ("element"=w1468:string)
            n834 = for {
              tunnel: w1477 -> [w1505] mode=indexing
              tunnel: [w1504] -> w1476 mode=indexing
              tunnel: [w1503] -> w1475
              i -> [w1503]
              n835 = Unbundle By Name(w1505) -> ("BackFace\nDepth"=w1504:sgl)
            }
            n836 = Increment(x=w1475) -> (x+1=w1473:i32)
            n837 = Add Array Elements(numeric array=w1476) -> (sum=w1474:sgl)
            n838 = To Single Precision Float(number=w1473) -> (single precision float=w1472:sgl)
            n839 = Divide(x=w1474, y=w1472) -> (x/y=w1471:sgl)
            n840 = Format Into String(format string="%1.1f", w1471) -> (resulting string=w1470:string)  [unwired: 2 in, 1 out]
            n841 = case shown="\"V50\"" w1468 {
              tunnel: [w1493 w1502] -> w1480
              tunnel: w1470 -> [w1481 w1501]
              frame "V50" {
                w1487 = "%1d" ("format string")
                n842 = local read "Z.M.R."() -> (w1485:sgl)
                n843 = Less Than 0?(x=w1485) -> (x < 0?=w1486:bool)
                n844 = local read "rangeOfResults"() -> (w1489:i32)
                n845 = local read "computed_V50"() -> (w1492:sgl)
                n846 = local read "lowComplete"() -> (w1490:i32)
                n847 = local read "highPartial"() -> (w1491:i32)
                n848 = case shown="True" w1486 {
                  tunnel: w1485 -> [w1498 _]
                  tunnel: [w1498 sgl 0.0 ("Z.M.R.")] -> w1484
                  frame False {
                  }
                  frame True {
                  }
                }
                n849 = Format Into String(format string="%1.1f", w1492) -> (resulting string=w1496:string)  [unwired: 2 in, 1 out]
                n850 = Format Into String(format string=w1487, w1491) -> (resulting string=w1495:string)  [unwired: 2 in, 1 out]
                n851 = Format Into String(format string=w1487, w1490) -> (resulting string=w1494:string)  [unwired: 2 in, 1 out]
                n852 = Format Into String(format string=w1487, w1489) -> (resulting string=w1497:string)  [unwired: 2 in, 1 out]
                n853 = Format Into String(format string="%1.1f", w1484) -> (resulting string=w1483:string)  [unwired: 2 in, 1 out]
                n854 = Bundle(w1496, w1495, w1494, w1497, w1483, w1481, w1481) -> (w1493:T33)  [unwired: 1 out]
              }
              frame Default {
                w1500 = "" ("Empty String Constant")
                n855 = Bundle(w1500, w1500, w1500, w1500, w1500, w1501, w1501) -> (w1502:T33)  [unwired: 1 out]
              }
            }
            n856 = Cluster To Array(cluster=w1480) -> (array=w1479:string[])
            n857 = Build Array(w1479) -> (w1478:string[][])
          }
          frame #3 {
            # "PB Req"
            # "SAMPLE"
            n858 = control-ref of="Methods"() -> (w1508:refnum<vi>)
            n859 = call "Dropdown Selection (SubVI).vi"("reference"=w1508) -> ("element"=w1510:string)
            n860 = Equal?(x=w1510, y="V50") -> (x = y?=w1509:bool)
            n861 = local read "totalSampleWt"() -> (w1520:sgl)
            n862 = case shown="True" w1509 {
              tunnel: ["n/a" w1530] -> w1514
              frame False {
              }
              frame True {
                n863 = local read "minV50"() -> (w1529:i32)
                n864 = Format Into String(w1529) -> (resulting string=w1530:string)  [unwired: 3 in, 1 out]
              }
            }
            n865 = local read "Type of work"() -> (w1506:string)
            n866 = control-ref of="SampleDimensions"() -> (w1526:refnum<vi>)
            n867 = control-ref of="SampleCoverings"() -> (w1527:refnum<vi>)
            n868 = control-ref of="Models"() -> (w1513:refnum<vi>)
            n869 = local read "serialNum"() -> (w1522:string)
            n870 = local read "SampleID"() -> (w1524:string)
            n871 = local read "Thickness"() -> (w1517:dbl)
            n872 = local read "totalBAW"() -> (w1516:sgl)
            n873 = call "Dropdown Selection (SubVI).vi"("reference"=w1526) -> ("element"=w1523:string)
            n874 = call "Dropdown Selection (SubVI).vi"("reference"=w1513) -> ("element"=w1512:string)
            n875 = call "Dropdown Selection (SubVI).vi"("reference"=w1527) -> ("element"=w1521:string)
            n876 = Format Into String(w1520) -> (resulting string=w1519:string)  [unwired: 3 in, 1 out]
            n877 = Format Into String(w1517) -> (resulting string=w1518:string)  [unwired: 3 in, 1 out]
            n878 = Format Into String(w1516) -> (resulting string=w1515:string)  [unwired: 3 in, 1 out]
            n879 = Bundle("SampleID"=w1524, "element"=w1523, "Type of work"=w1506, "serialNum"=w1522, "element"=w1512, w1519, w1518, w1515, "element"=w1521, w1514) -> (w1525:T34)  [unwired: 1 out]
            n880 = Cluster To Array(cluster=w1525) -> (array=w1507:string[])
          }
          frame #4 {
            # "SHOT TABLE"
            n881 = control-ref of="Methods"() -> (w1532:refnum<vi>)
            n882 = call "Dropdown Selection (SubVI).vi"("reference"=w1532) -> ("element"=w1531:string)
            n883 = for {
              tunnel: w1533 -> [w1572] mode=indexing
              shift-right: [w1549] -> _
              shift-left: T25 [] -> [w1551]
              tunnel: [w1549] -> w1536
              tunnel: w1531 -> [w1545]
              n884 = Unbundle By Name(w1572) -> ("shot order"=w1571:i32, "Powder Loading"=w1570:sgl, "Uncorrected Impact"=w1569:sgl, "UncorrectedRed_PB"=w1568:sgl, "UncorrectedAvgVel_PB"=w1567:sgl, "velLoss_PB"=w1566:sgl, "strikeVel_PB"=w1565:sgl, "SHOT STATUS"=w1554:u16, "usedv50"=w1564:bool, "Shot Angle"=w1546:u16, "BackFace\nDepth"=w1547:sgl)
              n885 = case shown="\"V50\"" w1545 {
                tunnel: w1564 -> [w1574 _]
                tunnel: [w1573 w1578] -> w1563
                tunnel: w1546 -> [_ w1577]
                frame "V50" {
                  n886 = case shown="True" w1574 {
                    tunnel: ["" ("Empty String Constant") "*"] -> w1573
                    frame False {
                    }
                    frame True {
                    }
                  }
                }
                frame Default {
                  n887 = Format Into String(w1577) -> (resulting string=w1578:string)  [unwired: 3 in, 1 out]
                }
              }
              n888 = case shown="1" w1554 {
                tunnel: ["P" "C"] -> w1553
                frame 0, Default {
                }
                frame 1 {
                }
              }
              n889 = Format Into String(format string="%2d", w1571) -> (resulting string=w1556:string)  [unwired: 2 in, 1 out]
              n890 = Format Into String(w1570) -> (resulting string=w1557:string)  [unwired: 3 in, 1 out]
              n891 = Format Into String(w1569) -> (resulting string=w1558:string)  [unwired: 3 in, 1 out]
              n892 = Format Into String(w1568) -> (resulting string=w1559:string)  [unwired: 3 in, 1 out]
              n893 = Format Into String(w1567) -> (resulting string=w1560:string)  [unwired: 3 in, 1 out]
              n894 = Format Into String(w1566) -> (resulting string=w1561:string)  [unwired: 3 in, 1 out]
              n895 = Format Into String(w1565) -> (resulting string=w1562:string)  [unwired: 3 in, 1 out]
              n896 = Format Into String(w1547) -> (resulting string=w1555:string)  [unwired: 3 in, 1 out]
              n897 = Build Array(w1556, w1557, w1558, w1559, w1560, w1561, w1562, w1553, w1563, w1555) -> (w1550:string[])
              n898 = Array To Cluster(array=w1550) -> (cluster=w1552:T36)
              n899 = Build Array (concatenate)(w1551, w1552) -> (w1549:T25)
            }
            n900 = Array Size(array=w1536) -> (size(s)=w1538:i32)
            n901 = Equal To 0?(x=w1538) -> (x = 0?=w1534:bool)
            n902 = case shown="True" w1534 {
              tunnel: [w1541 T25 [{"[0]"="", "[1]"="", "[2]"="", "[3]"="", "[4]"="", "[5]"="", "[6]"="", "[7]"="", "[8]"="", "[9]"=""}]] -> w1535
              tunnel: w1536 -> [w1541 _]
              frame False {
              }
              frame True {
              }
            }
            n903 = Sort 1D Array(array=w1535) -> (sorted array=w1537:T25)
            n904 = for {
              tunnel: w1537 -> [w1544] mode=indexing
              tunnel: [w1543] -> w1540 mode=indexing
              n905 = Cluster To Array(cluster=w1544) -> (array=w1543:string[])
            }
          }
          frame #5 {
            # "THREAT"
            # "Range # (supports a PB reporting requirement)"
            # "Project Name goes here.\nSupports a PB reporting requirement."
            # "GENERAL"
            n906 = local read "threatDetails"() -> (w1582:T1)
            n907 = Unbundle By Name(w1582) -> ("barrelLength"=w1586:string)
            n908 = Unbundle By Name(w1582) -> ("grainSize"=w1581:string)
            n909 = local read "Shot Angle"() -> (w1587:u16)
            n910 = control-ref of="WeaponTypes"() -> (w1596:refnum<vi>)
            n911 = control-ref of="ThreatGroups"() -> (w1595:refnum<vi>)
            n912 = control-ref of="PowderTypes"() -> (w1594:refnum<vi>)
            n913 = control-ref of="Recorders"() -> (w1597:refnum<vi>)
            n914 = control-ref of="Shooters"() -> (w1598:refnum<vi>)
            n915 = Format Into String(w1587) -> (resulting string=w1588:string)  [unwired: 3 in, 1 out]
            n916 = call "Dropdown Selection (SubVI).vi"("reference"=w1596) -> ("element"=w1592:string)
            n917 = call "Dropdown Selection (SubVI).vi"("reference"=w1595) -> ("element"=w1591:string)
            n918 = call "Dropdown Selection (SubVI).vi"("reference"=w1594) -> ("element"=w1590:string)
            n919 = call "Dropdown Selection (SubVI).vi"("reference"=w1597) -> ("element"=w1589:string)
            n920 = call "Dropdown Selection (SubVI).vi"("reference"=w1598) -> ("element"=w1585:string)
            n921 = Bundle("element"=w1592, "element"=w1591, "grainSize"=w1581, "element"=w1590, "barrelLength"=w1586, w1588, "element"="1", "element"=w1585, "element"=w1589) -> (w1593:T38)  [unwired: 1 out]
            n922 = Cluster To Array(cluster=w1593) -> (array=w1583:string[])
            n923 = local read "Comments"() -> (w1602:string)
            n924 = local read "ProjectID"() -> (w1599:string)
            n925 = local read "lastSamp"() -> (w1607:i32)
            n926 = control-ref of="TestStandards"() -> (w1606:refnum<vi>)
            n927 = control-ref of="Methods"() -> (w1605:refnum<vi>)
            n928 = call "Dropdown Selection (SubVI).vi"("reference"=w1606) -> ("element"=w1601:string)
            n929 = call "Dropdown Selection (SubVI).vi"("reference"=w1605) -> ("element"=w1604:string)
            n930 = Increment(x=w1607) -> (x+1=w1603:i32)
          }
        }
        n931 = To Variant(anything=w1390) -> (Variant=w1384:variant)
        n932 = To Variant(anything=w1389) -> (Variant=w1383:variant)
        n933 = To Variant(anything=w1388) -> (Variant=w1382:variant)
        n934 = To Variant(anything=w1387) -> (Variant=w1381:variant)
        n935 = To Variant(anything=w1386) -> (Variant=w1380:variant)
        n936 = To Variant(anything=w1385) -> (Variant=w1379:variant)
        n937 = To Variant(anything=w1372) -> (Variant=w1378:variant)
        n938 = To Variant(anything=w1371) -> (Variant=w1377:variant)
        n939 = To Variant(anything=w1370) -> (Variant=w1376:variant)
        n940 = To Variant(anything=w1369) -> (Variant=w1373:variant)
        n941 = To Variant(anything=w1368) -> (Variant=w1374:variant)
        n942 = To Variant(anything=w1367) -> (Variant=w1375:variant)
        n943 = call "TestReport_XL.vi"("Enable"=w1392, "blockFabric"=w1384, "blockRange"=w1383, "blockResults"=w1382, "blockSample"=w1381, "blockShotTbl"=w1380, "error in (no error)"=w1364, "blockThreat"=w1379, "method"=w1378, "projName"=w1377, "projNum"=w1376, "recNum"=w1373, "remark"=w1374, "standard"=w1375) -> ("error out"=w1391:errorcluster)  [unwired: 5 in, 8 out]
        n944 = call <vilib>:"Simple Error Handler.vi"("error in (no error)"=w1391) -> ("error out"=w1393:errorcluster)  [unwired: 1 in, 7 out]
        n945 = case shown="No Error" w1393 {
          selector: w1393 -> [w1608 w1610]
          tunnel: [w1608 w1610] -> w1363
          frame No Error {
            n946 = One Button Dialog(message=" VsVr Ballistic Test Report is ready") -> ()  [unwired: 2 out]
          }
          frame Error {
          }
        }
      }
      frame "SAVE SHOTS" {
        # "case # 4"
        # "This section saves the shots to the data base"
        n947 = stacked-sequence {
          seq-local: [w1653 _ _] -> [_ w1739 _]
          seq-local: [w1655 _ _] -> [_ w1736 _]
          seq-local: [_ w1724 _] -> [_ _ w1753]
          seq-local: [_ w1726 _] -> [_ _ w1752]
          seq-local: [w1651 _ _] -> [_ _ w1745]
          seq-local: [w1625 _ _] -> [_ w1682 _]
          tunnel: [_ _ w1747] -> w1615
          tunnel: [_ _ w1750] -> w1616
          tunnel: w1612 -> [_ w1691 w1744]
          tunnel: w1614 -> [w1627 _ _]
          frame #0 {
            # "Legacy requirements:"
            # "Shared requirements:"
            n948 = local read "fab1_totalWt"() -> (w1663:sgl)
            n949 = local read "fab2_totalWt"() -> (w1662:sgl)
            n950 = local read "fab3_totalWt"() -> (w1661:sgl)
            n951 = local read "fab4_totalWt"() -> (w1660:sgl)
            n952 = local read "fab5_totalWt"() -> (w1659:sgl)
            n953 = local read "fab6_totalWt"() -> (w1658:sgl)
            n954 = Build Array(w1663, w1662, w1661, w1660, w1659, w1658) -> (w1657:sgl[])
            n955 = call "SQL Statement for Sample Descritpion.vi"("error IN"=w1627, "Layer Weight Array"=w1657, "VALUES clause IN"=" VALUES (%d " ("SQL statement IN"), "INSERT clause IN"="INSERT INTO Experiments " ("SQL statement IN")) -> ("error OUT"=w1626:errorcluster, "VALUES clause OUT"=w1656:string, "INSERT clause OUT"=w1654:string)  [unwired: 1 out]
            n956 = local read "lastSamp"() -> (w1652:i32)
            n957 = Increment(x=w1652) -> (x+1=w1651:i32)
            n958 = local read "rangeOfResults"() -> (w1629:i32)
            n959 = local read "lowComplete"() -> (w1630:i32)
            n960 = local read "clayAverage"() -> (w1632:sgl)
            n961 = local read "highPartial"() -> (w1631:i32)
            n962 = control-ref of="SampleClamping"() -> (w1624:refnum<vi>)
            n963 = control-ref of="BackLayer"() -> (w1622:refnum<vi>)
            n964 = control-ref of="FrontLayer"() -> (w1621:refnum<vi>)
            n965 = control-ref of="Ballisticians"() -> (w1646:refnum<vi>)
            n966 = control-ref of="Shooters"() -> (w1642:refnum<vi>)
            n967 = control-ref of="Recorders"() -> (w1641:refnum<vi>)
            n968 = control-ref of="Submitters"() -> (w1645:refnum<vi>)
            n969 = control-ref of="SampleCoverings"() -> (w1638:refnum<vi>)
            n970 = control-ref of="ThreatGroups"() -> (w1637:refnum<vi>)
            n971 = call "Dropdown Selection (SubVI).vi"("reference"=w1646) -> ("element"=w1644:string)
            n972 = call "Dropdown Selection (SubVI).vi"("reference"=w1642) -> ("element"=w1640:string)
            n973 = call "Dropdown Selection (SubVI).vi"("reference"=w1641) -> ("element"=w1639:string)
            n974 = call "Dropdown Selection (SubVI).vi"("reference"=w1645) -> ("element"=w1643:string)
            n975 = call "Dropdown Selection (SubVI).vi"("reference"=w1638) -> ("element"=w1636:string)
            n976 = call "Dropdown Selection (SubVI).vi"("reference"=w1637) -> ("element"=w1635:string)
            n977 = call "Dropdown Selection (SubVI).vi"("reference"=w1624) -> ("element"=w1623:string)
            n978 = call "Dropdown Selection (SubVI).vi"("reference"=w1622) -> ("element"=w1620:string)
            n979 = call "Dropdown Selection (SubVI).vi"("reference"=w1621) -> ("element"=w1619:string)
            n980 = Format Into String(format string=", %d, #%s#, '%s', '%s', '%s', '%s', '%s', '%s', %.1f, '%s', %.1f, %d, %d, %d, '%s', '%s', '%s'" ("Format String"), initial string=w1656, error in=w1626, w1651, "shotTimestamp", w1644, w1640, w1639, w1643, w1636, w1635, "clayTemp", "clayCalib", w1632, w1631, w1630, w1629, w1623, w1620, w1619) -> (resulting string=w1655:string, error out=w1625:errorcluster)
            n981 = Concatenate Strings(w1654, ", expt, [date], Ballistician1, Ballistician2, Ballistician3, Submitter1, SampleCovering, ProjectileType, ClayTemp, ClayCalibration, ClayAvgThickness, highPartial, lowComplete, rangeOfResults, clamping, FrontPly, BackPly," ("Substring")) -> (w1653:string)
            n982 = flat-sequence {
              tunnel: ["TestStandards"] -> _
              tunnel: ["Shooters"] -> _
              tunnel: ["Recorders"] -> _
              tunnel: ["WeaponTypes"] -> _
              tunnel: ["Models"] -> _
              tunnel: ["serialNum"] -> _
              tunnel: ["layerStitch_1"] -> _
              tunnel: ["layerStitch_2"] -> _
              tunnel: ["layerStitch_3"] -> _
              tunnel: ["layerStitch_4"] -> _
              tunnel: ["layerStitch_5"] -> _
              tunnel: ["layerStitch_6"] -> _
              tunnel: ["minV50"] -> _
              frame #0 {
                # "PB-only requirements:"
              }
            }
          }
          frame #1 {
            w1738 = " Angle, Conditions, SampleType, ThreatGrain, ThreatDetail, V50dc, V50, maker, thickness, powder, numshots, backing, totalnumberplys, testcomments, NIJ1, method, temperature, humidity, Dimensions, zmr, ProjectID, SampleID, panelmaker, panelWeight, totalBAW)"  # INSERT clause continued
            # "Although shot angle is defined for the overall\nexperiment, it is also recorded for each shot."
            n983 = local read "computed_V50"() -> (w1734:sgl)
            n984 = local read "Drag Corrected"() -> (w1729:bool)
            n985 = local read "Impact factor"() -> (w1731:sgl)
            n986 = Array Size(array=w1691) -> (size(s)=w1722:i32)
            n987 = Select(t=w1731, s=w1729, f=sgl 1.0) -> (s? t:f=w1730:sgl)
            n988 = Divide(x=w1734, y=w1730) -> (x/y=w1733:sgl)
            n989 = control-ref of="ModelMfrs"() -> (w1717:refnum<vi>)
            n990 = control-ref of="PowderTypes"() -> (w1715:refnum<vi>)
            n991 = call "Dropdown Selection (SubVI).vi"("reference"=w1717) -> ("element"=w1716:string)
            n992 = call "Dropdown Selection (SubVI).vi"("reference"=w1715) -> ("element"=w1699:string)
            n993 = local read "GrainSize"() -> (w1680:u16)
            n994 = local read "Z.M.R."() -> (w1705:sgl)
            n995 = local read "Shot Angle"() -> (w1693:u16)
            n996 = Less Than 0?(x=w1705) -> (x < 0?=w1704:bool)
            n997 = local read "totalNumLayers"() -> (w1721:i32)
            n998 = control-ref of="ThreatDetails"() -> (w1677:refnum<vi>)
            n999 = control-ref of="SampleTypes"() -> (w1687:refnum<vi>)
            n1000 = control-ref of="TestConditions"() -> (w1706:refnum<vi>)
            n1001 = control-ref of="SampleBackings"() -> (w1714:refnum<vi>)
            n1002 = Format Into String(w1680) -> (resulting string=w1679:string)  [unwired: 3 in, 1 out]
            n1003 = local read "totalBAW"() -> (w1707:sgl)
            n1004 = case shown="True" w1704 {
              tunnel: w1705 -> [w1742 _]
              tunnel: [w1742 sgl 0.0 ("Z.M.R.")] -> w1703
              frame False {
              }
              frame True {
              }
            }
            n1005 = control-ref of="SampleDimensions"() -> (w1710:refnum<vi>)
            n1006 = control-ref of="N.I.J"() -> (w1712:refnum<vi>)
            n1007 = control-ref of="Methods"() -> (w1697:refnum<vi>)
            n1008 = control-ref of="Assemblers"() -> (w1708:refnum<vi>)
            n1009 = call "Dropdown Selection (SubVI).vi"("reference"=w1677) -> ("element"=w1678:string)
            n1010 = call "Dropdown Selection (SubVI).vi"("reference"=w1687) -> ("element"=w1686:string)
            n1011 = call "Dropdown Selection (SubVI).vi"("reference"=w1706) -> ("element"=w1692:string)
            n1012 = call "Dropdown Selection (SubVI).vi"("reference"=w1714) -> ("element"=w1713:string)
            n1013 = Equal?(x=w1679, y="") -> (x = y?=w1701:bool)
            n1014 = call "Dropdown Selection (SubVI).vi"("reference"=w1712) -> ("element"=w1711:string)
            n1015 = call "Dropdown Selection (SubVI).vi"("reference"=w1697) -> ("element"=w1696:string)
            n1016 = call "Dropdown Selection (SubVI).vi"("reference"=w1710) -> ("element"=w1709:string)
            n1017 = call "Dropdown Selection (SubVI).vi"("reference"=w1708) -> ("element"=w1698:string)
            n1018 = case shown="False" w1701 {
              tunnel: [w1740 "0" ("element")] -> w1700
              tunnel: w1679 -> [w1740 _]
              frame False {
              }
              frame True {
              }
            }
            n1019 = call "Prepare DB Connect Path (SubVI).vi"("connectString"=path "BIMS_Collector.udl", "error in"=w1682) -> ("appended path"=w1681:path, "error out"=w1683:errorcluster)  [unwired: 1 out]
            n1020 = Format Into String(format string=", %d, '%s', '%s', '%s', '%s', %.4f, %.1f, '%s', %.4f, '%s', %d, '%s', %d, '%s', '%s', '%s', %.1f, %.1f, '%s', %.1f, '%s', '%s', '%s', %.1f, %.1f);" ("Format String"), initial string=w1736, error in=w1683, w1693, w1692, w1686, w1700, w1678, w1734, w1733, w1716, "Thickness", w1699, w1722, w1713, w1721, "Comments", w1711, w1696, "RoomT", "RoomHum", w1709, w1703, "ProjectID", "SampleID", w1698, "totalSampleWt", w1707) -> (resulting string=w1735:string, error out=w1685:errorcluster)
            n1021 = call-poly <vilib>:"DB Tools Open Connection.vi"("error in (no error)"=w1685, "connection information"=w1681) -> ("error out"=w1694:errorcluster, "connection reference"=w1695:T40)  [unwired: 3 in, 3 out]
            n1022 = Concatenate Strings(w1739, w1738, w1735) -> (w1728:string)
            n1023 = call-poly <vilib>:"DB Tools Execute Query.vi"("error in (no error)"=w1694, "SQL query"=w1728, "connection reference"=w1695) -> ("error out"=w1727:errorcluster, "recordset reference"=w1725:T41)  [unwired: 1 in, 4 out]
            n1024 = call-poly <vilib>:"DB Tools Free Object.vi"("error in (no error)"=w1727, "recordset reference"=w1725) -> ("error out"=w1726:errorcluster, "connection reference"=w1724:T40)  [unwired: 8 out]
          }
          frame #2 {
            # "Experiment.expt"
            n1025 = local read "lastShot"() -> (w1751:i32)
            n1026 = Increment(x=w1751) -> (x+1=w1749:i32)
            n1027 = for {
              tunnel: w1744 -> [w1797] mode=indexing
              tunnel: w1753 -> [w1772]
              tunnel: w1752 -> [w1756]
              tunnel: [w1770] -> w1746
              tunnel: [w1771] -> w1748
              tunnel: w1749 -> [w1777]
              tunnel: [w1769] -> w1750
              tunnel: w1745 -> [w1765]
              i -> [w1769]
              w1757 = sgl 1.0 ("f")
              # "Shot.id"
              n1028 = Add(x=w1777, y=w1769) -> (x+y=w1776:i32)
              n1029 = Unbundle By Name(w1797) -> ("IMPACT VELOCITY"=w1783:sgl, "Redundant_Velocity"=w1762:sgl, "RESIDUAL  VELOCITY"=w1761:sgl, "Shot Description"=w1763:string, "Powder Loading"=w1787:sgl, "Barrel Temperature"=w1788:sgl, "TIME / DATE"=w1789:string, "shot order"=w1790:i32, "Shot Angle"=w1791:u16, "BackFace\nDepth"=w1792:sgl, "BackFace\nDiameter"=w1793:sgl, "SHOT STATUS"=w1795:u16, "Projectile Mass"=w1786:sgl, "usedv50"=w1785:bool, "Energy Loss (J)"=w1784:sgl, "avgVel_PB"=w1768:sgl, "velLoss_PB"=w1767:sgl, "strikeVel_PB"=w1766:sgl, "Frag Rod"=w1754:sgl)
              n1030 = local read "Drag Corrected"() -> (w1759:bool)
              n1031 = local read "Residual factor"() -> (w1781:sgl)
              n1032 = local read "Impact factor"() -> (w1758:sgl)
              n1033 = Select(t=w1758, s=w1759, f=w1757) -> (s? t:f=w1779:sgl)
              n1034 = Select(t=w1758, s=w1759, f=w1757) -> (s? t:f=w1764:sgl)
              n1035 = Select(t=w1781, s=w1759, f=w1757) -> (s? t:f=w1780:sgl)
              n1036 = Divide(x=w1783, y=w1779) -> (x/y=w1778:sgl)
              n1037 = Divide(x=w1762, y=w1764) -> (x/y=w1760:sgl)
              n1038 = Divide(x=w1761, y=w1780) -> (x/y=w1782:sgl)
              n1039 = Greater Than 0?(x=w1795) -> (x > 0?=w1794:bool)
              n1040 = Format Into String(format string="INSERT INTO shots (impactdc, redundantdc, residualdc,  comment, loading, barreltemp, [date], [order], shotangle, bfdepth, bfdiameter, [complete], expt, id, weight,usedv50, loss, residual, impact, redundant, avgVel_PB, velLoss_PB, strikeVel_PB, fragRod)  VALUES (%.1f, %.1f, %.1f, '%s', %.4f, %.1f, #%s#, %d, %d, %.3f, %.3f, %d, %d, %d, %.4f, %d, %.4f, %.1f, %.1f, %.1f, %.1f, %.1f, %.1f, %.1f)" ("Substring"), error in=w1756, w1783, w1762, w1761, w1763, w1787, w1788, w1789, w1790, w1791, w1792, w1793, w1794, w1765, w1776, w1786, w1785, w1784, w1782, w1778, w1760, w1768, w1767, w1766, w1754) -> (resulting string=w1773:string, error out=w1755:errorcluster)  [unwired: 1 in]
              n1041 = call-poly <vilib>:"DB Tools Execute Query.vi"("error in (no error)"=w1755, "SQL query"=w1773, "connection reference"=w1772) -> ("error out"=w1775:errorcluster, "recordset reference"=w1774:T41)  [unwired: 1 in, 4 out]
              n1042 = call-poly <vilib>:"DB Tools Free Object.vi"("error in (no error)"=w1775, "recordset reference"=w1774) -> ("error out"=w1770:errorcluster, "connection reference"=w1771:T40)  [unwired: 8 out]
            }
            n1043 = call <vilib>:"DB Tools Close Connection.vi"("error in (no error)"=w1746, "connection reference"=w1748) -> ("error out"=w1747:errorcluster)  [unwired: 5 out]
          }
        }
        n1044 = case shown="No Error" w1615 {
          selector: w1615 -> [w1809 w1828]
          tunnel: [-1 -1] -> w1617
          tunnel: [Collector_State."POLL" ("progState") Collector_State."POLL" ("progState")] -> w1618
          tunnel: w1616 -> [w1812 _]
          tunnel: [w1805 w1826] -> w1613
          tunnel: w1612 -> [w1804 w1825]
          tunnel: [w1802 w1825] -> w1611
          frame No Error {
            n1045 = local read "lastSamp"() -> (w1811:i32)
            n1046 = local read "configPath"() -> (w1799:path)
            n1047 = local read "lastShot"() -> (w1813:i32)
            n1048 = flat-sequence {
              tunnel: w1805 -> [_]
              tunnel: w1801 -> [w1823]
              tunnel: [w1823] -> w1802
              frame #0 {
                w1816 = T15."Disabled and Grayed Out" ("Disabled")
                n1049 = property on="saveReq" class="Str"("Visible"=TRUE) -> ()  [unwired: 2 in, 2 out]
                n1050 = local write "SampleID"("") -> ()
                n1051 = property on="clearShots" class="Bool"("Disabled"=T15."Enabled") -> ()  [unwired: 2 in, 2 out]
                n1052 = property on="addShot" class="Bool"("Disabled"=w1816) -> ()  [unwired: 2 in, 2 out]
                n1053 = property on="undoLastShot" class="Bool"("Disabled"=w1816) -> ()  [unwired: 2 in, 2 out]
                n1054 = property on="saveShots" class="Bool"("Disabled"=w1816) -> ()  [unwired: 2 in, 2 out]
                n1055 = property on="mainTabCntrl" class="TabCtl (strict)"("Val(Sgnl)"=enum32{"Setup", "Measure", "History", "System"}."Setup" ("mainTabCntrl")) -> ()  [unwired: 2 in, 2 out]
                n1056 = One Button Dialog(message="Data Saved. Enter new Sample ID.") -> ()  [unwired: 1 in, 1 out]
                n1057 = property on="SampleEntryTabCntrl" class="TabCtl (strict)"("Value"=enum32{"Environment", "Sample"}."Sample" ("SampleEntryTabCntrl")) -> ()  [unwired: 2 in, 2 out]
                n1058 = property on="Sample SubTabCntrl" class="TabCtl (strict)"("Value"=T2."General Specification" ("Sample SubTabCntrl")) -> ()  [unwired: 2 in, 2 out]
              }
            }
            n1059 = Array Size(array=w1804) -> (size(s)=w1803:i32)
            n1060 = Increment(x=w1813) -> (x+1=w1810:i32)
            n1061 = for {
              N: w1803 -> [_]
              shift-right: [w1814] -> w1801
              shift-left: w1804 -> [w1815]
              n1062 = Delete From Array(array=w1815) -> (array with subset deleted=w1814:T6)  [unwired: 2 in, 1 out]
            }
            n1063 = Add(x=w1810, y=w1812) -> (x+y=w1800:i32)
            n1064 = Increment(x=w1811) -> (x+1=w1798:i32)
            n1065 = local write "lastShot"(w1800) -> ()
            n1066 = call "save stats to INI (SubVI).vi"("lastSamp"=w1798, "errIN"=w1809, "lastShot"=w1800, "configPath"=w1799) -> ("errOUT"=w1805:errorcluster, "recordNum"=w1808:dbl)  [unwired: 6 in]
            n1067 = property on="Record #" class="DigNum (strict)"("Maximum"=w1808) -> ()  [unwired: 2 in, 2 out]
            n1068 = local write "lastSamp"(w1798) -> ()
            n1069 = property on="shotsArr" class="Arr (strict)"("Val(Sgnl)"=w1801) -> ()  [unwired: 2 in, 2 out]
          }
          frame Error {
            n1070 = One Button Dialog(message="Error saving Data. ") -> ()  [unwired: 2 out]
            n1071 = call <vilib>:"General Error Handler.vi"("error in (no error)"=w1828) -> ("error out"=w1826:errorcluster)  [unwired: 2 in, 12 out]
          }
        }
      }
      frame "ADD SHOT" {
        # "case # 5"
        # "Shot Order"
        # "This section accepts new data to the shot table."
        n1072 = local read "Impact/speed"() -> (w1868:sgl)
        n1073 = local read "residual/speed"() -> (w1864:sgl)
        n1074 = property on="undoLastShot" class="Bool"(error in=w1843, "Disabled"=T15."Enabled") -> (error out=w1842:errorcluster)  [unwired: 1 in, 1 out]
        n1075 = local read "Current/residual/speed"() -> (w1853:sgl)
        n1076 = local read "CorrectedVelScrnSet1"() -> (w1854:sgl)
        n1077 = local read "CorrectedVelScrnSet2"() -> (w1873:sgl)
        n1078 = local read "Current/avg/speed"() -> (w1875:sgl)
        n1079 = local read "Corrected Residual"() -> (w1852:sgl)
        n1080 = local read "Redundant/speed"() -> (w1872:sgl)
        n1081 = local read "conversion factor"() -> (w1862:sgl)
        n1082 = local read "MeasVelScrnSet1"() -> (w1871:sgl)
        n1083 = local read "MeasVelScrnSet2"() -> (w1870:sgl)
        n1084 = local read "Projectile Mass"() -> (w1844:sgl)
        n1085 = case shown="\"grains\"" "loadingUnits" {
          tunnel: [w1881 w1882] -> w1838
          tunnel: "Powder Loading" -> [w1881 w1883]
          frame "grams", Default {
            # "Always save in grams."
          }
          frame "grains" {
            # "Always save in grams."
            n1086 = Multiply(x=w1883, y=sgl 0.06479891) -> (x*y=w1882:sgl)
          }
        }
        n1087 = local read "Avg/speed"() -> (w1874:sgl)
        n1088 = Array Size(array=w1847) -> (size(s)=w1850:i32)
        n1089 = Multiply(x=w1868, y=w1862) -> (x*y=w1860:sgl)
        n1090 = Multiply(x=w1862, y=w1864) -> (x*y=w1861:sgl)
        n1091 = Increment(x=w1850) -> (x+1=w1869:i32)
        n1092 = Multiply(x=w1860, y=w1860) -> (x*y=w1856:sgl)
        n1093 = Multiply(x=w1861, y=w1861) -> (x*y=w1857:sgl)
        n1094 = Subtract(x=w1856, y=w1857) -> (x-y=w1858:sgl)
        n1095 = Compound Arithmetic op=MULTIPLY(w1844, w1858, sgl 0.0005 ("Input")) -> (w1863:sgl)
        n1096 = Format Date/Time String(time format string (%c)="%x   %H:%M:%S") -> (date/time string=w1865:string)  [unwired: 2 out]
        "SUBMIT DATE/TIME" <- w1865
        n1097 = Index Array(array=w1847) -> (element=w1849:T7)  [unwired: 1 in]
        n1098 = Bundle By Name(cluster=w1849, "TIME / DATE"=w1865, "shot order"=w1869, "IMPACT VELOCITY"=w1868, "RESIDUAL  VELOCITY"=w1864, "Shot Description"="Shot Description", "Powder Loading"=w1838, "Barrel Temperature"="Barrel Temp", "SHOT STATUS"="Current/shotstatus", "BackFace\nDepth"="backdepth", "Shot Angle"="Shot Angle", "Uncorrected Impact"=w1871, "Corrected Impact"=w1854, "Uncorrected Residual"=w1853, "Corrected residual"=w1852, "Projectile Mass"=w1844, "Energy Loss (J)"=w1863, "UncorrectedRed_PB"=w1870, "Redundant_Velocity"=w1872, "CorrectedRed_PB"=w1873, "UncorrectedAvgVel_PB"=w1875, "avgVel_PB"=w1874, "Frag Rod"="Frag Rod", "V50userExcl"=FALSE) -> (w1851:T7)
        n1099 = Build Array (concatenate)(w1847, w1851) -> (w1834:T6)
        n1100 = flat-sequence {
          tunnel: w1842 -> [w1879]
          tunnel: [w1878] -> w1841
          tunnel: w1834 -> [w1876]
          tunnel: [w1876] -> w1833
          frame #0 {
            n1101 = local write "backdepth"(sgl 0.0 ("BACKFACE DEPTH")) -> ()
            n1102 = property on="shotsTabCntrl" class="TabCtl (strict)"(error in=w1879, "Value"=T5."Shots Table" ("shotsTabCntrl")) -> (error out=w1878:errorcluster)  [unwired: 1 in, 1 out]
          }
        }
      }
      frame "CLEAR SHOTS" {
        # "case # 6"
        # "This section will clear the shot table and re-enable the \"ADD SHOT\" button to get ready for a new test panel."
        n1103 = Two Button Dialog(message="Shot table cleared even if not saved. Are you sure?", 1:"NO" ("F button name (\"Cancel\")"), 2:"YES" ("T button name (\"OK\")")) -> (T button?=w1888:bool)
        n1104 = case shown="True" w1888 {
          tunnel: [w1894 T6 [{"Uncorrected Impact"=0.0, "Uncorrected Residual"=0.0, "avgVel_PB"=0.0, "IMPACT VELOCITY"=0.0, "RESIDUAL  VELOCITY "=0.0, "Shot Description"="", "Powder Loading "=0.0, "Barrel Temperature"=0.0, "TIME / DATE"="", "shot order"=1, "SHOT STATUS"=1, "Shot Angle"=0, "Corrected Impact"=0.0, "Corrected residual"=0.0, "Projectile Mass"=0.0, "usedv50"=FALSE, "Energy Loss (J)"=0.0, "BackFace\nDepth"=0.0, "BackFace\nDiameter"=0.0, "Redundant_Velocity"=0.0, "velLoss_PB"=0.0, "strikeVel_PB"=0.0, "UncorrectedRed_PB"=0.0, "CorrectedRed_PB"=0.0, "UncorrectedAvgVel_PB"=0.0, "V50userExcl"=FALSE, "Frag Rod"=0.0}] ("shotsArr")] -> w1893
          tunnel: w1889 -> [w1894 _]
          frame False {
          }
          frame True {
            w1896 = T15."Disabled and Grayed Out" ("Disabled")
            n1105 = invoke on="Table of Shots" class="Tbl (strict)" method="Reinit To Default"() -> ()  [unwired: 3 in, 3 out]
            n1106 = property on="addShot" class="Bool"("Disabled"=T15."Enabled") -> ()  [unwired: 2 in, 2 out]
            n1107 = invoke on="shotsArr" class="Arr (strict)" method="Reinit To Default"() -> ()  [unwired: 3 in, 3 out]
            n1108 = property on="saveReq" class="Str"("Visible"=TRUE) -> ()  [unwired: 2 in, 2 out]
            n1109 = property on="clearShots" class="Bool"("Disabled"=w1896) -> ()  [unwired: 2 in, 2 out]
            n1110 = property on="undoLastShot" class="Bool"("Disabled"=w1896) -> ()  [unwired: 2 in, 2 out]
            n1111 = property on="saveShots" class="Bool"("Disabled"=w1896) -> ()  [unwired: 2 in, 2 out]
          }
        }
      }
      frame "NEXT SHOT" {
        # "case # 7"
        n1112 = property on="shotsArr" class="Arr (strict)"(error in=w1902) -> (error out=w1901:errorcluster, "Index Values"=w1906:u32[])  [unwired: 1 in, 1 out]
        n1113 = Array Size(array=w1899) -> (size(s)=w1909:i32)
        n1114 = Index Array "Index Array"(array=w1906) -> (element=w1911:u32)  [unwired: 1 in]
        n1115 = To Unsigned Long Integer(number=w1909) -> (unsigned 32bit integer=w1905:u32)
        n1116 = Increment(x=w1911) -> (x+1=w1910:u32)
        n1117 = Quotient & Remainder(x=w1910, y=w1905) -> (x-y*floor(x/y)=w1908:u32)  [unwired: 1 out]
        n1118 = Replace Array Subset "Replace Array Subset"(array=w1906, new element=w1908) -> (w1907:u32[])  [unwired: 1 in]
        n1119 = property on="shotsArr" class="Arr (strict)"(error in=w1901, "Index Values"=w1907) -> (error out=w1900:errorcluster)  [unwired: 1 in, 1 out]
      }
      frame "DELETE SHOT" {
        # "case # 8"
        # "This section undoes new shot data OR deletes the currently accessed previous shot"
        n1120 = local read "deleteShot"() -> (w1918:bool)
        n1121 = case shown="False" w1918 {
          tunnel: w1917 -> [w1922 w1933]
          tunnel: [w1923 w1934] -> w1914
          frame False {
            n1122 = Array Size(array=w1922) -> (size(s)=w1920:i32)
            n1123 = while {
              tunnel: [w1924] -> w1921
              tunnel: w1920 -> [w1926]
              tunnel: w1922 -> [w1928] mode=indexing
              i -> [w1924]
              stop <- w1927 stop-if-true
              n1124 = Unbundle By Name(w1928) -> ("shot order"=w1925:i32)
              n1125 = Equal?(x=w1925, y=w1926) -> (x = y?=w1927:bool)
            }
            n1126 = Delete From Array "Delete From Array"(array=w1922, index=w1921) -> (array with subset deleted=w1923:T6)  [unwired: 1 in, 1 out]
            n1127 = property on="undoLastShot" class="Bool"("Disabled"=T15."Disabled and Grayed Out") -> ()  [unwired: 2 in, 2 out]
          }
          frame True {
            n1128 = property on="shotsArr" class="Arr (strict)"() -> ("Index Values"=w1942:u32[])  [unwired: 2 in, 2 out]
            n1129 = local write "deleteShot"(FALSE) -> ()
            n1130 = Index Array(array=w1942, index=0 ("Index")) -> (element=w1932:u32)
            n1131 = To Long Integer(number=w1932) -> (32bit integer=w1929:i32)
            n1132 = Index Array(array=w1933, index=w1929) -> (element=w1931:T7)
            n1133 = Unbundle By Name(w1931) -> ("shot order"=w1930:i32)
            n1134 = Format Into String(format string="The currently displayed Shot, #%d", w1930) -> (resulting string=w1939:string)  [unwired: 2 in, 1 out]
            n1135 = Concatenate Strings(w1939, ", will be deleted.  IT CANNOT RECOVERED!  Do you want to DELETE the shot?" ("message")) -> (w1938:string)
            n1136 = Two Button Dialog(message=w1938, 1:"NO I do NOT want to delete.  Cancel Request" ("F button name (\"Cancel\")"), 2:"YES I want to delete the shot" ("T button name (\"OK\")")) -> (T button?=w1945:bool)
            n1137 = case shown="True" w1945 {
              tunnel: w1933 -> [w1958 w1961]
              tunnel: [w1958 w1963] -> w1936
              tunnel: w1929 -> [_ w1960]
              tunnel: [10000 ("shot order") w1962] -> w1935
              frame False {
              }
              frame True {
                n1138 = Index Array(array=w1961, index=w1960) -> (element=w1959:T7)
                n1139 = Unbundle By Name(w1959) -> ("shot order"=w1962:i32)
                n1140 = Delete From Array(array=w1961, index=w1960) -> (array with subset deleted=w1963:T6)  [unwired: 1 in, 1 out]
              }
            }
            n1141 = for {
              tunnel: [w1952] -> w1934 mode=indexing
              tunnel: w1936 -> [w1947] mode=indexing
              tunnel: w1935 -> [w1951]
              n1142 = Unbundle By Name(w1947) -> ("shot order"=w1949:i32)
              n1143 = Decrement(x=w1949) -> (x-1=w1948:i32)
              n1144 = Greater?(x=w1949, y=w1951) -> (0:w1950:bool)
              n1145 = case shown="True" w1950 {
                tunnel: w1948 -> [_ w1955]
                tunnel: w1947 -> [w1953 w1956]
                tunnel: [w1953 w1954] -> w1952
                frame False {
                }
                frame True {
                  n1146 = Bundle By Name(cluster=w1956, "shot order"=w1955) -> (w1954:T7)
                }
              }
            }
          }
        }
        n1147 = property on="shotsArr" class="Arr (strict)"(error in=w1913, "Val(Sgnl)"=w1914) -> (error out=w1912:errorcluster)  [unwired: 1 in, 1 out]
      }
      frame "READY CLOCK" {
        # "case # 9"
        n1148 = case shown="\"Screens\"" "MeasSrc" {
          tunnel: w1965 -> [w1972 w1977 w1979]
          tunnel: [w1970 w1977 w1979] -> w1964
          frame "Simulated", Default {
            n1149 = flat-sequence {
              tunnel: w1972 -> [w1973]
              tunnel: [w1973] -> w1971
              tunnel: [w1975] -> w1970
              tunnel: w1971 -> [w1975]
              frame #0 {
                n1150 = local write "readyClock"(FALSE ("RANGE RESET")) -> ()
              }
              frame #1 {
                n1151 = Wait (ms)(milliseconds to wait=u32 100) -> ()  [unwired: 1 out]
              }
            }
          }
          frame "Radar" {
          }
          frame "Screens" {
            n1152 = local write "readyClock"(FALSE ("RANGE RESET")) -> ()
          }
        }
      }
      frame "PROC SHOTS" {
        # "case # 10"
        n1153 = local write "processShots"(FALSE ("ProcessShots")) -> ()
        n1154 = local read "Drag Corrected"() -> (w1985:bool)
        n1155 = stacked-sequence {
          seq-local: [_ w2043 _ _] -> [_ _ w2075 w2125]
          seq-local: [w1988 _ _ _] -> [_ w2039 _ _]
          seq-local: [w2006 _ _ _] -> [_ w2040 _ _]
          seq-local: [w2007 _ _ _] -> [_ w2041 _ _]
          tunnel: [_ _ _ w2118] -> w1986
          tunnel: w1985 -> [w2009 w2042 _ _]
          tunnel: w1982 -> [_ w2038 _ _]
          tunnel: w1981 -> [w2005 _ _ _]
          tunnel: [w2005 _ _ _] -> w1980
          frame #0 {
            n1156 = disable-structure "Diagram Disable Structure" shown="Enabled" {
              disable-tunnel: [w2026 w2033] -> w2014
              frame Disabled {
                n1157 = local read "factor array"() -> (w2028:sgl[])
                n1158 = local read "Threat"() -> (w2025:u16)
                n1159 = To Long Integer(number=w2025) -> (32bit integer=w2027:i32)
                n1160 = Index Array(array=w2028, index=w2027) -> (element=w2026:sgl)
              }
              frame Enabled {
                n1161 = local read "threatDetails"() -> (w2032:T1)
                n1162 = Unbundle By Name(w2032) -> ("dragCorrection"=w2030:string)
                n1163 = Not Equal?(x=w2030, y="") -> (x != y?=w2031:bool)
                n1164 = case shown="True" w2031 {
                  tunnel: [sgl 1.0 ("default value 1") w2036] -> w2033
                  tunnel: w2030 -> [_ w2035]
                  frame False {
                  }
                  frame True {
                    n1165 = Scan From String(input string=w2035, default 1=sgl 0.0 ("default value 1")) -> (output 1=w2036:sgl)  [unwired: 3 in, 3 out]
                  }
                }
              }
            }
            "correction coefficient" <- w2014
            n1166 = local read "Current/avg/speed"() -> (w2010:sgl)
            n1167 = local read "mid_to_targ_dist"() -> (w2011:sgl)
            n1168 = local read "lengthUnits"() -> (w2008:string)
            n1169 = call "Compute Strike Velocity.vi"("drag coefficient"=w2014, "decay distance"=w2011, "raw velocity"=w2010, "distance units"=w2008) -> ("correction factor"=w1988:sgl, "strike velocity"=w2012:sgl)  [unwired: 1 out]
            "DC_ factor" <- w1988
            "Corrected Average" <- w2012
            n1170 = call "Velocity Correction.vi"("raw impact"="MeasVelScrnSet1", "distance units"=w2008, "raw redundant"="MeasVelScrnSet2", "raw residual"="Current/residual/speed", "screen set midpt to target"="Set#1_to_Target", "residual screen to target"="Residual/Target Dist", "correction coefficient"=w2014) -> ("corrected impact"=w2019:sgl, "corrected redundant"=w2015:sgl, "corrected residual"=w2017:sgl, "impact factor"=w2006:sgl, "conversion factor"=→"conversion factor":sgl, "residual factor"=w2007:sgl)  [unwired: 3 out]
            "Residual factor" <- w2007
            "Impact factor" <- w2006
            "CorrectedVelScrnSet1" <- w2019
            "Corrected Residual" <- w2017
            "CorrectedVelScrnSet2" <- w2015
            n1171 = Select(t=w2015, s=w2009, f="MeasVelScrnSet2") -> (s? t:f=→"Redundant/speed":sgl)
            n1172 = Select(t=w2012, s=w2009, f=w2010) -> (s? t:f=→"Avg/speed":sgl)
            n1173 = Select(t=w2019, s=w2009, f="MeasVelScrnSet1") -> (s? t:f=→"Impact/speed":sgl)
            n1174 = Select(t=w2017, s=w2009, f="Current/residual/speed") -> (s? t:f=→"residual/speed":sgl)
            n1175 = Add(x="MeasVelScrnSet2", y="MeasVelScrnSet1") -> (x+y=w1992:sgl)
            n1176 = Subtract(x="MeasVelScrnSet2", y="MeasVelScrnSet1") -> (x-y=w1991:sgl)
            n1177 = Divide(x=w1992, y=sgl 200.0) -> (x/y=w1993:sgl)
            n1178 = Divide(x=w1991, y=w1993) -> (x/y=w1997:sgl)
            "%_Difference" <- w1997
            n1179 = Absolute Value(x=w1997) -> (abs(x)=w1999:sgl)
            n1180 = Less?(x=w1999, y="percent warning") -> (x < y?=w2004:bool)
            n1181 = Select(t=u32 65343, s=w2004, f=u32 15668992) -> (s? t:f=w2000:u32)
            n1182 = Select(t=u32 0, s=w2004, f=u32 16777226) -> (s? t:f=w2003:u32)
            n1183 = property on="%_Difference" class="DigNum (strict)"("Numeric Text.Text Colors:BG Color"=w2000, "NumText.TextColor"=w2003) -> ()  [unwired: 2 in, 2 out]
          }
          frame #1 {
            # "<-- DC_factor (for Average of impact and redundant)"
            # "IF drag corrected THEN apply factors"
            # "Residual factor"
            # "Impact factor\n(also applies to\nredundant velocity)"
            n1184 = for {
              tunnel: w2038 -> [w2054] mode=indexing
              tunnel: w2041 -> [w2063]
              tunnel: w2040 -> [w2058]
              tunnel: w2042 -> [w2052]
              tunnel: [w2065] -> w2043 mode=indexing
              tunnel: w2039 -> [w2048]
              n1185 = Unbundle By Name(w2054) -> ("UncorrectedAvgVel_PB"=w2053:sgl)
              n1186 = Unbundle By Name(w2054) -> ("UncorrectedRed_PB"=w2060:sgl)
              n1187 = Unbundle By Name(w2054) -> ("Uncorrected Impact"=w2057:sgl)
              n1188 = Unbundle By Name(w2054) -> ("Uncorrected Residual"=w2062:sgl)
              n1189 = Multiply(x=w2048, y=w2053) -> (x*y=w2050:sgl)
              n1190 = Multiply(x=w2058, y=w2060) -> (x*y=w2059:sgl)
              n1191 = Multiply(x=w2058, y=w2057) -> (x*y=w2049:sgl)
              n1192 = Multiply(x=w2063, y=w2062) -> (x*y=w2055:sgl)
              n1193 = Select(t=w2050, s=w2052, f=w2053) -> (s? t:f=w2051:sgl)
              n1194 = Select(t=w2059, s=w2052, f=w2060) -> (s? t:f=w2061:sgl)
              n1195 = Select(t=w2055, s=w2052, f=w2062) -> (s? t:f=w2064:sgl)
              n1196 = Select(t=w2049, s=w2052, f=w2057) -> (s? t:f=w2056:sgl)
              n1197 = Subtract(x=w2051, y=w2050) -> (x-y=w2045:sgl)
              n1198 = Not A Number/Path/Refnum?(number/path/refnum=w2045) -> (NaN/Path/Refnum?=w2047:bool)
              n1199 = Select(t=sgl 0.0, s=w2047, f=w2045) -> (s? t:f=w2044:sgl)
              n1200 = Bundle By Name(cluster=w2054, "velLoss_PB"=w2044, "strikeVel_PB"=w2050, "avgVel_PB"=w2051, "CorrectedRed_PB"=w2059, "Redundant_Velocity"=w2061, "Corrected Impact"=w2049, "IMPACT VELOCITY"=w2056, "Corrected residual"=w2055, "RESIDUAL  VELOCITY"=w2064) -> (w2065:T7)
            }
          }
          frame #2 {
            w2076 = sgl[] [] ("Partial")
            # "This section calculates the V50"
            n1201 = for {
              shift-right: [w2100] -> w2078
              shift-left: w2076 -> [w2101]
              shift-right: [w2098] -> w2077
              shift-left: w2076 -> [w2099]
              tunnel: w2075 -> [w2092] mode=indexing
              n1202 = Unbundle By Name(w2092) -> ("SHOT STATUS"=w2097:u16)
              n1203 = Unbundle By Name(w2092) -> ("V50userExcl"=w2091:bool)
              n1204 = Unbundle By Name(w2092) -> ("IMPACT VELOCITY"=w2096:sgl)
              n1205 = Unbundle By Name(w2092) -> ("strikeVel_PB"=w2095:sgl)
              n1206 = Select(t=w2095, s="ScreenSetAvgg", f=w2096) -> (s? t:f=w2094:sgl)
              n1207 = case shown="False" w2091 {
                tunnel: w2101 -> [w2107 w2117]
                tunnel: [w2106 w2117] -> w2100
                tunnel: w2099 -> [w2105 w2116]
                tunnel: [w2104 w2116] -> w2098
                tunnel: w2097 -> [w2103 _]
                tunnel: w2094 -> [w2102 _]
                frame False {
                  n1208 = case shown="1" w2103 {
                    tunnel: w2102 -> [w2108 w2112]
                    tunnel: [w2111 w2113] -> w2106
                    tunnel: w2107 -> [w2110 w2113]
                    tunnel: w2105 -> [w2109 w2115]
                    tunnel: [w2109 w2114] -> w2104
                    frame 0, Default {
                      n1209 = Build Array (concatenate)(w2110, w2108) -> (w2111:sgl[])
                    }
                    frame 1 {
                      n1210 = Build Array (concatenate)(w2115, w2112) -> (w2114:sgl[])
                    }
                  }
                }
                frame True {
                }
              }
            }
            n1211 = Sort 1D Array(array=w2078) -> (sorted array=w2090:sgl[])
            n1212 = Sort 1D Array(array=w2077) -> (sorted array=w2083:sgl[])
            "Complete" <- w2083
            n1213 = Reverse 1D Array(array=w2090) -> (reversed array=w2081:sgl[])
            "Partial" <- w2081
            n1214 = Array Size(array=w2083) -> (size(s)=→"#_completes":i32)
            n1215 = Array Size(array=w2081) -> (size(s)=→"#_partials":i32)
            n1216 = Array Max & Min(array=w2081) -> (max value=w2087:sgl)  [unwired: 3 out]
            n1217 = Array Max & Min(array=w2083) -> (min value=w2085:sgl)  [unwired: 3 out]
            n1218 = call "Compute V50.vi"("Partial"=w2081, "Maximum Deviation"="maxDev", "Complete"=w2083) -> ("Pairs"=→"Pairs":i16, "zmr"=w2066:sgl, "V50"=→"computed_V50":sgl)  [unwired: 2 out]
            "Z.M.R." <- w2066
            n1219 = To Long Integer(number=w2087) -> (32bit integer=→"highPartial":i32)
            n1220 = To Long Integer(number=w2085) -> (32bit integer=→"lowComplete":i32)
            n1221 = Absolute Value(x=w2066) -> (abs(x)=→"zmr 2":sgl)
            n1222 = Less Than 0?(x=w2066) -> (x < 0?=w2069:bool)
            n1223 = Select(t="Low C minus High P", s=w2069, f="ZMR") -> (s? t:f=w2072:string)
            n1224 = Select(t=u32 65336, s=w2069, f=u32 16755266) -> (s? t:f=w2073:u32)
            n1225 = property on="zmr 2" class="DigNum (strict)"("Caption.Text"=w2072, "Numeric Text.Text Colors:BG Color"=w2073) -> ()  [unwired: 2 in, 2 out]
          }
          frame #3 {
            n1226 = local read "Pairs"() -> (w2130:i16)
            n1227 = Sort 1D Array(array=w2125) -> (sorted array=w2128:T7[])
            n1228 = for {
              tunnel: w2128 -> [w2178] mode=indexing
              tunnel: w2130 -> [w2188]
              shift-right: [w2187] -> _
              shift-left: i16 0 -> [w2186]
              tunnel: [w2180] -> w2126 mode=indexing
              # "this section marks the lowest completes that are used in V50"
              n1229 = Unbundle By Name(w2178) -> ("SHOT STATUS"=w2184:u16, "Projectile Mass"=w2182:sgl, "avgVel_PB"=w2181:sgl, "RESIDUAL  VELOCITY"=w2183:sgl)
              n1230 = Unbundle By Name(w2178) -> ("V50userExcl"=w2179:bool)
              n1231 = local read "conversion factor"() -> (w2189:sgl)
              n1232 = case shown="False" w2179 {
                tunnel: w2188 -> [w2200 _]
                tunnel: [w2199 w2209] -> w2187
                tunnel: w2186 -> [w2198 w2209]
                tunnel: [w2197 FALSE] -> w2185
                tunnel: w2184 -> [w2196 _]
                frame False {
                  n1233 = case shown="1" w2196 {
                    tunnel: w2200 -> [_ w2207]
                    tunnel: [FALSE w2206] -> w2197
                    tunnel: [w2202 w2205] -> w2199
                    tunnel: w2198 -> [w2202 w2203]
                    frame 0, Default {
                    }
                    frame 1 {
                      n1234 = Less?(x=w2203, y=w2207) -> (x < y?=w2206:bool)
                      n1235 = Add(x=w2203, y=i16 1 ("t")) -> (x+y=w2205:i16)
                    }
                  }
                }
                frame True {
                }
              }
              n1236 = Multiply(x=w2189, y=w2183) -> (x*y=w2190:sgl)
              n1237 = Multiply(x=w2181, y=w2189) -> (x*y=w2191:sgl)
              n1238 = Multiply(x=w2191, y=w2191) -> (x*y=w2195:sgl)
              n1239 = Multiply(x=w2190, y=w2190) -> (x*y=w2194:sgl)
              n1240 = Subtract(x=w2195, y=w2194) -> (x-y=w2193:sgl)
              n1241 = Compound Arithmetic op=MULTIPLY(w2182, w2193, sgl 0.0005 ("Input")) -> (w2176:sgl)
              n1242 = Not A Number/Path/Refnum?(number/path/refnum=w2176) -> (NaN/Path/Refnum?=w2177:bool)
              n1243 = Select(t=sgl 0.0, s=w2177, f=w2176) -> (s? t:f=w2174:sgl)
              n1244 = Bundle By Name(cluster=w2178, "usedv50"=w2185, "Energy Loss (J)"=w2174) -> (w2180:T7)
            }
            n1245 = Reverse 1D Array(array=w2126) -> (reversed array=w2127:T7[])
            n1246 = for {
              tunnel: w2127 -> [w2150] mode=indexing
              tunnel: w2130 -> [w2157]
              shift-right: [w2155] -> _
              shift-left: i16 0 -> [w2156]
              tunnel: [w2153] -> w2118 mode=indexing
              # "chooses highest partials used in v50"
              n1247 = Unbundle By Name(w2150) -> ("SHOT STATUS"=w2158:u16, "usedv50"=w2152:bool)
              n1248 = Unbundle By Name(w2150) -> ("V50userExcl"=w2151:bool)
              n1249 = case shown="False" w2151 {
                tunnel: w2158 -> [w2164 _]
                tunnel: w2157 -> [w2163 _]
                tunnel: w2156 -> [w2162 w2173]
                tunnel: [w2161 w2173] -> w2155
                tunnel: [w2160 FALSE ("usedv50")] -> w2154
                tunnel: w2152 -> [w2159 _]
                frame False {
                  n1250 = case shown="1" w2164 {
                    tunnel: w2163 -> [w2168 _]
                    tunnel: [w2167 w2171] -> w2160
                    tunnel: w2162 -> [w2165 w2170]
                    tunnel: [w2166 w2170] -> w2161
                    tunnel: w2159 -> [_ w2171]
                    frame 0, Default {
                      n1251 = Less?(x=w2165, y=w2168) -> (x < y?=w2167:bool)
                      n1252 = Add(x=w2165, y=i16 1) -> (x+y=w2166:i16)
                    }
                    frame 1 {
                    }
                  }
                }
                frame True {
                }
              }
              n1253 = Bundle By Name(cluster=w2150, "usedv50"=w2154) -> (w2153:T7)
            }
            n1254 = for {
              shift-right: [w2136] -> w2119
              shift-left: sgl[] [] ("Partial") -> [w2133]
              tunnel: w2118 -> [w2135] mode=indexing
              n1255 = local read "ScreenSetAvgg"() -> (w2140:bool)
              n1256 = Unbundle By Name(w2135) -> ("V50userExcl"=w2134:bool, "usedv50"=w2132:bool)
              n1257 = Unbundle By Name(w2135) -> ("IMPACT VELOCITY"=w2138:sgl)
              n1258 = Unbundle By Name(w2135) -> ("strikeVel_PB"=w2139:sgl)
              n1259 = Select(t=w2139, s=w2140, f=w2138) -> (s? t:f=w2137:sgl)
              n1260 = case shown="False" w2134 {
                tunnel: w2137 -> [w2141 _]
                tunnel: [w2142 w2149] -> w2136
                tunnel: w2133 -> [w2143 w2149]
                tunnel: w2132 -> [w2144 _]
                frame False {
                  n1261 = case shown="False" w2144 {
                    tunnel: w2143 -> [w2145 w2148]
                    tunnel: [w2145 w2147] -> w2142
                    tunnel: w2141 -> [_ w2146]
                    frame False {
                    }
                    frame True {
                      n1262 = Build Array (concatenate)(w2148, w2146) -> (w2147:sgl[])
                    }
                  }
                }
                frame True {
                }
              }
            }
            n1263 = Array Max & Min(array=w2119) -> (max value=w2124:sgl, min value=w2123:sgl)  [unwired: 2 out]
            n1264 = Subtract(x=w2124, y=w2123) -> (x-y=w2122:sgl)
            n1265 = property on="shotsArr" class="Arr (strict)"("Val(Sgnl)"=w2118) -> ()  [unwired: 2 in, 2 out]
            n1266 = To Long Integer(number=w2122) -> (32bit integer=→"rangeOfResults":i32)
          }
        }
      }
      frame "CHECK DAQ" {
        w2215 = 500  # timeout in ms
        # "case # 11"
        n1267 = Dequeue Element(queue=w2210, timeout in ms (-1)=w2215, error in (no error)=w2211) -> (element=w2214:dbl[], timed out?=w2213:bool, error out=w2212:errorcluster)  [unwired: 1 out]
        n1268 = case shown="False" w2213 {
          tunnel: [Collector_State."PROC SHOTS" ("progState") Collector_State."POLL" ("progState")] -> w2218
          tunnel: [-1 -1 ("index of element")] -> w2217
          tunnel: [w2226 w2279] -> w2216
          tunnel: w2212 -> [w2220 w2279]
          tunnel: w2214 -> [w2221 _]
          frame False {
            n1269 = local read "MeasSrc"() -> (w2225:T12)
            n1270 = case shown="\"Screens\"" w2225 {
              tunnel: [w2233 w2254 w2275] -> w2224
              tunnel: w2220 -> [w2231 w2253 w2267]
              tunnel: [w2231 w2253 w2274] -> w2226
              tunnel: w2221 -> [_ _ w2273]
              tunnel: [w2230 w2252 w2258] -> w2223
              tunnel: [w2229 w2251 w2257] -> w2222
              frame "Simulated", Default {
                # "Simulated"
                n1271 = local read "minV50"() -> (w2236:i32)
                n1272 = local read "Powder Loading"() -> (w2250:sgl)
                n1273 = Wait (ms)(milliseconds to wait=u32 500 ("number")) -> ()  [unwired: 1 out]
                n1274 = To Single Precision Float(number=w2236) -> (single precision float=w2235:sgl)
                n1275 = call "Get Shell Speed.vi"("loading"=w2250, "v50"=w2235) -> ("impact"=w2230:sgl, "residual"=w2245:sgl)  [unwired: 1 in, 2 out]
                n1276 = Greater Than 0?(x=w2245) -> (x > 0?=w2247:bool)
                n1277 = local write "Current/residual/speed"(w2245) -> ()
                n1278 = Select(t=u16 1, s=w2247, f=u16 0) -> (s? t:f=w2246:u16)
                n1279 = local write "Current/shotstatus"(w2246) -> ()
                n1280 = Random Number (0-1)() -> (number: 0 to 1=w2243:dbl)
                n1281 = To Single Precision Float(number=w2243) -> (single precision float=w2239:sgl)
                n1282 = Multiply(x=w2239, y=sgl 0.002) -> (x*y=w2242:sgl)
                n1283 = local write "readyClock"(TRUE ("RANGE RESET")) -> ()
                n1284 = Add(x=w2242, y=sgl 0.999) -> (x+y=w2240:sgl)
                n1285 = Multiply(x=w2230, y=w2240) -> (x*y=w2229:sgl)
                n1286 = Add(x=w2230, y=w2229) -> (x+y=w2237:sgl)
                n1287 = Divide(x=w2237, y=sgl 2.0 ("v50")) -> (x/y=w2233:sgl)
              }
              frame "Radar" {
                # "Radar -- (future)"
                n1288 = local read "MeasVelScrnSet1"() -> (w2252:sgl)
                n1289 = local read "MeasVelScrnSet2"() -> (w2251:sgl)
                n1290 = Add(x=w2252, y=w2251) -> (x+y=w2255:sgl)
                n1291 = Divide(x=w2255, y=sgl 2.0) -> (x/y=w2254:sgl)
              }
              frame "Screens" {
                # "This section checks to see if the counters have been fired.  If they have then the counter times are read"
                n1292 = To Single Precision Float(number=w2273) -> (single precision float=w2272:sgl[])
                n1293 = Index Array(array=w2272) -> (element #1=w2266:sgl, element #2=w2265:sgl)  [unwired: 2 in]
                n1294 = Equal To 0?(x=w2266) -> (x = 0?=w2264:bool)
                n1295 = Equal To 0?(x=w2265) -> (x = 0?=w2260:bool)
                n1296 = local read "Set#1 Separation"() -> (w2271:sgl)
                n1297 = local read "Set#2 Separation"() -> (w2268:sgl)
                n1298 = Divide(x=w2271, y=w2266) -> (x/y=w2262:sgl)
                n1299 = Divide(x=w2268, y=w2265) -> (x/y=w2259:sgl)
                n1300 = Select(t=sgl 0.0, s=w2264, f=w2262) -> (s? t:f=w2258:sgl)
                n1301 = Select(t=sgl 0.0, s=w2260, f=w2259) -> (s? t:f=w2257:sgl)
                n1302 = Add(x=w2258, y=w2257) -> (x+y=w2269:sgl)
                n1303 = Divide(x=w2269, y=sgl 2.0) -> (x/y=w2275:sgl)
                n1304 = case shown="No Error" w2267 {
                  selector: w2267 -> [w2278 _]
                  frame No Error {
                    # "=false"
                    n1305 = Unbundle By Name(w2278) -> ("status"=w2277:bool)
                    n1306 = Not(x=w2277) -> (.not. x?=w2276:bool)
                    n1307 = local write "readyClock"(w2276) -> ()
                  }
                  frame Error {
                  }
                }
                n1308 = call <vilib>:"Simple Error Handler.vi"("error in (no error)"=w2267) -> ("error out"=w2274:errorcluster)  [unwired: 1 in, 7 out]
              }
            }
            "Current/avg/speed" <- w2224
            n1309 = local write "MeasVelScrnSet1"(w2223) -> ()
            n1310 = local write "MeasVelScrnSet2"(w2222) -> ()
          }
          frame True {
            # "timeout expired"
          }
        }
      }
    }
    "SMErr" <- w535
    "progState" <- w534
    n1311 = disable-structure shown="Disabled" {
      disable-tunnel: w535 -> [w544 _]
      disable-tunnel: w534 -> [w543 _]
      frame Disabled {
        n1312 = flat-sequence {
          tunnel: w543 -> [_]
          tunnel: w544 -> [_]
          frame #0 {
            n1313 = Wait (ms)(milliseconds to wait=u32 1) -> ()  [unwired: 1 out]
          }
          frame #1 {
            n1314 = property on="progState" class="Enum (strict)"() -> ("RingText.Text"=w549:string)  [unwired: 2 in, 2 out]
            n1315 = Get Date/Time In Seconds() -> (seconds since 1Jan1904=w547:timestamp)
            n1316 = Format Date/Time String(seconds (now)=w547) -> (date/time string=w546:string)  [unwired: 2 out]
            n1317 = Build Array(w546, "," ("element"), w549) -> (w550:string[])
            n1318 = call-poly <vilib>:"Write To Spreadsheet File.vi"("append to file? (new file:F)"=TRUE, "1D data"=w550, "file path (dialog if empty)"=path "C:/state.txt") -> ()  [unwired: 5 in, 1 out]
          }
        }
      }
      frame Enabled {
      }
    }
    n1319 = Wait (ms)(milliseconds to wait=u32 50 ("millisecond timer value")) -> ()  [unwired: 1 out]
  }
  n1320 = while "Arming Loop" {
    tunnel: w3 -> [w2306]
    shift-right: [w2304] -> w20
    shift-left: w21 -> [w2305]
    shift-right: [w2298] -> w11
    shift-left: w1 -> [w2302]
    shift-right: [w2299] -> w12
    shift-left: w2 -> [w2303]
    shift-right: [w2293] -> w13
    shift-left: w10 -> [w2301]
    shift-right: [w2292] -> w14
    shift-left: w9 -> [w2300]
    stop <- "close arming loop" stop-if-true
    w2296 = 10.0  # timeout
    # "error code -200474\ntimeout expired"
    n1321 = call-poly <vilib>:"DAQmx Read.vi"("task/channels in"=w2302, "timeout"=w2296, "error in"=w2300) -> ("task out"=w2298:refnum<k21>, "data"=w2294:dbl, "error out"=w2289:errorcluster)  [unwired: 10 in]
    n1322 = call-poly <vilib>:"DAQmx Read.vi"("task/channels in"=w2303, "timeout"=w2296, "error in"=w2301) -> ("task out"=w2299:refnum<k21>, "data"=w2295:dbl, "error out"=w2287:errorcluster)  [unwired: 10 in]
    n1323 = Unbundle By Name(w2287) -> ("code"=w2284:i32)
    n1324 = Unbundle By Name(w2289) -> ("code"=w2288:i32)
    n1325 = Equal?(x=w2284, y=-200474) -> (x = y?=w2283:bool)
    n1326 = Equal?(x=w2288, y=-200474) -> (x = y?=w2291:bool)
    n1327 = Or(x=w2283, y=w2291) -> (x .or. y?=w2286:bool)
    n1328 = case shown="False" w2286 {
      tunnel: w2306 -> [w2315 _]
      tunnel: w2305 -> [w2314 w2320]
      tunnel: [w2313 w2320] -> w2304
      tunnel: w2295 -> [w2311 _]
      tunnel: w2294 -> [w2310 _]
      frame False {
        n1329 = Build Array(w2311, w2310) -> (w2312:dbl[])
        n1330 = Enqueue Element(queue=w2315, element=w2312, error in (no error)=w2314) -> (queue out=w2308:refnum<queue>, error out=w2313:errorcluster)  [unwired: 1 in, 1 out]
        n1331 = for {
          N: 10 -> [w2318]
          tunnel: w2308 -> [_]
          i -> [w2317]
          n1332 = Subtract(x=w2318, y=w2317) -> (x-y=→"cntDn":i32)
          n1333 = Wait (ms)(milliseconds to wait=u32 1000) -> ()  [unwired: 1 out]
        }
        "ARMED" <- FALSE ("ARMED")
      }
      frame True {
      }
    }
    n1334 = local write "ARMED"(TRUE ("ARMED")) -> ()
    n1335 = case shown="No Error" w2287 {
      selector: w2287 -> [w2324 w2326]
      tunnel: [w2324 errorcluster {"status"=FALSE, "code"=0, "source"=""} ("error IO")] -> w2293
      frame No Error {
      }
      frame Error {
        "errCtr0" <- w2326
      }
    }
    n1336 = case shown="No Error" w2289 {
      selector: w2289 -> [w2321 w2323]
      tunnel: [w2321 errorcluster {"status"=FALSE, "code"=0, "source"=""} ("error IO")] -> w2292
      frame No Error {
      }
      frame Error {
        "errCtr1" <- w2323
      }
    }
  }
  n1337 = call <vilib>:"DAQmx Clear Task.vi"("task in"=w11, "error in"=w14) -> ("error out"=w17:errorcluster)  [unwired: 13 in]
  n1338 = call <vilib>:"DAQmx Clear Task.vi"("task in"=w12, "error in"=w13) -> ("error out"=w18:errorcluster)  [unwired: 13 in]
  n1339 = Release Queue(queue=w3, force destroy? (F)=TRUE, error in (no error)=w20) -> (error out=w15:errorcluster)  [unwired: 2 out]
  n1340 = Merge Errors(w18, w17, w15) -> (w19:errorcluster)
  n1341 = call <vilib>:"General Error Handler.vi"("type of dialog (OK msg:1)"=w16, "error in (no error)"=w19) -> ()  [unwired: 9 in, 5 out]
